vi "Beampointing_BELLA_HTT.vi"() -> ()   [LabVIEW 2020]
uses:
  Shared/GUI_Template/GUI_master/tcp_new_data_event.ctl
  Shared/GUI_Template/GUI_master/tcp new data cluster.ctl
  Ctrs/beam detection.ctl
  GUI_Beampointing_single_TRA/Ctrs/move.ctl
  General GUIs/Device GUIs/GUI_Cameras/Controls/Crosshair type def.ctl
  <vilib>/Utility/file.llb/Read From Spreadsheet File (string).vi
  <userlib>/_OpenG.lib/array/array.llb/Filter 1D Array with Scalar (String)__ogtk.vi
  <vilib>/Utility/file.llb/Write To Spreadsheet File (string).vi
  <vilib>/Analysis/NI_AALBase.lvlib
  <vilib>/vision/NI_Vision_Development_Module.lvlib
panel:
  out "error out 3":errorcluster
  out "error out":errorcluster
  in  "Position.Axis 1::100":dbl caption="Motor Axis 1" min=-3.0 max=13.0 format="%#_6f"
  in  "Position.Axis 2::100":dbl caption="Motor Axis 1" min=-3.0 max=17.0 format="%#_6f"
  in  "GUIdevice 100":string
  out "Array 3":sgl[](array[numeric])=[35.01637, 16.987305, 27.281555, 56.5656, 0.0, 12.310791, 0.0, 0.0, 0.0, 0.0, 0.0, 0.0]
  in  "save path":path=path "W:/BP_DATA"
  out "size(s) 6":i32=12
  out "config path":string
  out "motor refs 7":refnum<vi>[](array[refnum])
  out "Moving Y":string
  out "Moving X":string
  out "particles":T1(array[cluster])=[{"Area"=13625.0, "Number of Holes"=0.0, "Bounding Rect"={"Left"=100.0, "Top"=93.0, "Right"=241.0, "Bottom"=225.0}, "Center of Mass"={"X"=171.3850275229358, "Y"=158.37277064220183}, "Orientation"=31.450434142859965, "Dimensions"={"Width"=141.0, "Height"=132.0}}]
  out "motor refs 6":refnum<vi>[](array[refnum])
  out "millisecond timer value":u32=150056294
  out "motor refs 5":refnum<vi>[](array[refnum])
  out "appended path":path=path "C:/Users/loasis.BELLANET/Documents/000 Labview/Developers Version/Interface/GUI_Beampointing_multi/defaultDevices_PICObooster.txt"
  out "motor refs 4":refnum<vi>[](array[refnum])
  in  "active Axis ref 3":cluster{"Ref X":refnum<vi>, "Ref Y":refnum<vi>}
  out "motor refs 3":refnum<vi>[](array[refnum])
  in  "active man refs":cluster{"Ref X":refnum<vi>, "Ref Y":refnum<vi>}
  out "motor refs 2":refnum<vi>[](array[refnum])
  in  "Numeric":dbl=2.0
  out "Current State":string="Exit"
  in  "output cluster 2":T5 {"detection para"."smal para"."Measurement Parameter" items=["Center of Mass X", "Center of Mass Y", "First Pixel X", "First Pixel Y", "Bounding Rect Left", "Bounding Rect Top", "Bounding Rect Right", "Bounding Rect Bottom", "Max Feret Diameter Start X", "Max Feret Diameter Start Y", "Max Feret Diameter End X", "Max Feret Diameter End Y", "Max Horiz. Segment Length Left", "Max Horiz. Segment Length Right", "Max Horiz. Segment Length Row", "-", "Bounding Rect Width", "Bounding Rect Height", "Bounding Rect Diagonal", "Perimeter", "Convex Hull Perimeter", "Holes' Perimeter", "Max Feret Diameter", "Equivalent Ellipse Major Axis", "Equivalent Ellipse Minor Axis", "Equivalent Ellipse Minor Axis (Feret)", "Equivalent Rect Long Side", "Equivalent Rect Short Side", "Equivalent Rect Diagonal", "Equivalent Rect Short Side (Feret)", "Average Horiz. Segment Length", "Average Vert. Segment Length", "Hydraulic Radius", "Waddel Disk Diameter", "-", "Area", "Holes' Area", "Particle & Holes' Area", "Convex Hull Area", "Image Area", "-", "Number of Holes", "Number of Horiz. Segments", "Number of Vert. Segments", "-", "Orientation", "Max Feret Diameter Orientation", "-", "% Area/Image Area", "% Area/(Particle & Holes' Area)", "Ratio of Equivalent Ellipse Axes", "Ratio of Equivalent Rect Sides", "-", "Elongation Factor", "Compactness Factor", "Heywood Circularity Factor", "Type Factor", "-", "Sum X", "Sum Y", "Sum XX", "Sum XY", "Sum YY", "Sum XXX", "Sum XXY", "Sum XYY", "Sum YYY", "-", "Moment of Inertia XX", "Moment of Inertia XY", "Moment of Inertia YY", "Moment of Inertia XXX", "Moment of Inertia XXY", "Moment of Inertia XYY", "Moment of Inertia YYY", "Norm. Moment of Inertia XX", "Norm. Moment of Inertia XY", "Norm. Moment of Inertia YY", "Norm. Moment of Inertia XXX", "Norm. Moment of Inertia XXY", "Norm. Moment of Inertia XYY", "Norm. Moment of Inertia YYY", "Hu Moment 1", "Hu Moment 2", "Hu Moment 3", "Hu Moment 4", "Hu Moment 5", "Hu Moment 6", "Hu Moment 7"]; "detection para"."smal para"."Range Lower Value" format="%.2f"; "detection para"."smal para"."Range Upper Value" format="%.2f"; "detection para"."detection method" items=["clustering", "entropy", "metric", "moments", "inter-class variance"]; "detection para"."Filter" items=["No Filter", "Median Filter", "Low Pass Filter"]}
  out "CCDs":string[](array[string])=["RegenCam", "BoosterCam", "PreampCam", "Amp1Cam", "Amp2Cam", "Amp3Cam", "", "", "", "", "", ""]
  in  "GUIdevice 12":string
  in  "GUIdevice 11":string
  in  "GUIdevice 10":string
  in  "GUIdevice 9":string
  out "error out 2":errorcluster
  in  "active cams":string[](array[string])
  in  "Motor Y":dbl[][](array[numeric])
  in  "Motor X":dbl[][](array[numeric])
  out "Names":string[](array[string])=["device12", "device45", "", ""]
  in  "Offset X stats":dbl[][](array[numeric])
  in  "Offset Y stats":dbl[][](array[numeric])
  out "Box":T6(array[cluster])=[{"Left"=100.0, "Top"=93.0, "Right"=241.0, "Bottom"=225.0}, {"Left"=87.0, "Top"=22.0, "Right"=220.0, "Bottom"=185.0}, {"Left"=80.0, "Top"=37.0, "Right"=220.0, "Bottom"=176.0}, {"Left"=78.0, "Top"=52.0, "Right"=221.0, "Bottom"=209.0}, {"Left"=0.0, "Top"=0.0, "Right"=0.0, "Bottom"=0.0}]
  in  "Tab Control 2":enum32{"Config ", "Main", "History"}(tab)=enum."Main"
  in  "associated motors":T7={"Motor CCD 1"=0, "Motor CCD 2"=0, "Motor CCD 3"=1, "Motor CCD 4"=0, "Motor CCD 5"=0, "Motor CCD 6"=0, "Motor CCD 7"=0, "Motor CCD 8"=0, "Motor CCD 9"=0, "Motor CCD 10"=0, "Motor CCD 11"=0, "Motor CCD 12"=0} {"Motor CCD 12" items=["device12", "device34", "HeatESP", ""]; "Motor CCD 11" items=["device12", "device34", "HeatESP", ""]; "Motor CCD 10" items=["device12", "device34", "HeatESP", ""]; "Motor CCD 9" items=["device12", "device34", "HeatESP", ""]; "Motor CCD 8" items=["device12", "device34", "HeatESP", ""]; "Motor CCD 7" items=["device12", "device34", "HeatESP", ""]; "Motor CCD 6" items=["device12", "device34", "HeatESP", ""]; "Motor CCD 5" items=["device12", "device34", "HeatESP", ""]; "Motor CCD 4" items=["device12", "device34", "HeatESP", ""]; "Motor CCD 3" items=["device12", "device34", "HeatESP", ""]; "Motor CCD 2" items=["device12", "device34", "HeatESP", ""]; "Motor CCD 1" items=["device12", "device34", "HeatESP", ""]}
  out "Cameras":T8={"[0]"="RegenCam", "[1]"="BoosterCam", "[2]"="PreampCam", "[3]"="Amp1Cam", "[4]"="Amp2Cam", "[5]"="Amp3Cam", "[6]"="", "[7]"="", "[8]"="", "[8] 2"="", "[8] 3"="", "[8] 4"=""}
  out "Status":cluster{i32, i32, "Centroid X":dbl[][]}(graph)={0, 1, "Centroid X"=[[171.87383691112902, 0.0, 0.0], [153.80799798158193, 0.0, 0.0], [147.97157969527117, 0.0, 0.0], [147.97285865350722, 0.0, 0.0], [0.0, 0.0, 0.0], [0.0, 0.0, 0.0], [0.0, 0.0, 0.0], [0.0, 0.0, 0.0], [0.0, 0.0, 0.0], [0.0, 0.0, 0.0], [0.0, 0.0, 0.0], [0.0, 0.0, 0.0]]}
  in  "Exposure:12":dbl=0.095 min=0.0001 max=1.0 format="%#_6f"
  in  "Triggerdelay::12":dbl=0.003 min=0.0 max=0.09 format="%#_6f"
  in  "Exposure::11":dbl=0.095 min=0.0001 max=1.0 format="%#_6f"
  in  "Triggerdelay::11":dbl=0.003 min=0.0 max=0.09 format="%#_6f"
  in  "Exposure::10":dbl=0.095 min=0.0001 max=1.0 format="%#_6f"
  in  "Triggerdelay::10":dbl=0.003 min=0.0 max=0.09 format="%#_6f"
  in  "Exposure::9":dbl=0.095 min=0.0001 max=1.0 format="%#_6f"
  in  "Triggerdelay::9":dbl=0.003 min=0.0 max=0.09 format="%#_6f"
  in  "Trigger::9":bool
  in  "Trigger::10":bool caption="Trigger:10"
  in  "Trigger::11":bool
  in  "Trigger::12":bool
  in  "Target.Y::9":dbl=45.0 caption="T9y" min=0.0 max=2000.0 format="%#_6f"
  in  "Target.X::9":dbl=47.0 caption="Tx9" min=0.0 max=2000.0 format="%#_6f"
  in  "Target.Y::10":dbl=45.0 caption="T10y" min=0.0 max=2000.0 format="%#_6f"
  in  "Target.X::10":dbl=47.0 caption="T10x" min=0.0 max=2000.0 format="%#_6f"
  in  "Target.Y::11":dbl=45.0 caption="T11y" min=0.0 max=2000.0 format="%#_6f"
  in  "Target.X::11":dbl=47.0 caption="T11x" min=0.0 max=2000.0 format="%#_6f"
  in  "Target.Y::12":dbl=45.0 caption="T12y" min=0.0 max=2000.0 format="%#_6f"
  in  "Target.X::12":dbl=47.0 caption="T12x" min=0.0 max=2000.0 format="%#_6f"
  in  "Exposure::8":dbl=0.095 min=0.0001 max=1.0 format="%#_6f"
  in  "Triggerdelay::8":dbl=0.003 min=0.0 max=0.09 format="%#_6f"
  in  "Trigger::8":bool
  in  "Target.Y::8":dbl=45.0 caption="T8y" min=0.0 max=2000.0 format="%#_6f"
  in  "Target.X::8":dbl=47.0 caption="T8x" min=0.0 max=2000.0 format="%#_6f"
  in  "Target.Y::7":dbl=45.0 caption="T7x" min=0.0 max=2000.0 format="%#_6f"
  in  "Target.X::7":dbl=47.0 caption="T7y" min=0.0 max=2000.0 format="%#_6f"
  in  "Target.Y::6":dbl=142.0 caption="T6y" min=0.0 max=5000.0 format="%#_6f"
  in  "Target.X::6":dbl=123.0 caption="T6x" min=0.0 max=5000.0 format="%#_6f"
  in  "Target.Y::5":dbl=108.0 caption="T5y" min=0.0 max=2000.0 format="%#_6f"
  in  "Target.X::5":dbl=172.0 caption="T5x" min=0.0 max=2000.0 format="%#_6f"
  in  "Target.Y::4":dbl=130.0 caption="T4y" min=0.0 max=2000.0 format="%#_6f"
  in  "Target.X::4":dbl=148.0 caption="T4x" min=0.0 max=2000.0 format="%#_6f"
  in  "Target.Y::3":dbl=110.0 caption="T3y" min=0.0 max=2000.0 format="%#_6f"
  in  "Target.X::3":dbl=154.0 caption="T3x" min=0.0 max=2000.0 format="%#_6f"
  in  "Target.Y::2":dbl=106.0 caption="T2y" min=0.0 max=2000.0 format="%#_6f"
  in  "Target.X::2":dbl=163.0 caption="T2x" min=0.0 max=2000.0 format="%#_6f"
  in  "Target.Y::1":dbl=162.0 caption="T1y" min=0.0 max=2000.0 format="%#_6f"
  in  "Target.X::1":dbl=171.0 caption="T1x" min=0.0 max=2000.0 format="%#_6f"
  in  "Exposure::7":dbl=0.095 min=3.8e-05 max=1.0 format="%#_6f"
  in  "Triggerdelay::7":dbl=0.003 min=0.0 max=0.09 format="%#_6f"
  in  "Trigger::7":bool
  in  "Exposure::6":dbl=0.095 min=3.8e-05 max=1.0 format="%#_6f"
  in  "Triggerdelay::6":dbl=0.003 min=0.0 max=0.09 format="%#_6f"
  in  "Trigger::6":bool
  in  "Exposure::5":dbl=0.095 min=3.8e-05 max=1.0 format="%#_6f"
  in  "Triggerdelay::5":dbl=0.003 min=0.0 max=0.09 format="%#_6f"
  in  "Trigger::5":bool
  in  "Exposure::4":dbl=0.095 min=3.8e-05 max=1.0 format="%#_6f"
  in  "Triggerdelay::4":dbl=0.003 min=0.0 max=0.09 format="%#_6f"
  in  "Trigger::4":bool
  in  "Exposure::3":dbl=0.095 min=3.8e-05 max=1.0 format="%#_6f"
  in  "Triggerdelay::3":dbl=0.003 min=0.0 max=0.09 format="%#_6f"
  in  "Trigger::3":bool
  in  "Exposure::2":dbl=0.095 min=0.0 max=1.0 format="%#_6f"
  in  "Triggerdelay::2":dbl=0.003 min=0.0 max=1.0 format="%#_6f"
  in  "Trigger::2":bool
  out "image::1":T9(plugin-control) caption="BellaCam32_3"
  out "image::2":T9(plugin-control) caption="BellaCam46_2_Scatter_In_1"
  out "image::3":T9(plugin-control)
  out "image::4":T9(plugin-control)
  out "image::5":T9(plugin-control)
  out "image::6":T9(plugin-control)
  out "image::7":T9(plugin-control)
  out "image::8":T9(plugin-control)
  in  "Exposure::1":dbl=0.095 min=0.0001 max=1000001.0 format="%#_6f"
  in  "Triggerdelay::1":dbl=0.003 min=0.0 max=100000.0 format="%#_6f"
  in  "Trigger::1":bool
  in  "UDP error message":string
  out "required Y":bool[](array[boolean])=[FALSE, TRUE, FALSE, FALSE, FALSE]
  out "required X":bool[](array[boolean])=[FALSE, TRUE, FALSE, FALSE, FALSE]
  out "detected":bool[](array[boolean])=[TRUE, TRUE, TRUE, TRUE, FALSE]
  out "name array":string[](array[string])=["RegenCam", "BoosterCam", "PreampCam", "Amp1Cam", "Amp3Cam"]
  out "image::9":T9(plugin-control)
  out "image::10":T9(plugin-control)
  out "image::11":T9(plugin-control)
  out "image::12":T9(plugin-control)
  out "speedmode X":bool[](array[boolean])=[TRUE, TRUE, TRUE, TRUE, FALSE]
  out "speedmode Y":bool[](array[boolean])=[TRUE, FALSE, TRUE, TRUE, FALSE]
  out "CCD 9":cluster{timestamp[], dbl[]}[](graph)=[{[timestamp(3549547983.3591223 s since 1904-01-01)], [0.0]}, {[timestamp(3549547983.3591223 s since 1904-01-01)], [0.0]}, {[timestamp(3549547983.3591223 s since 1904-01-01)], [20.0]}, {[timestamp(3549547983.3591223 s since 1904-01-01)], [-20.0, -20.0, -20.0, -20.0]}]
  out "CCD 10":cluster{timestamp[], dbl[]}[](graph)=[{[timestamp(3549547983.360123 s since 1904-01-01)], [0.0]}, {[timestamp(3549547983.360123 s since 1904-01-01)], [0.0]}, {[timestamp(3549547983.360123 s since 1904-01-01)], [20.0]}, {[timestamp(3549547983.360123 s since 1904-01-01)], [-20.0, -20.0, -20.0, -20.0]}]
  out "CCD 11":cluster{timestamp[], dbl[]}[](graph)=[{[timestamp(3549547983.360123 s since 1904-01-01)], [0.0]}, {[timestamp(3549547983.360123 s since 1904-01-01)], [0.0]}, {[timestamp(3549547983.360123 s since 1904-01-01)], [20.0]}, {[timestamp(3549547983.360123 s since 1904-01-01)], [-20.0, -20.0, -20.0, -20.0]}]
  out "CCD 12":cluster{timestamp[], dbl[]}[](graph)=[{[timestamp(3549547983.360123 s since 1904-01-01)], [0.0]}, {[timestamp(3549547983.360123 s since 1904-01-01)], [0.0]}, {[timestamp(3549547983.360123 s since 1904-01-01)], [20.0]}, {[timestamp(3549547983.360123 s since 1904-01-01)], [-20.0, -20.0, -20.0, -20.0]}]
  out "CCD 5":cluster{timestamp[], dbl[]}[](graph)=[{[timestamp(3549547983.358122 s since 1904-01-01)], [0.0]}, {[timestamp(3549547983.358122 s since 1904-01-01)], [0.0]}, {[timestamp(3549547983.358122 s since 1904-01-01)], [20.0]}, {[timestamp(3549547983.358122 s since 1904-01-01)], [-20.0, -20.0, -20.0, -20.0]}]
  out "CCD 6":cluster{timestamp[], dbl[]}[](graph)=[{[timestamp(3549547983.3591223 s since 1904-01-01)], [0.0]}, {[timestamp(3549547983.3591223 s since 1904-01-01)], [0.0]}, {[timestamp(3549547983.3591223 s since 1904-01-01)], [20.0]}, {[timestamp(3549547983.3591223 s since 1904-01-01)], [-20.0, -20.0, -20.0, -20.0]}]
  out "CCD 7":cluster{timestamp[], dbl[]}[](graph)=[{[timestamp(3549547983.3591223 s since 1904-01-01)], [0.0]}, {[timestamp(3549547983.3591223 s since 1904-01-01)], [0.0]}, {[timestamp(3549547983.3591223 s since 1904-01-01)], [20.0]}, {[timestamp(3549547983.3591223 s since 1904-01-01)], [-20.0, -20.0, -20.0, -20.0]}]
  out "CCD 8":cluster{timestamp[], dbl[]}[](graph)=[{[timestamp(3549547983.3591223 s since 1904-01-01)], [0.0]}, {[timestamp(3549547983.3591223 s since 1904-01-01)], [0.0]}, {[timestamp(3549547983.3591223 s since 1904-01-01)], [20.0]}, {[timestamp(3549547983.3591223 s since 1904-01-01)], [-20.0, -20.0, -20.0, -20.0]}]
  out "CCD 2":cluster{timestamp[], dbl[]}[](graph)=[{[timestamp(3549547983.358122 s since 1904-01-01)], [3.0783937413765585]}, {[timestamp(3549547983.358122 s since 1904-01-01)], [8.883046862591215]}, {[timestamp(3549547983.358122 s since 1904-01-01)], [20.0]}, {[timestamp(3549547983.358122 s since 1904-01-01)], [-20.0, -20.0, -20.0, -20.0]}]
  out "CCD 1":cluster{timestamp[], dbl[]}[](graph)=[{[timestamp(3549547983.357121 s since 1904-01-01)], [3.1654865062995725]}, {[timestamp(3549547983.357121 s since 1904-01-01)], [-0.42630614615123363]}, {[timestamp(3549547983.357121 s since 1904-01-01)], [20.0]}, {[timestamp(3549547983.357121 s since 1904-01-01)], [-20.0, -20.0, -20.0, -20.0]}]
  out "CCD 3":cluster{timestamp[], dbl[]}[](graph)=[{[timestamp(3549547983.358122 s since 1904-01-01)], [5.607599326451648]}, {[timestamp(3549547983.358122 s since 1904-01-01)], [4.73033759911138]}, {[timestamp(3549547983.358122 s since 1904-01-01)], [0.0]}, {[timestamp(3549547983.358122 s since 1904-01-01)], [0.0, 0.0, 0.0, 0.0]}]
  out "CCD 4":cluster{timestamp[], dbl[]}[](graph)=[{[timestamp(3549547983.358122 s since 1904-01-01)], [1.2734976836249814]}, {[timestamp(3549547983.358122 s since 1904-01-01)], [-0.6350086940318818]}, {[timestamp(3549547983.358122 s since 1904-01-01)], [20.0]}, {[timestamp(3549547983.358122 s since 1904-01-01)], [-20.0, -20.0, -20.0, -20.0]}]
  in  "History Size":i32=2000
  out "History Index":i32=1
  in  "Feedback Global":bool
  in  "detection para":T3[](array[typedef])=[{"Filter"=1, "Filter Para"={"X Size"=5, "Y Size"=5, "% Tolerance"=1}, "detection method"=4, "smal para"=[{"Measurement Parameter"=35, "Range Lower Value"=0.0, "Range Upper Value"=0.0, "Range"=TRUE, "Measurement Type"=FALSE}], "Remove small Objects"=TRUE, "Restrict to round Objects"=FALSE}, {"Filter"=1, "Filter Para"={"X Size"=5, "Y Size"=5, "% Tolerance"=1}, "detection method"=4, "smal para"=[{"Measurement Parameter"=35, "Range Lower Value"=0.0, "Range Upper Value"=500.0, "Range"=FALSE, "Measurement Type"=FALSE}], "Remove small Objects"=TRUE, "Restrict to round Objects"=FALSE}, {"Filter"=1, "Filter Para"={"X Size"=5, "Y Size"=5, "% Tolerance"=1}, "detection method"=4, "smal para"=[{"Measurement Parameter"=35, "Range Lower Value"=0.0, "Range Upper Value"=500.0, "Range"=TRUE, "Measurement Type"=FALSE}], "Remove small Objects"=TRUE, "Restrict to round Objects"=FALSE}, {"Filter"=1, "Filter Para"={"X Size"=5, "Y Size"=5, "% Tolerance"=1}, "detection method"=4, "smal para"=[{"Measurement Parameter"=35, "Range Lower Value"=0.0, "Range Upper Value"=500.0, "Range"=TRUE, "Measurement Type"=FALSE}], "Remove small Objects"=TRUE, "Restrict to round Objects"=FALSE}, {"Filter"=1, "Filter Para"={"X Size"=5, "Y Size"=5, "% Tolerance"=1}, "detection method"=4, "smal para"=[{"Measurement Parameter"=35, "Range Lower Value"=0.0, "Range Upper Value"=500.0, "Range"=TRUE, "Measurement Type"=FALSE}], "Remove small Objects"=TRUE, "Restrict to round Objects"=FALSE}, {"Filter"=1, "Filter Para"={"X Size"=5, "Y Size"=5, "% Tolerance"=1}, "detection method"=4, "smal para"=[{"Measurement Parameter"=35, "Range Lower Value"=0.0, "Range Upper Value"=500.0, "Range"=TRUE, "Measurement Type"=FALSE}], "Remove small Objects"=TRUE, "Restrict to round Objects"=FALSE}, {"Filter"=1, "Filter Para"={"X Size"=5, "Y Size"=5, "% Tolerance"=1}, "detection method"=4, "smal para"=[{"Measurement Parameter"=35, "Range Lower Value"=0.0, "Range Upper Value"=500.0, "Range"=TRUE, "Measurement Type"=FALSE}], "Remove small Objects"=TRUE, "Restrict to round Objects"=FALSE}, {"Filter"=1, "Filter Para"={"X Size"=5, "Y Size"=5, "% Tolerance"=1}, "detection method"=3, "smal para"=[{"Measurement Parameter"=35, "Range Lower Value"=0.0, "Range Upper Value"=0.0, "Range"=FALSE, "Measurement Type"=FALSE}], "Remove small Objects"=TRUE, "Restrict to round Objects"=FALSE}, {"Filter"=1, "Filter Para"={"X Size"=5, "Y Size"=5, "% Tolerance"=1}, "detection method"=4, "smal para"=[{"Measurement Parameter"=35, "Range Lower Value"=0.0, "Range Upper Value"=0.0, "Range"=FALSE, "Measurement Type"=FALSE}], "Remove small Objects"=TRUE, "Restrict to round Objects"=FALSE}, {"Filter"=1, "Filter Para"={"X Size"=5, "Y Size"=5, "% Tolerance"=1}, "detection method"=4, "smal para"=[{"Measurement Parameter"=35, "Range Lower Value"=0.0, "Range Upper Value"=500.0, "Range"=TRUE, "Measurement Type"=FALSE}], "Remove small Objects"=TRUE, "Restrict to round Objects"=FALSE}, {"Filter"=1, "Filter Para"={"X Size"=5, "Y Size"=5, "% Tolerance"=1}, "detection method"=4, "smal para"=[{"Measurement Parameter"=35, "Range Lower Value"=0.0, "Range Upper Value"=500.0, "Range"=TRUE, "Measurement Type"=FALSE}], "Remove small Objects"=TRUE, "Restrict to round Objects"=FALSE}, {"Filter"=1, "Filter Para"={"X Size"=5, "Y Size"=5, "% Tolerance"=1}, "detection method"=4, "smal para"=[{"Measurement Parameter"=35, "Range Lower Value"=0.0, "Range Upper Value"=500.0, "Range"=TRUE, "Measurement Type"=FALSE}], "Remove small Objects"=TRUE, "Restrict to round Objects"=FALSE}] {"smal para"."Measurement Parameter" items=["Center of Mass X", "Center of Mass Y", "First Pixel X", "First Pixel Y", "Bounding Rect Left", "Bounding Rect Top", "Bounding Rect Right", "Bounding Rect Bottom", "Max Feret Diameter Start X", "Max Feret Diameter Start Y", "Max Feret Diameter End X", "Max Feret Diameter End Y", "Max Horiz. Segment Length Left", "Max Horiz. Segment Length Right", "Max Horiz. Segment Length Row", "-", "Bounding Rect Width", "Bounding Rect Height", "Bounding Rect Diagonal", "Perimeter", "Convex Hull Perimeter", "Holes' Perimeter", "Max Feret Diameter", "Equivalent Ellipse Major Axis", "Equivalent Ellipse Minor Axis", "Equivalent Ellipse Minor Axis (Feret)", "Equivalent Rect Long Side", "Equivalent Rect Short Side", "Equivalent Rect Diagonal", "Equivalent Rect Short Side (Feret)", "Average Horiz. Segment Length", "Average Vert. Segment Length", "Hydraulic Radius", "Waddel Disk Diameter", "-", "Area", "Holes' Area", "Particle & Holes' Area", "Convex Hull Area", "Image Area", "-", "Number of Holes", "Number of Horiz. Segments", "Number of Vert. Segments", "-", "Orientation", "Max Feret Diameter Orientation", "-", "% Area/Image Area", "% Area/(Particle & Holes' Area)", "Ratio of Equivalent Ellipse Axes", "Ratio of Equivalent Rect Sides", "-", "Elongation Factor", "Compactness Factor", "Heywood Circularity Factor", "Type Factor", "-", "Sum X", "Sum Y", "Sum XX", "Sum XY", "Sum YY", "Sum XXX", "Sum XXY", "Sum XYY", "Sum YYY", "-", "Moment of Inertia XX", "Moment of Inertia XY", "Moment of Inertia YY", "Moment of Inertia XXX", "Moment of Inertia XXY", "Moment of Inertia XYY", "Moment of Inertia YYY", "Norm. Moment of Inertia XX", "Norm. Moment of Inertia XY", "Norm. Moment of Inertia YY", "Norm. Moment of Inertia XXX", "Norm. Moment of Inertia XXY", "Norm. Moment of Inertia XYY", "Norm. Moment of Inertia YYY", "Hu Moment 1", "Hu Moment 2", "Hu Moment 3", "Hu Moment 4", "Hu Moment 5", "Hu Moment 6", "Hu Moment 7"]; "smal para"."Range Lower Value" format="%.2f"; "smal para"."Range Upper Value" format="%.2f"; "detection method" items=["clustering", "entropy", "metric", "moments", "inter-class variance"]; "Filter" items=["No Filter", "Median Filter", "Low Pass Filter"]}
  in  "GUIdevice 8":string
  in  "Tab Control":T10(tab)
  in  "new tdms":bool
  in  "Save Stats":bool
  in  "Save Config":bool
  in  "Load Config":bool
  in  "update speed [ms]":i32=1000
  in  "img to avg":i32=6 min=3 max=200
  in  "Reset History":bool
  in  "autodetect":bool
  in  "Detection Rate":dbl=0.8 min=0.001 max=1.0
  in  "Center":bool
  in  "Align":bool
  in  "Speedmode @":dbl=5.0 min=1.0 max=20.0
  in  "device ini":bool
  in  "beam detection para":T3={"Filter"=1, "Filter Para"={"X Size"=5, "Y Size"=5, "% Tolerance"=1}, "detection method"=4, "smal para"=[{"Measurement Parameter"=35, "Range Lower Value"=0.0, "Range Upper Value"=500.0, "Range"=FALSE, "Measurement Type"=FALSE}], "Remove small Objects"=TRUE, "Restrict to round Objects"=FALSE} {"smal para"."Measurement Parameter" items=["Center of Mass X", "Center of Mass Y", "First Pixel X", "First Pixel Y", "Bounding Rect Left", "Bounding Rect Top", "Bounding Rect Right", "Bounding Rect Bottom", "Max Feret Diameter Start X", "Max Feret Diameter Start Y", "Max Feret Diameter End X", "Max Feret Diameter End Y", "Max Horiz. Segment Length Left", "Max Horiz. Segment Length Right", "Max Horiz. Segment Length Row", "-", "Bounding Rect Width", "Bounding Rect Height", "Bounding Rect Diagonal", "Perimeter", "Convex Hull Perimeter", "Holes' Perimeter", "Max Feret Diameter", "Equivalent Ellipse Major Axis", "Equivalent Ellipse Minor Axis", "Equivalent Ellipse Minor Axis (Feret)", "Equivalent Rect Long Side", "Equivalent Rect Short Side", "Equivalent Rect Diagonal", "Equivalent Rect Short Side (Feret)", "Average Horiz. Segment Length", "Average Vert. Segment Length", "Hydraulic Radius", "Waddel Disk Diameter", "-", "Area", "Holes' Area", "Particle & Holes' Area", "Convex Hull Area", "Image Area", "-", "Number of Holes", "Number of Horiz. Segments", "Number of Vert. Segments", "-", "Orientation", "Max Feret Diameter Orientation", "-", "% Area/Image Area", "% Area/(Particle & Holes' Area)", "Ratio of Equivalent Ellipse Axes", "Ratio of Equivalent Rect Sides", "-", "Elongation Factor", "Compactness Factor", "Heywood Circularity Factor", "Type Factor", "-", "Sum X", "Sum Y", "Sum XX", "Sum XY", "Sum YY", "Sum XXX", "Sum XXY", "Sum XYY", "Sum YYY", "-", "Moment of Inertia XX", "Moment of Inertia XY", "Moment of Inertia YY", "Moment of Inertia XXX", "Moment of Inertia XXY", "Moment of Inertia XYY", "Moment of Inertia YYY", "Norm. Moment of Inertia XX", "Norm. Moment of Inertia XY", "Norm. Moment of Inertia YY", "Norm. Moment of Inertia XXX", "Norm. Moment of Inertia XXY", "Norm. Moment of Inertia XYY", "Norm. Moment of Inertia YYY", "Hu Moment 1", "Hu Moment 2", "Hu Moment 3", "Hu Moment 4", "Hu Moment 5", "Hu Moment 6", "Hu Moment 7"]; "smal para"."Range Lower Value" format="%.2f"; "smal para"."Range Upper Value" format="%.2f"; "detection method" items=["clustering", "entropy", "metric", "moments", "inter-class variance"]; "Filter" items=["No Filter", "Median Filter", "Low Pass Filter"]}
  in  "move config":T2={"Tolerance [%]"=0.1, "Stepsize"=0.0001, "Invert Axis"=TRUE, "Invert Direction X"=FALSE, "Invert Direction Y"=TRUE, "enable feedback"=FALSE, "Set Centriod Target"=FALSE}
  in  "Position 2":dbl=-20.0 caption="Stepsize" min=0.0 max=999999.0 format="%_6f"
  in  "Position 1":dbl=20.0 caption="Stepsize" min=0.0 max=999999.0 format="%_6f"
  in  "Right":bool caption="RelativeMove.Axis 1.CCW::1"
  in  "Left":bool caption="RelativeMove.Axis 1.CW::1"
  in  "Down":bool caption="RelativeMove.Axis. 2.CCW::1"
  in  "Up":bool caption="RelativeMove.Axis 2.CW::1"
  in  "StepSize":dbl=5.0 caption="Stepsize" min=0.0 max=500.0 format="%#.4f"
  in  "active axis refs 2":T11(array[cluster])
  in  "active Axis ref":cluster{"Ref X":refnum<vi>, "Ref Y":refnum<vi>}
  in  "CCDs":u16(ring) items=["BellaCam32_3", "BellaCam46_2_Scatter_In_1", "", "", "", "", "", "", "", "", "", ""]
  out "motor refs":refnum<vi>[](array[refnum])
  in  "Position.Axis 3::99":dbl caption="Motor Axis 1" min=-5000.0 max=5000.0
  in  "Position.Axis 4::99":dbl caption="Motor Axis 1" min=-5000.0 max=5000.0
  in  "Position.Axis 2::99":dbl=-20.0 caption="Motor Axis 1" min=-5000.0 max=5000.0
  in  "Position.Axis 1::99":dbl=20.0 caption="Motor Axis 1" min=-5000.0 max=5000.0
  in  "GUIdevice 99":string="PicoPad_LCave"
  in  "move properties":T2[](array[typedef])=[{"Tolerance [%]"=0.1, "Stepsize"=0.0001, "Invert Axis"=TRUE, "Invert Direction X"=FALSE, "Invert Direction Y"=TRUE, "enable feedback"=FALSE, "Set Centriod Target"=FALSE}, {"Tolerance [%]"=0.1, "Stepsize"=0.0001, "Invert Axis"=TRUE, "Invert Direction X"=FALSE, "Invert Direction Y"=TRUE, "enable feedback"=FALSE, "Set Centriod Target"=FALSE}, {"Tolerance [%]"=0.1, "Stepsize"=0.0001, "Invert Axis"=TRUE, "Invert Direction X"=FALSE, "Invert Direction Y"=TRUE, "enable feedback"=FALSE, "Set Centriod Target"=FALSE}, {"Tolerance [%]"=0.1, "Stepsize"=0.0001, "Invert Axis"=TRUE, "Invert Direction X"=FALSE, "Invert Direction Y"=TRUE, "enable feedback"=FALSE, "Set Centriod Target"=FALSE}, {"Tolerance [%]"=0.1, "Stepsize"=0.0001, "Invert Axis"=TRUE, "Invert Direction X"=FALSE, "Invert Direction Y"=TRUE, "enable feedback"=FALSE, "Set Centriod Target"=FALSE}, {"Tolerance [%]"=0.1, "Stepsize"=0.0001, "Invert Axis"=TRUE, "Invert Direction X"=FALSE, "Invert Direction Y"=TRUE, "enable feedback"=FALSE, "Set Centriod Target"=FALSE}, {"Tolerance [%]"=0.1, "Stepsize"=0.0001, "Invert Axis"=TRUE, "Invert Direction X"=FALSE, "Invert Direction Y"=TRUE, "enable feedback"=FALSE, "Set Centriod Target"=FALSE}, {"Tolerance [%]"=0.1, "Stepsize"=0.0001, "Invert Axis"=TRUE, "Invert Direction X"=FALSE, "Invert Direction Y"=TRUE, "enable feedback"=FALSE, "Set Centriod Target"=FALSE}, {"Tolerance [%]"=0.1, "Stepsize"=0.0001, "Invert Axis"=TRUE, "Invert Direction X"=FALSE, "Invert Direction Y"=TRUE, "enable feedback"=FALSE, "Set Centriod Target"=FALSE}, {"Tolerance [%]"=0.1, "Stepsize"=0.0001, "Invert Axis"=TRUE, "Invert Direction X"=FALSE, "Invert Direction Y"=TRUE, "enable feedback"=FALSE, "Set Centriod Target"=FALSE}, {"Tolerance [%]"=0.1, "Stepsize"=0.0001, "Invert Axis"=TRUE, "Invert Direction X"=FALSE, "Invert Direction Y"=TRUE, "enable feedback"=FALSE, "Set Centriod Target"=FALSE}, {"Tolerance [%]"=0.1, "Stepsize"=0.0001, "Invert Axis"=TRUE, "Invert Direction X"=FALSE, "Invert Direction Y"=TRUE, "enable feedback"=FALSE, "Set Centriod Target"=FALSE}, {"Tolerance [%]"=0.1, "Stepsize"=0.0001, "Invert Axis"=TRUE, "Invert Direction X"=FALSE, "Invert Direction Y"=TRUE, "enable feedback"=FALSE, "Set Centriod Target"=FALSE}]
  in  "Time":timestamp[][](array[timestamp])
  in  "Mean Size":dbl[][](array[numeric])
  in  "Size":dbl[][](array[numeric])
  in  "active CCDs":i32(listbox)=-1
  in  "Offset Y":dbl[][](array[numeric])
  in  "Offset X":dbl[][](array[numeric])
  in  "Mean Centroid X":dbl[][](array[numeric])
  in  "Mean Centroid Y":dbl[][](array[numeric])
  in  "Centroid Y":dbl[][](array[numeric])
  in  "Centroid X":dbl[][](array[numeric])
  in  "GUIdevice 7":string
  in  "GUIdevice 6":string="Amp3Cam"
  in  "GUIdevice 5":string="Amp2Cam"
  in  "GUIdevice 4":string="Amp1Cam"
  in  "GUIdevice 3":string="PreampCam"
  in  "GUIdevice 2":string="BoosterCam"
  in  "insert tag":bool=TRUE
  in  "stop":bool
  in  "GUIdevice 1":string="RegenCam"
  out "tcp data event":T12
  out "error IO 2":errorcluster
  # "x [Tolerance]"
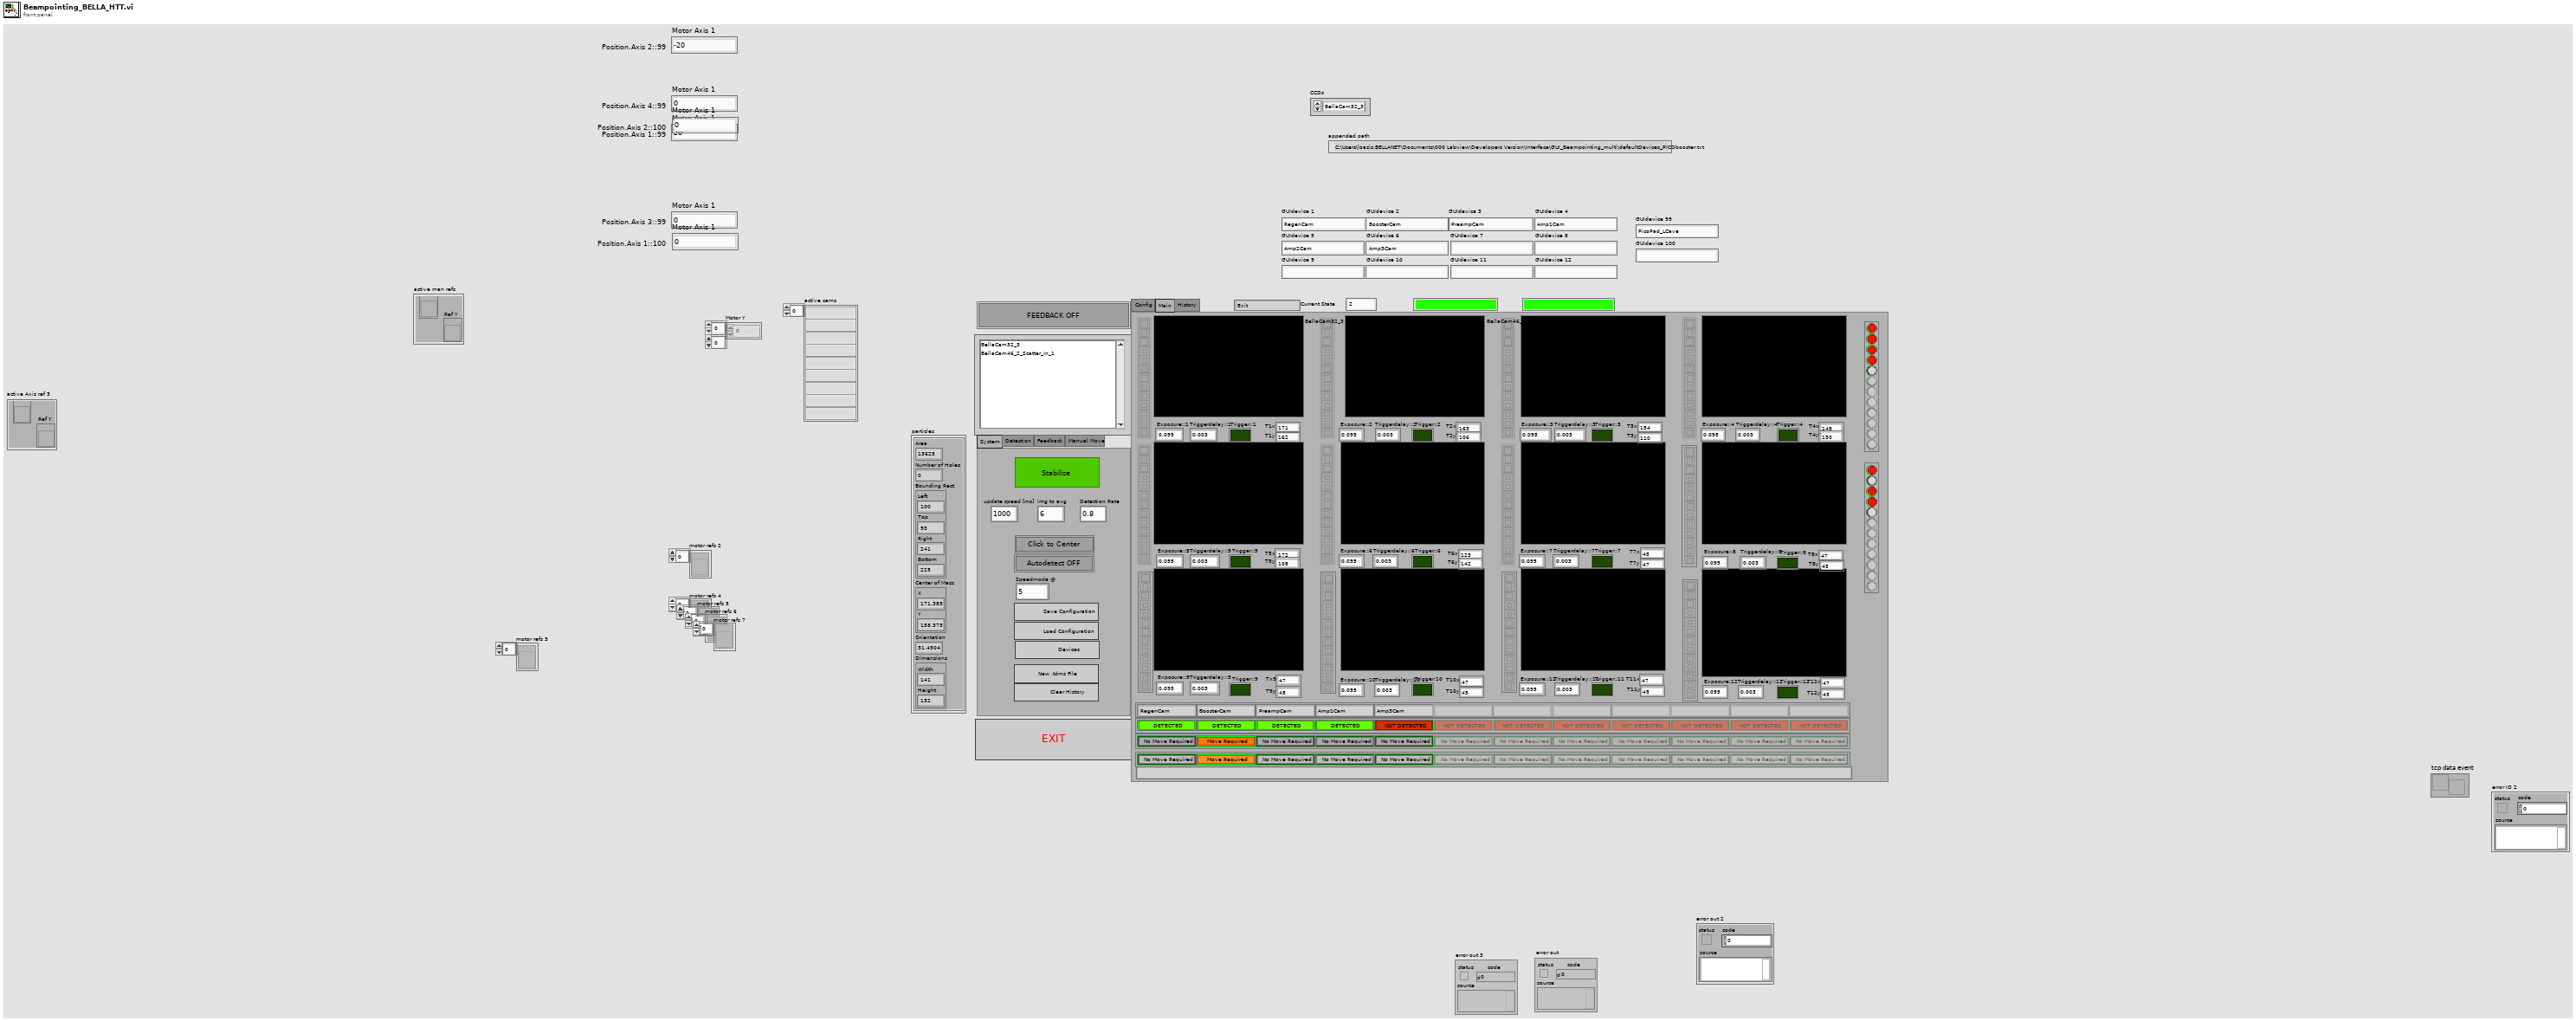
[diagram p1: front panel]
types:
  T1 = cluster{"Area":dbl, "Number of Holes":dbl, "Bounding Rect":cluster{"Left":dbl, "Top":dbl, "Right":dbl, "Bottom":dbl}, "Center of Mass":cluster{"X":dbl, "Y":dbl}, "Orientation":dbl, "Dimensions":cluster{"Width":dbl, "Height":dbl}}[]
  T2 = typedef "move.ctl" = cluster{"Tolerance [%]":dbl, "Stepsize":dbl, "Invert Axis":bool, "Invert Direction X":bool, "Invert Direction Y":bool, "enable feedback":bool, "Set Centriod Target":bool}
  T3 = typedef "beam detection.ctl" = cluster{"Filter":u16, "Filter Para":cluster{"X Size":i32, "Y Size":i32, "% Tolerance":i32}, "detection method":i32, "smal para":cluster{"Measurement Parameter":T4, "Range Lower Value":dbl, "Range Upper Value":dbl, "Range":bool, "Measurement Type":bool}[], "Remove small Objects":bool, "Restrict to round Objects":bool}
  T4 = typedef "Particle Parameters" = i32
  T5 = cluster{"CCDs":string[], "move properties":T2[], "detection para":T3[], "thresholds":cluster{"Lower value":sgl, "Upper value":sgl}[], "Value":cluster{"Motor CCD 1":u16, "Motor CCD 2":u16, "Motor CCD 3":u16, "Motor CCD 4":u16, "Motor CCD 5":u16, "Motor CCD 6":u16, "Motor CCD 7":u16, "Motor CCD 8":u16, "Motor CCD 9":u16, "Motor CCD 10":u16, "Motor CCD 11":u16, "Motor CCD 12":u16}}
  T6 = cluster{"Left":dbl, "Top":dbl, "Right":dbl, "Bottom":dbl}[]
  T7 = cluster{"Motor CCD 1":u16, "Motor CCD 2":u16, "Motor CCD 3":u16, "Motor CCD 4":u16, "Motor CCD 5":u16, "Motor CCD 6":u16, "Motor CCD 7":u16, "Motor CCD 8":u16, "Motor CCD 9":u16, "Motor CCD 10":u16, "Motor CCD 11":u16, "Motor CCD 12":u16}
  T8 = cluster{"[0]":string, "[1]":string, "[2]":string, "[3]":string, "[4]":string, "[5]":string, "[6]":string, "[7]":string, "[8]":string, "[8] 2":string, "[8] 3":string, "[8] 4":string}
  T9 = typedef "IMAQ Image.ctl" = refnum<image>
  T10 = enum32{"System", "Detection", "Feedback", "Manual Move"}
  T11 = cluster{"Ref X":refnum<vi>, "Ref Y":refnum<vi>}[]
  T12 = typedef "tcp_new_data_event.ctl" = refnum<user-event>
  T13 = typedef "tcp new data cluster.ctl" = cluster{"EventEnum":enum16{"new data", "connection status update"}, "Device name":string}
  T14 = typedef "Crosshair type def.ctl" = cluster{"Draw":bool, "Target":cluster{"x":dbl, "y":dbl}, "Size":cluster{"x":dbl, "y":dbl}, "Angle":dbl, "Color":u32, "Thickness":u8, "CrosshairLabel":string}
  T15 = cluster{"Left":i32, "Top":i32, "Right":i32, "Bottom":i32}
  T16 = enum32{"invalid app kind", "Development System", "Run Time System", "Student Edition", "Embedded LabVIEW", "Evaluation", "Custom"}
  T17 = enum16{"open", "open or create", "create or replace", "create", "open (read-only)"}
  T18 = enum32{"Invalid", "Standard", "Closed", "Hidden", "Minimized", "Maximized"}
  T19 = enum16{"open", "replace", "create", "open or create", "replace or create", "replace or create with confirmation"}
  T20 = enum8{"Enabled", "Disabled", "Disabled and Grayed Out"}
  T21 = typedef "Image Type" = u32
  T22 = cluster{"[0]":string, "[1]":string, "[2]":string, "[3]":string, "[4]":string, "[5]":string, "[6]":string, "[7]":string, "[8]":string, "[9]":string, "[10]":string, "[11]":string}
  T23 = cluster{"Target.X::1":refnum<vi>, "Target.Y::1":refnum<vi>}
  T24 = cluster{"Target.X::2":refnum<vi>, "Target.Y::2":refnum<vi>}
  T25 = cluster{"Target.X::3":refnum<vi>, "Target.Y::3":refnum<vi>}
  T26 = cluster{"Target.X::4":refnum<vi>, "Target.Y::4":refnum<vi>}
  T27 = cluster{"Target.X::5":refnum<vi>, "Target.Y::5":refnum<vi>}
  T28 = cluster{"Target.X::6":refnum<vi>, "Target.Y::6":refnum<vi>}
  T29 = cluster{"Target.X::7":refnum<vi>, "Target.Y::7":refnum<vi>}
  T30 = cluster{"Target.X::8":refnum<vi>, "Target.Y::8":refnum<vi>}
  T31 = cluster{"Target.X::12":refnum<vi>, "Target.Y::12":refnum<vi>}
  T32 = cluster{"Target.X::9":refnum<vi>, "Target.Y::9":refnum<vi>}
  T33 = cluster{"Target.X::10":refnum<vi>, "Target.Y::10":refnum<vi>}
  T34 = cluster{"Target.X::11":refnum<vi>, "Target.Y::11":refnum<vi>}
  T35 = cluster{"Target.X::12":refnum<vi>, "Target.Y::12":refnum<vi>}[]
  T36 = cluster{"Left":dbl, "Top":dbl, "Right":dbl, "Bottom":dbl}
  T37 = cluster{"Core":cluster{"Current VI Reference":refnum<vi>, "Close Panel on Exit?":bool}, "detection para":T3[], "thresholds":cluster{"Lower value":sgl, "Upper value":sgl}[], "Centroid X":dbl[][], "Centroid Y":dbl[][], "img to avg":i32, "Mean Centroid X":dbl[][], "Mean Centroid Y":dbl[][], "Offset X":dbl[][], "Offset Y":dbl[][], "Offset X stats ":dbl[][], "Offset Y stats ":dbl[][], "Size":dbl[][], "Mean Size":dbl[][], "Time":timestamp[][], "move properties":T2[], "active axis refs 2":cluster{"Ref X":refnum<vi>, "Ref Y":refnum<vi>}[], "active ccd":i32, "Feedback global":bool, "Motor X":dbl[][], "Motor Y":dbl[][], "active cams":string[], "Data Value Reference out":refnum<k34>, "active man refs":cluster{"Ref X":refnum<vi>, "Ref Y":refnum<vi>}, "detected":bool[], "speedmode X":bool[], "speedmode Y":bool[], "steps speed X":dbl[], "steps speed Y":dbl[]}
  T38 = cluster{"Current VI Reference":refnum<vi>, "Close Panel on Exit?":bool}
  T39 = cluster{"appended array":timestamp[], "appended array":dbl[]}
  T40 = cluster{"appended array":timestamp[], "appended array":dbl[]}[]
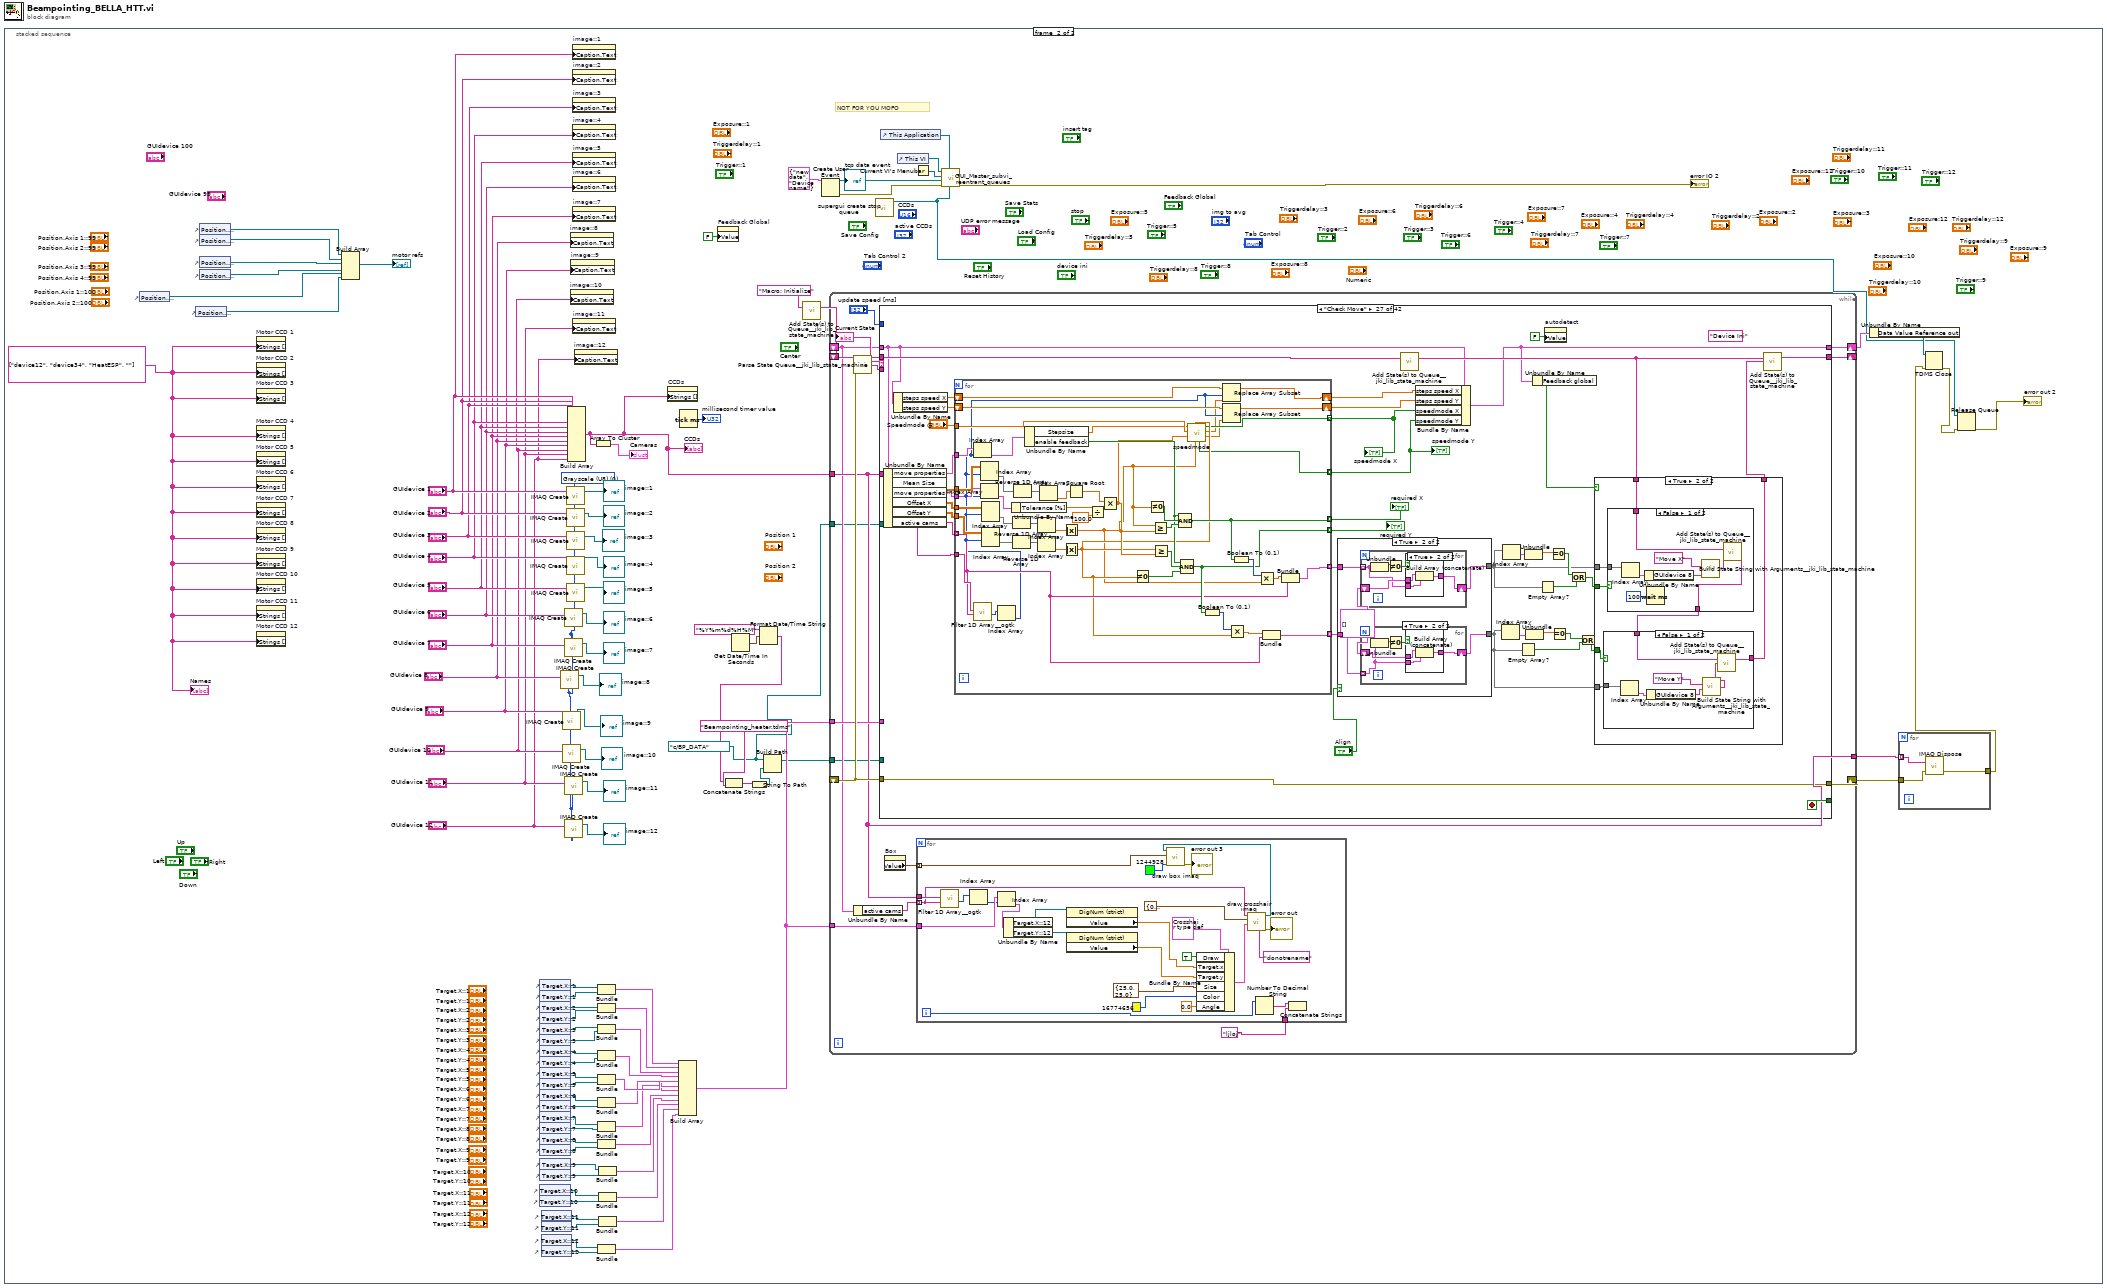
[diagram p0: block diagram]
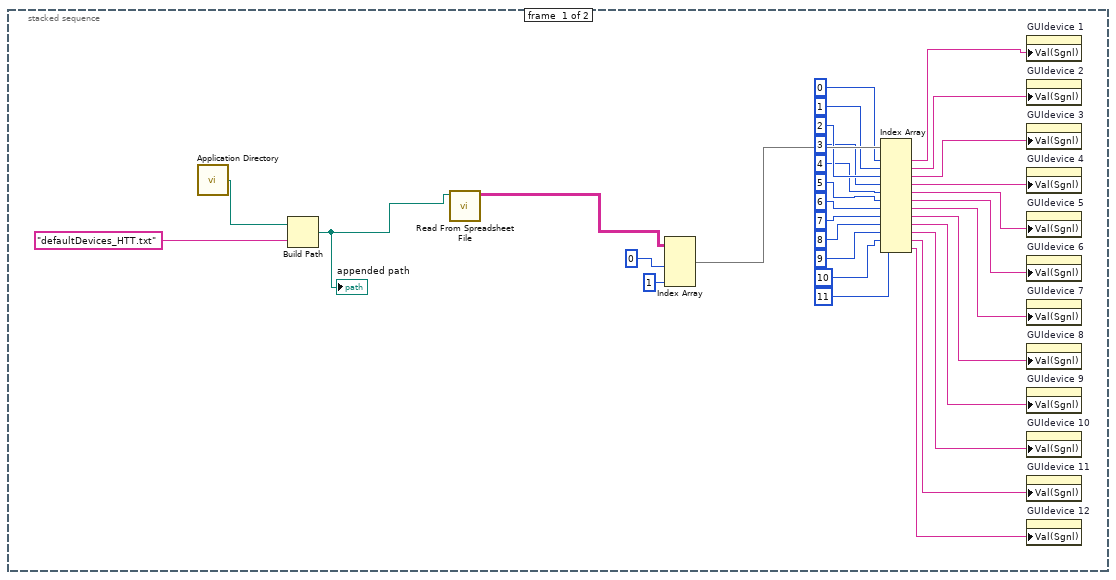
[diagram p2: hidden frame]
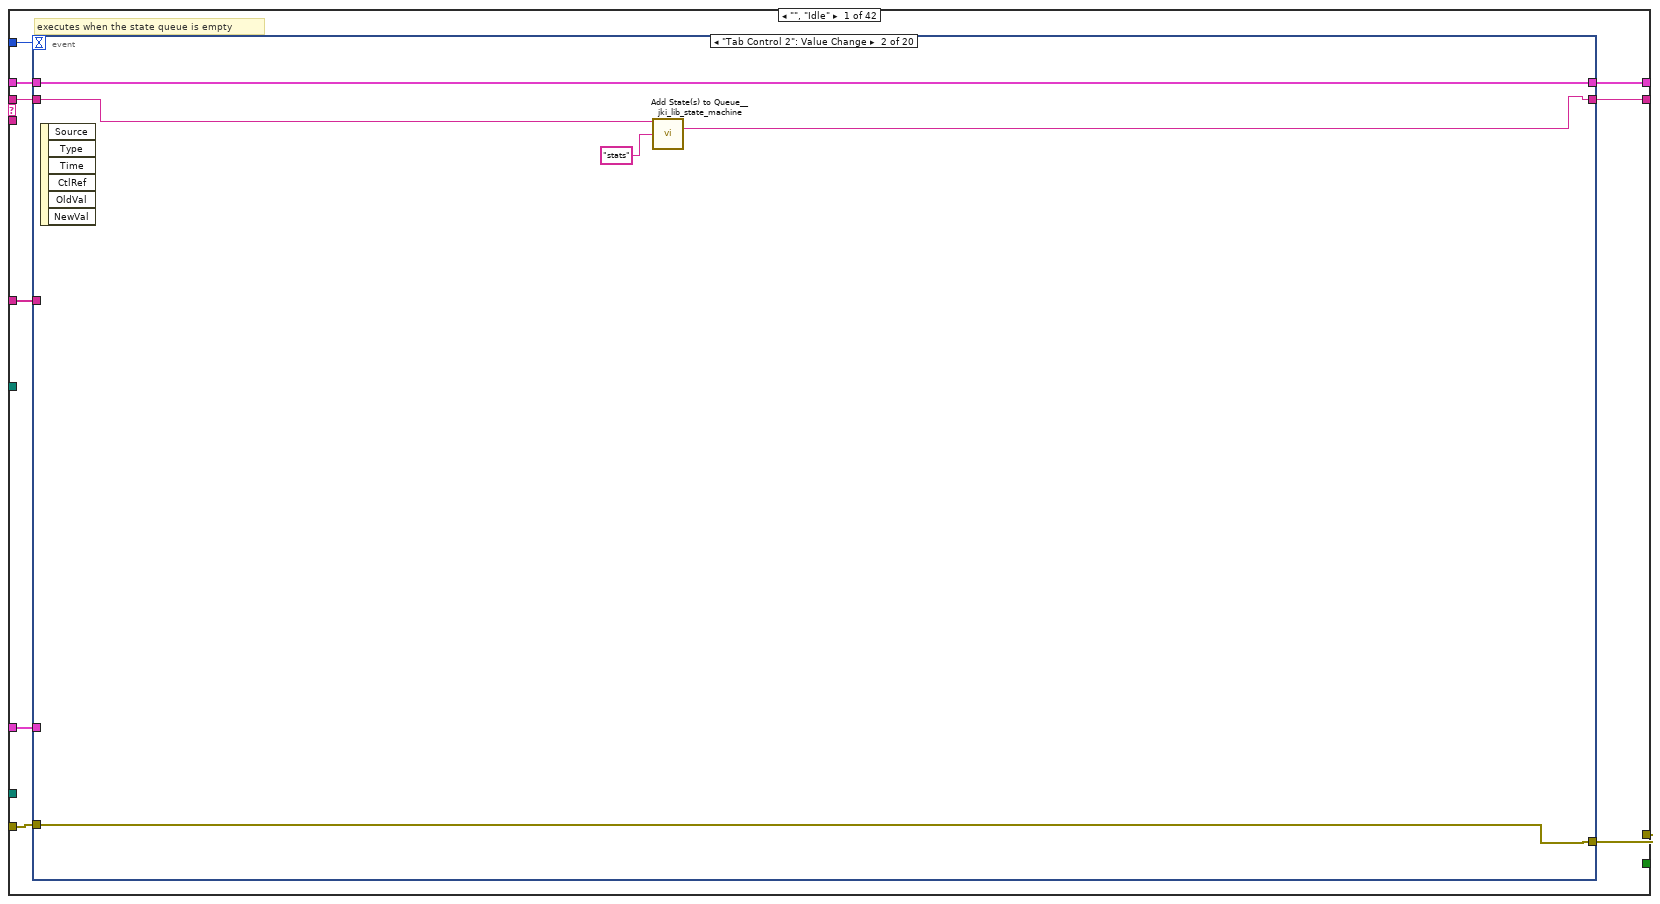
[diagram p3: hidden frame]
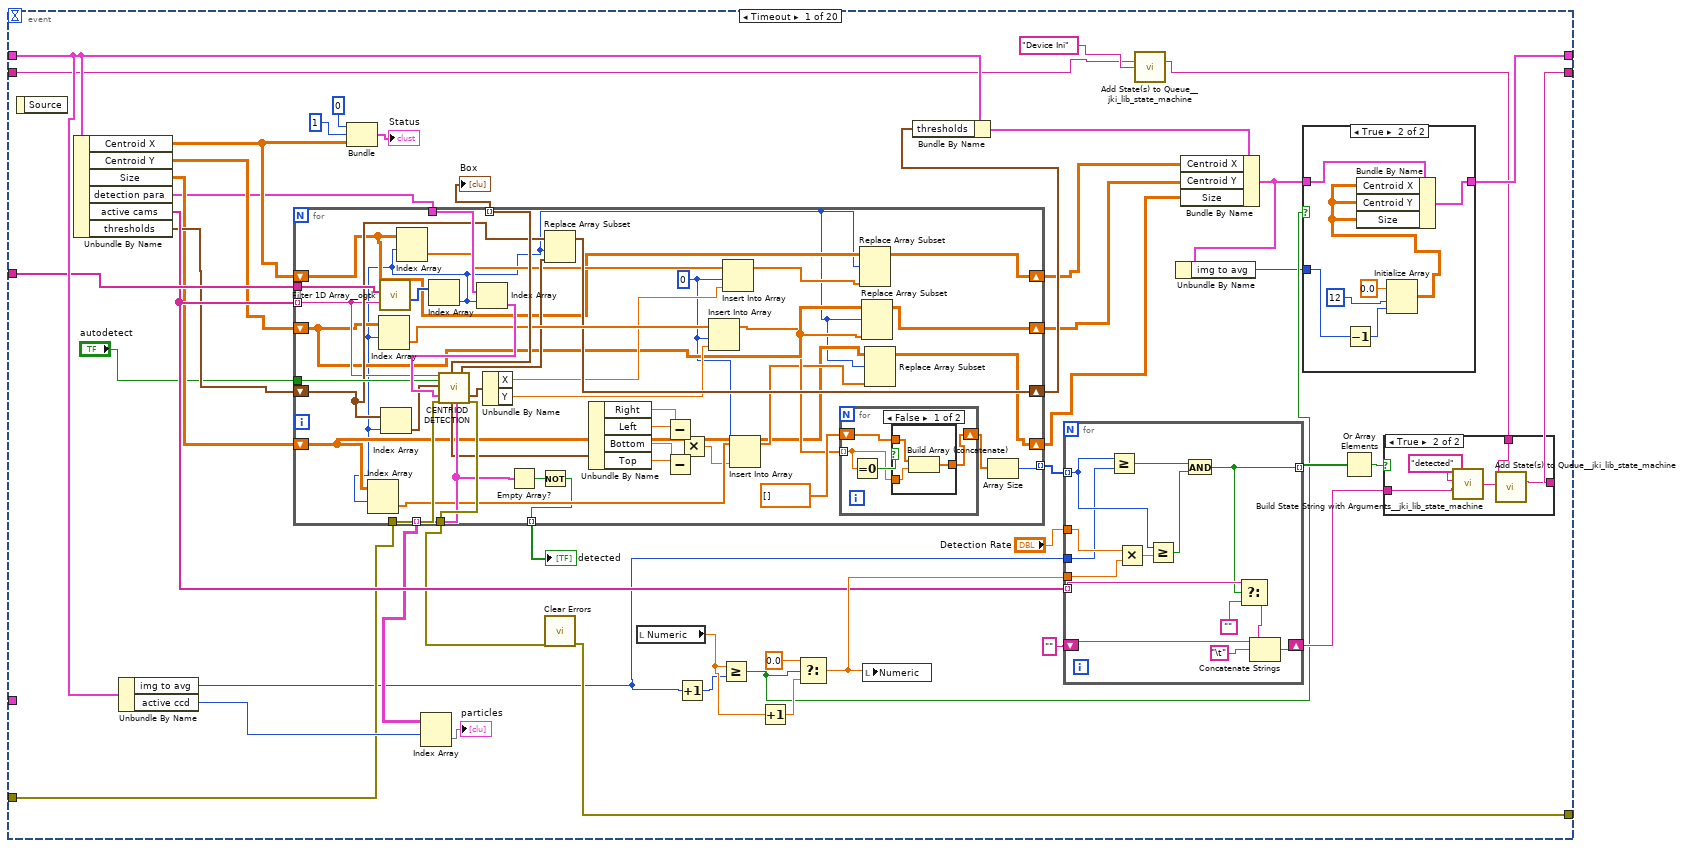
[diagram p4: hidden frame]
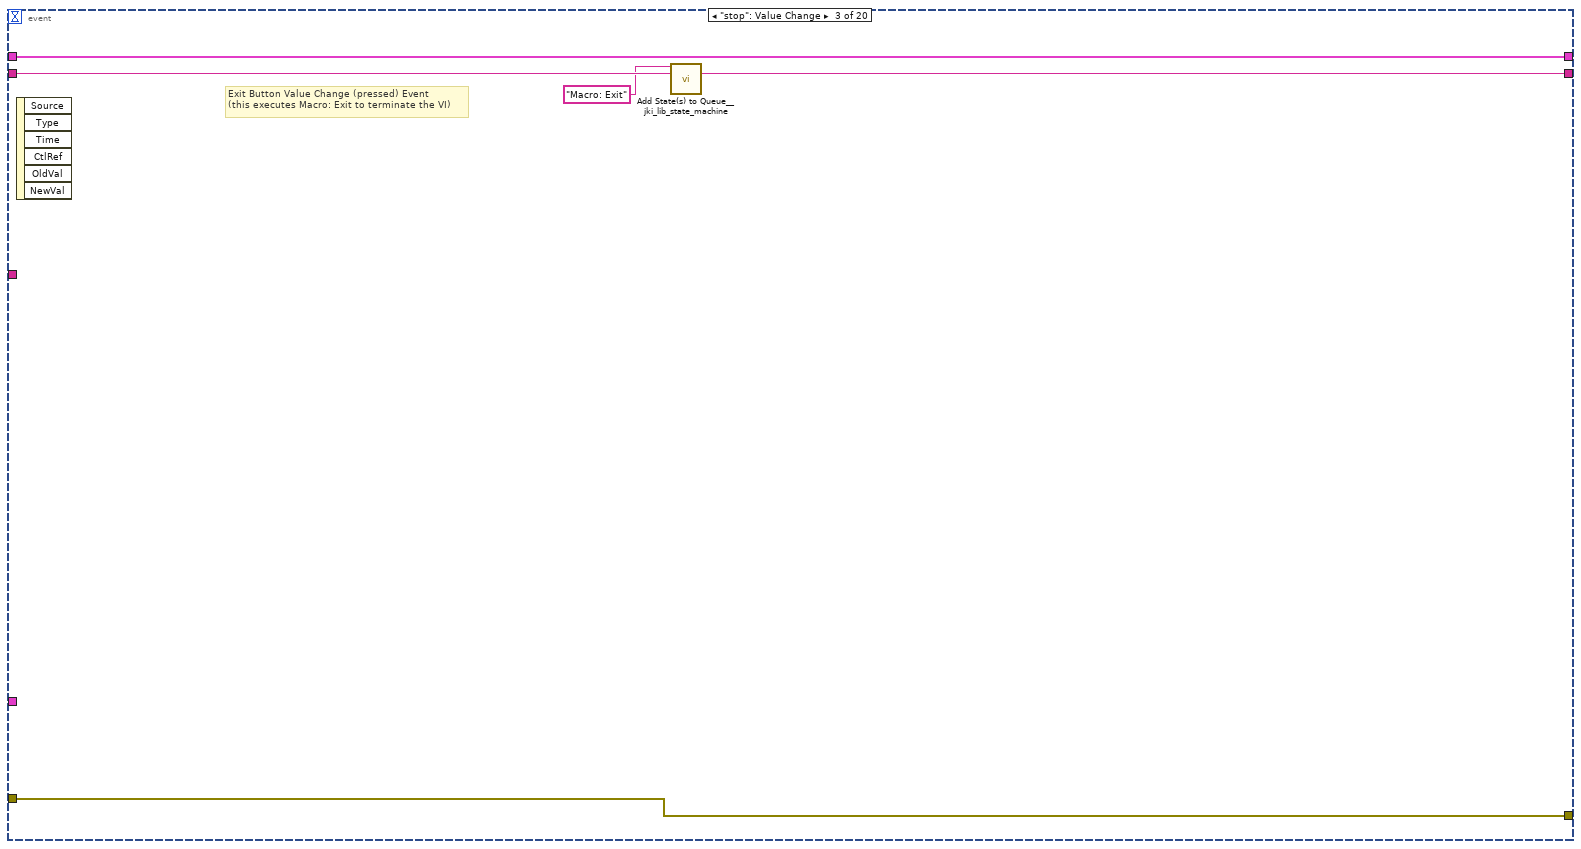
[diagram p8: hidden frame]
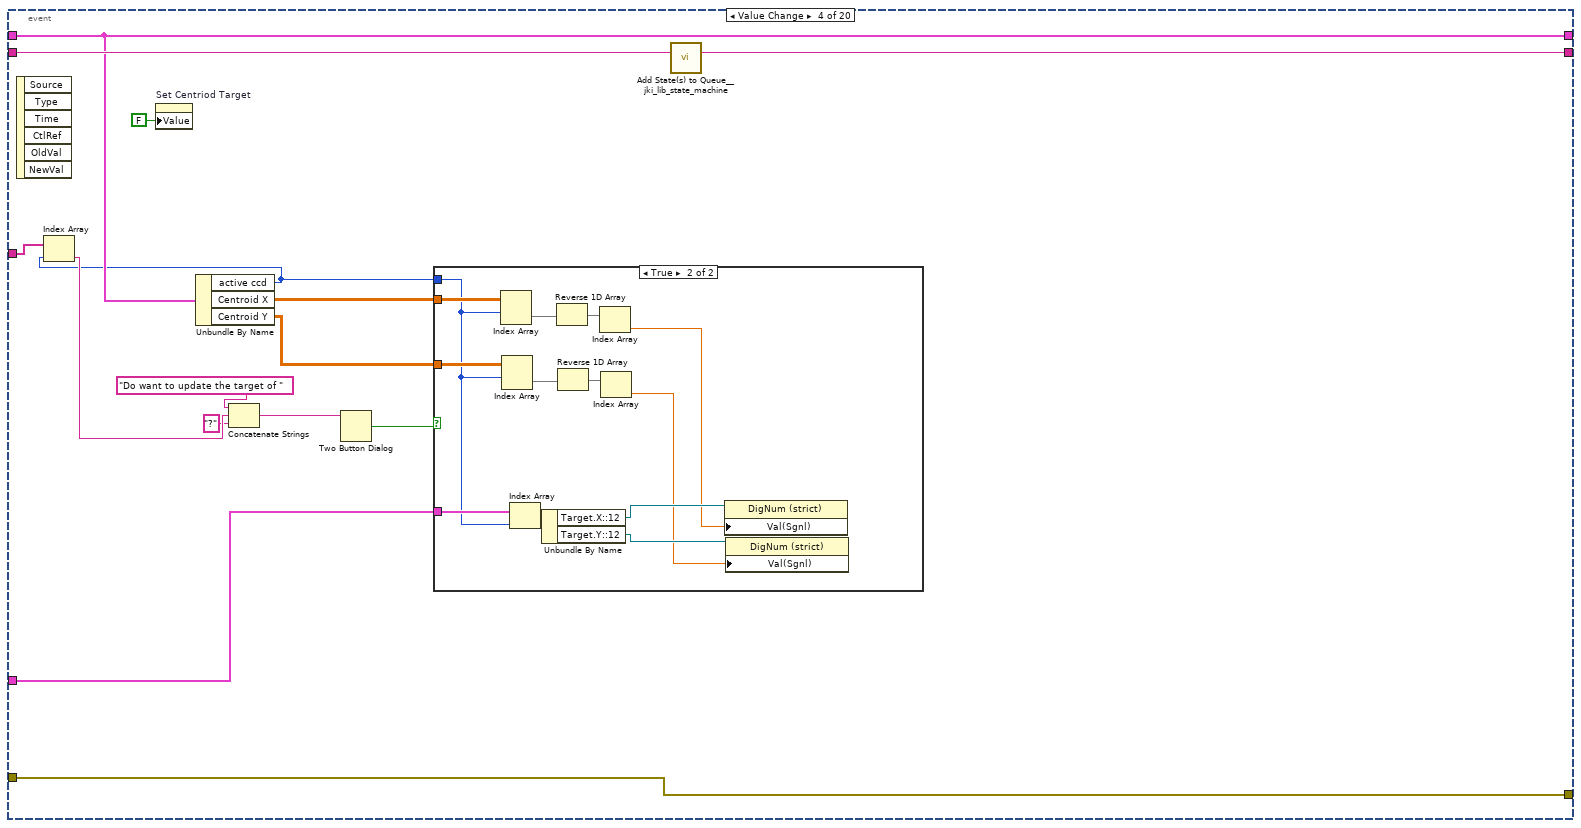
[diagram p9: hidden frame]
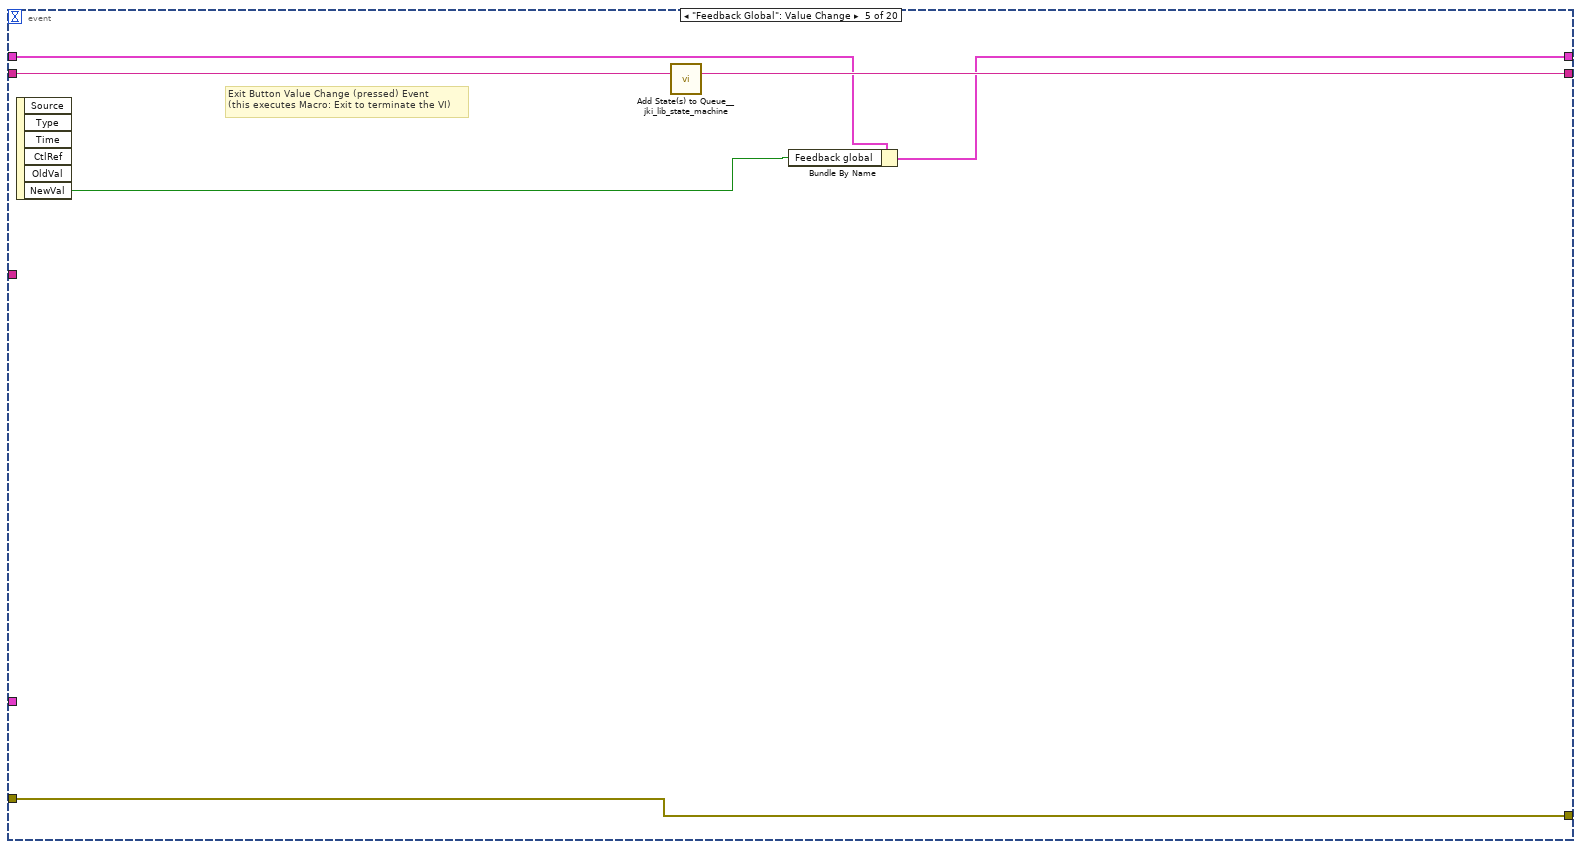
[diagram p11: hidden frame]
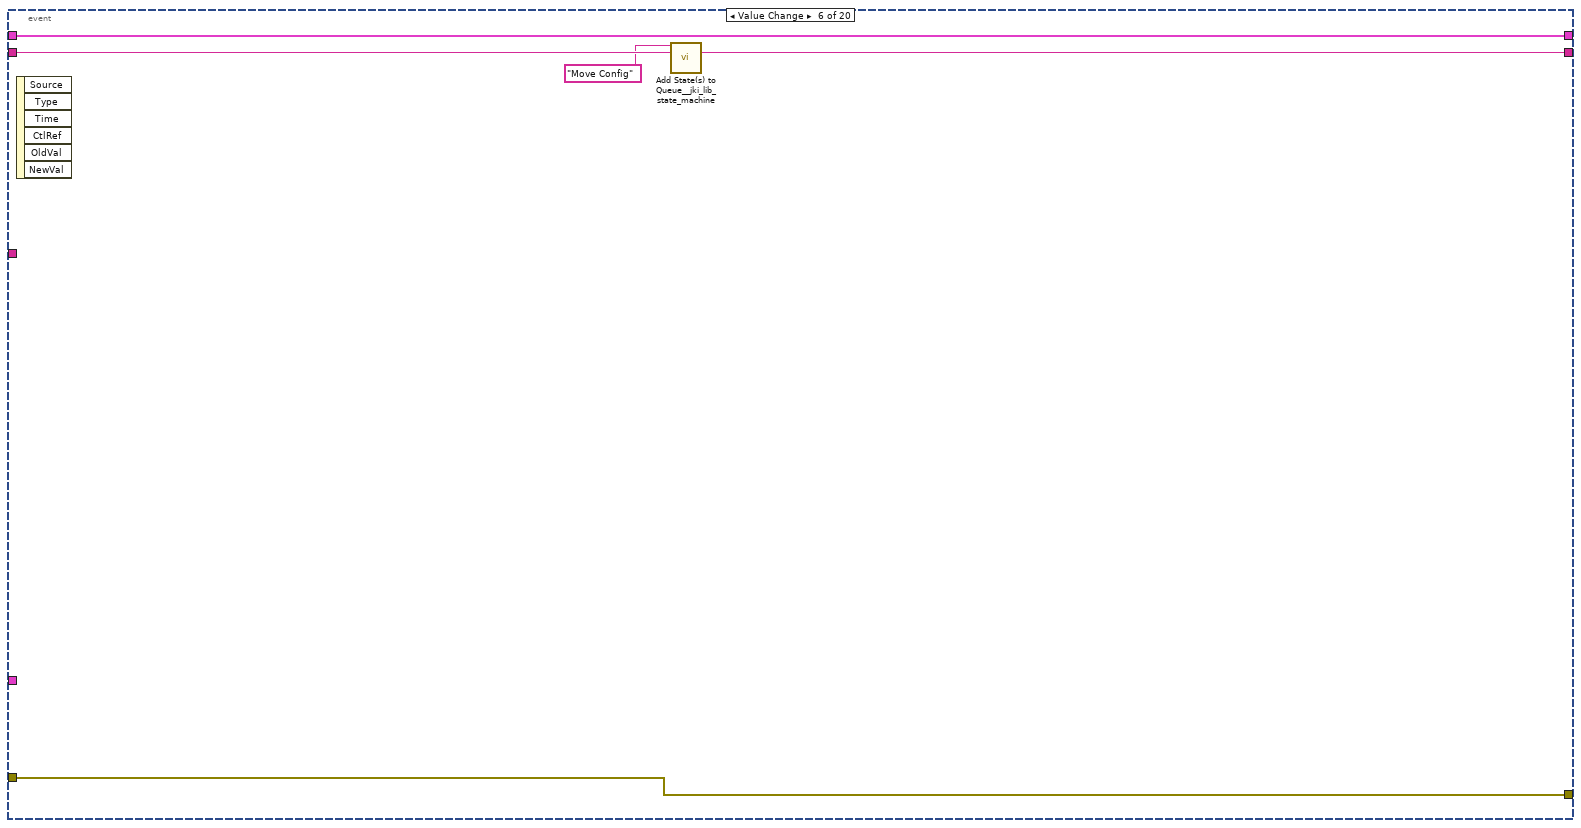
[diagram p12: hidden frame]
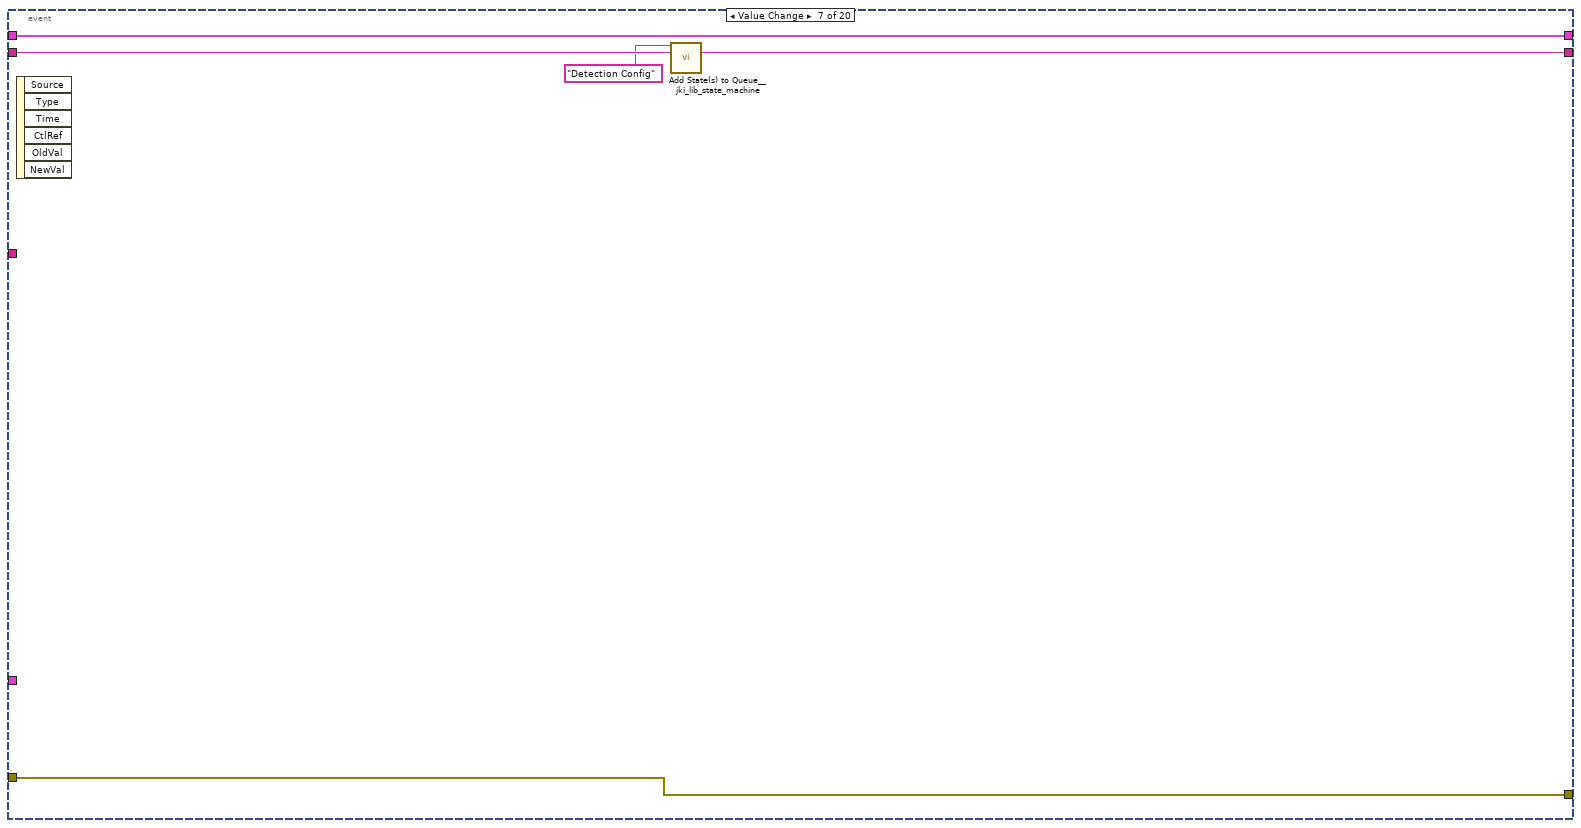
[diagram p13: hidden frame]
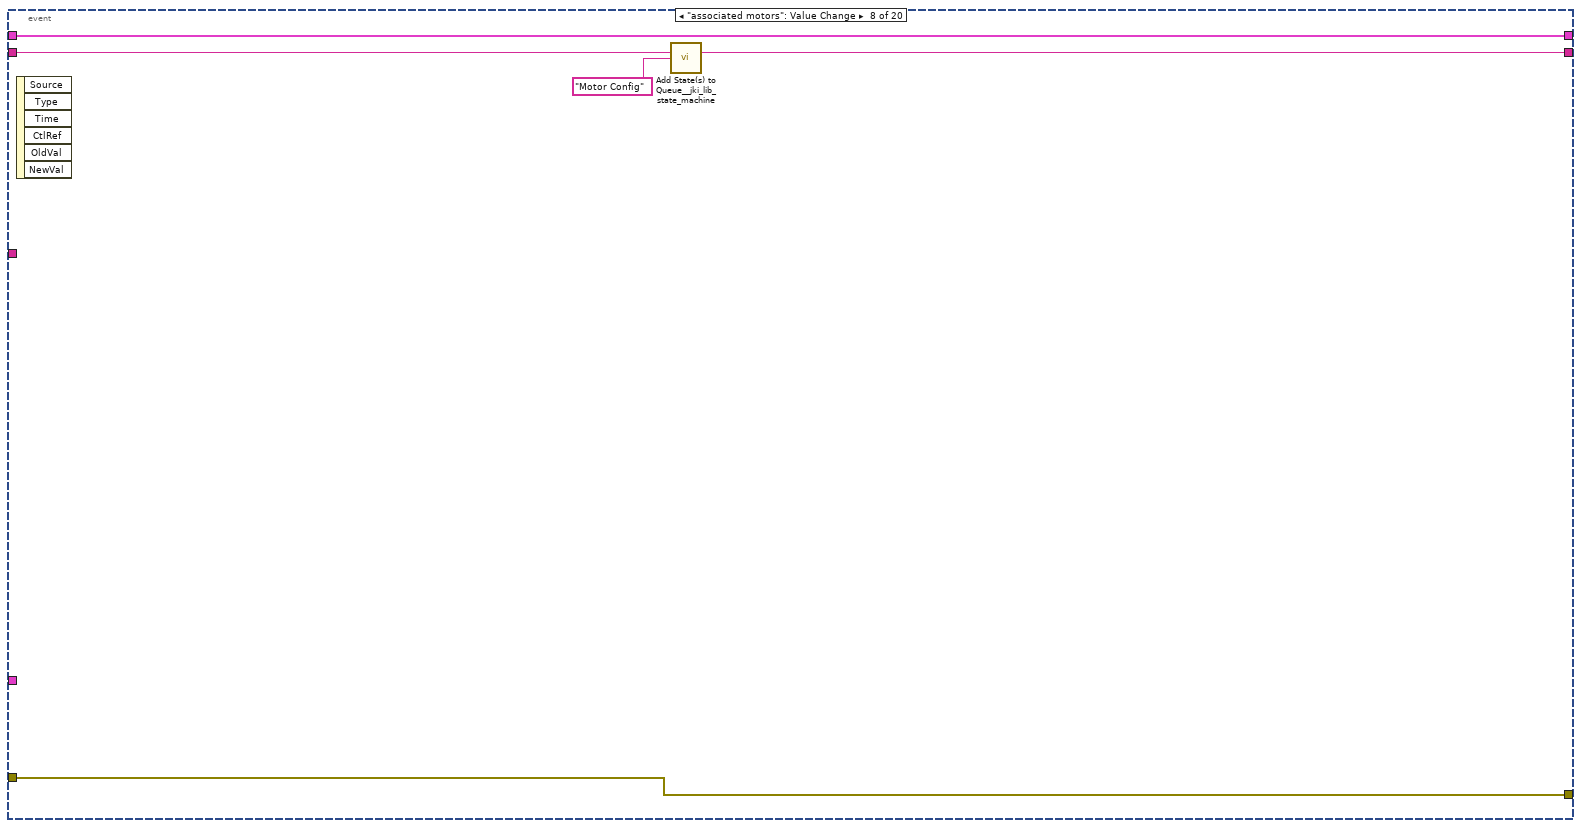
[diagram p14: hidden frame]
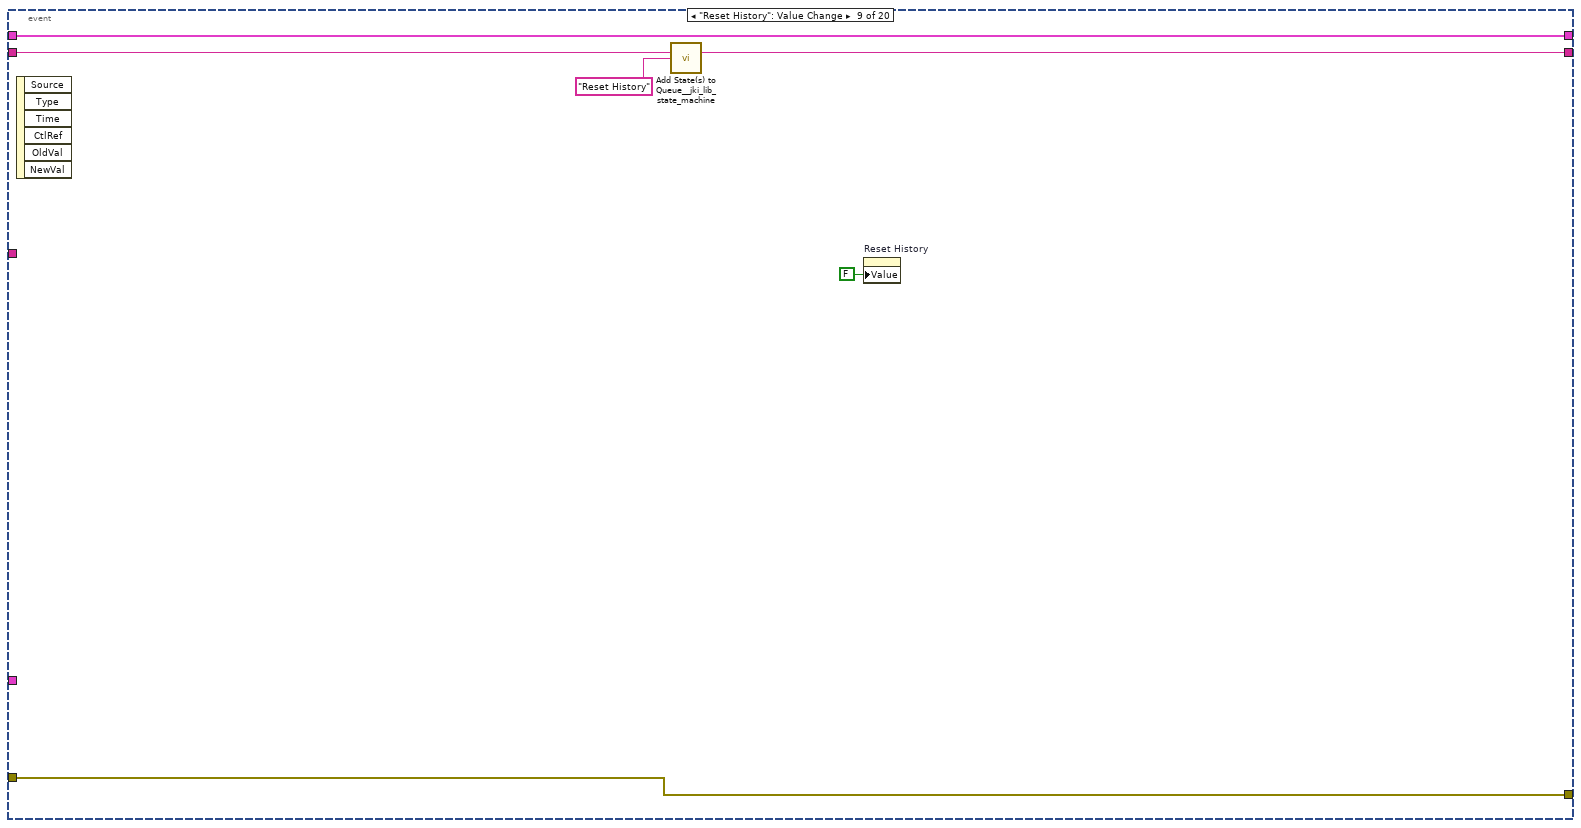
[diagram p15: hidden frame]
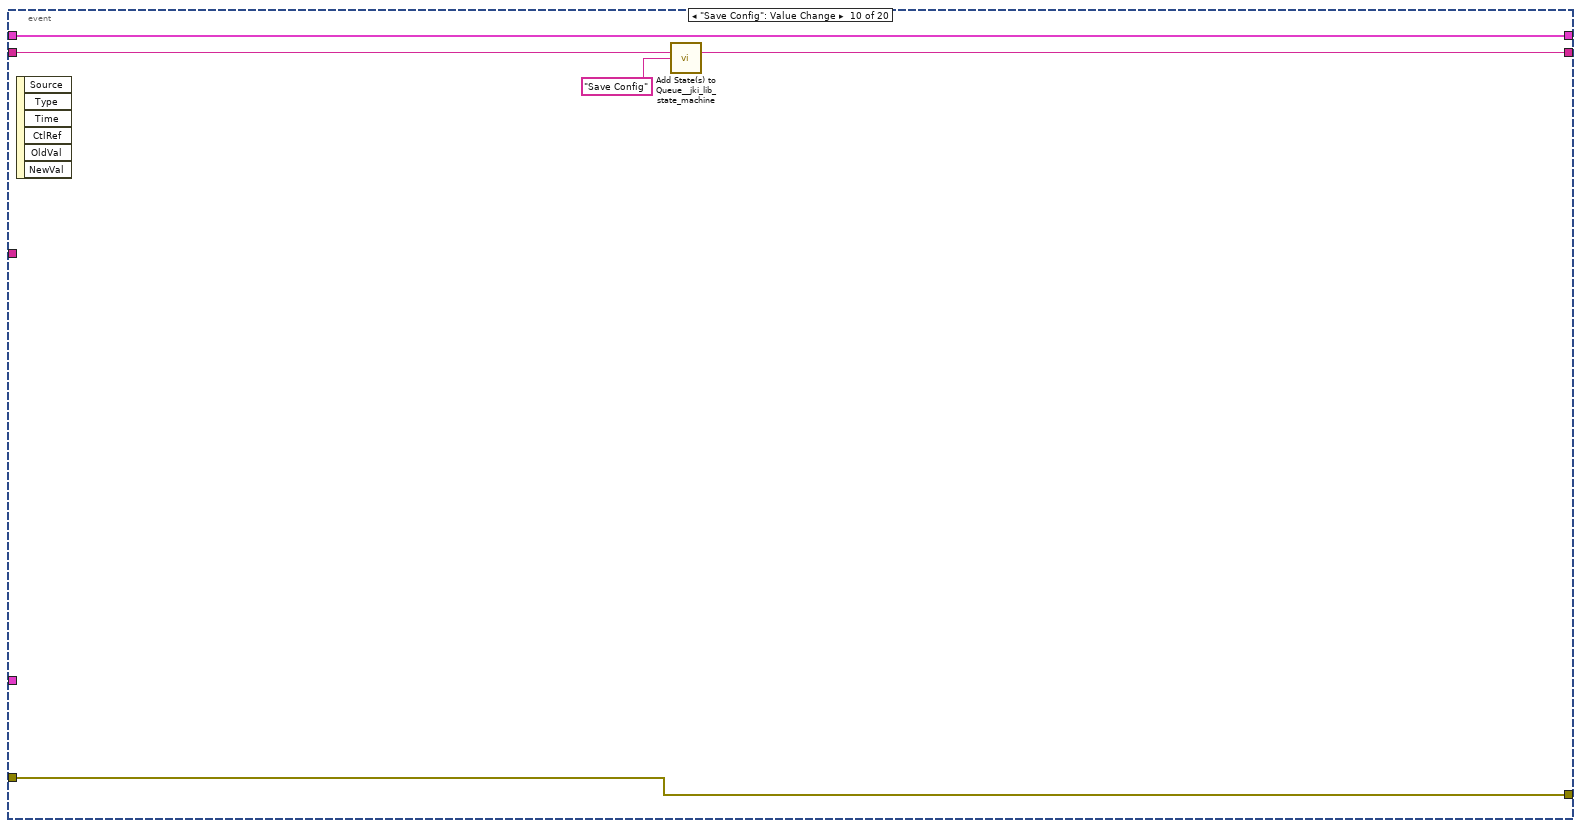
[diagram p16: hidden frame]
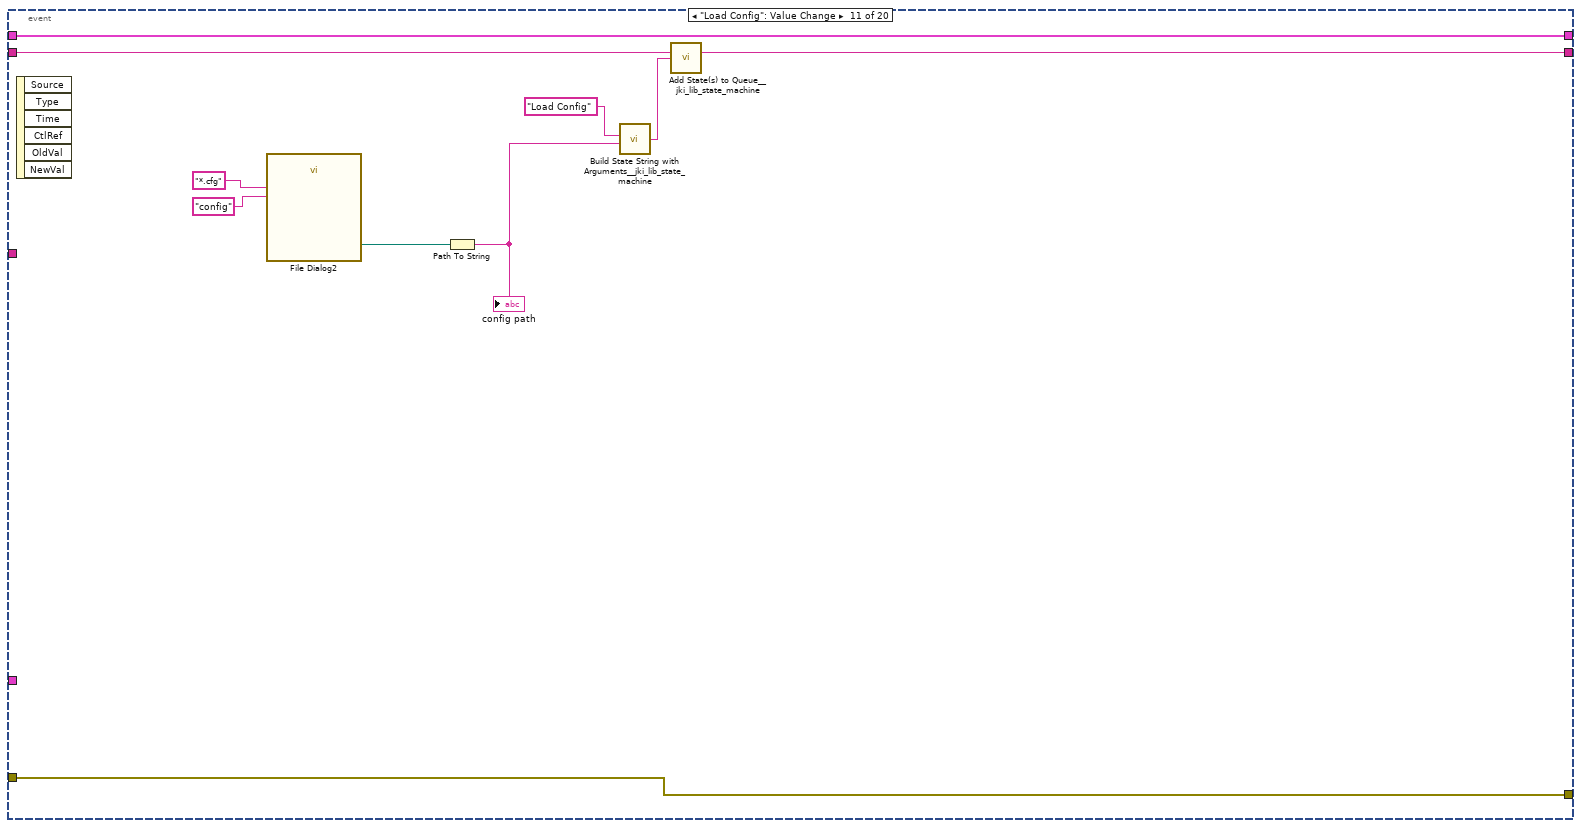
[diagram p17: hidden frame]
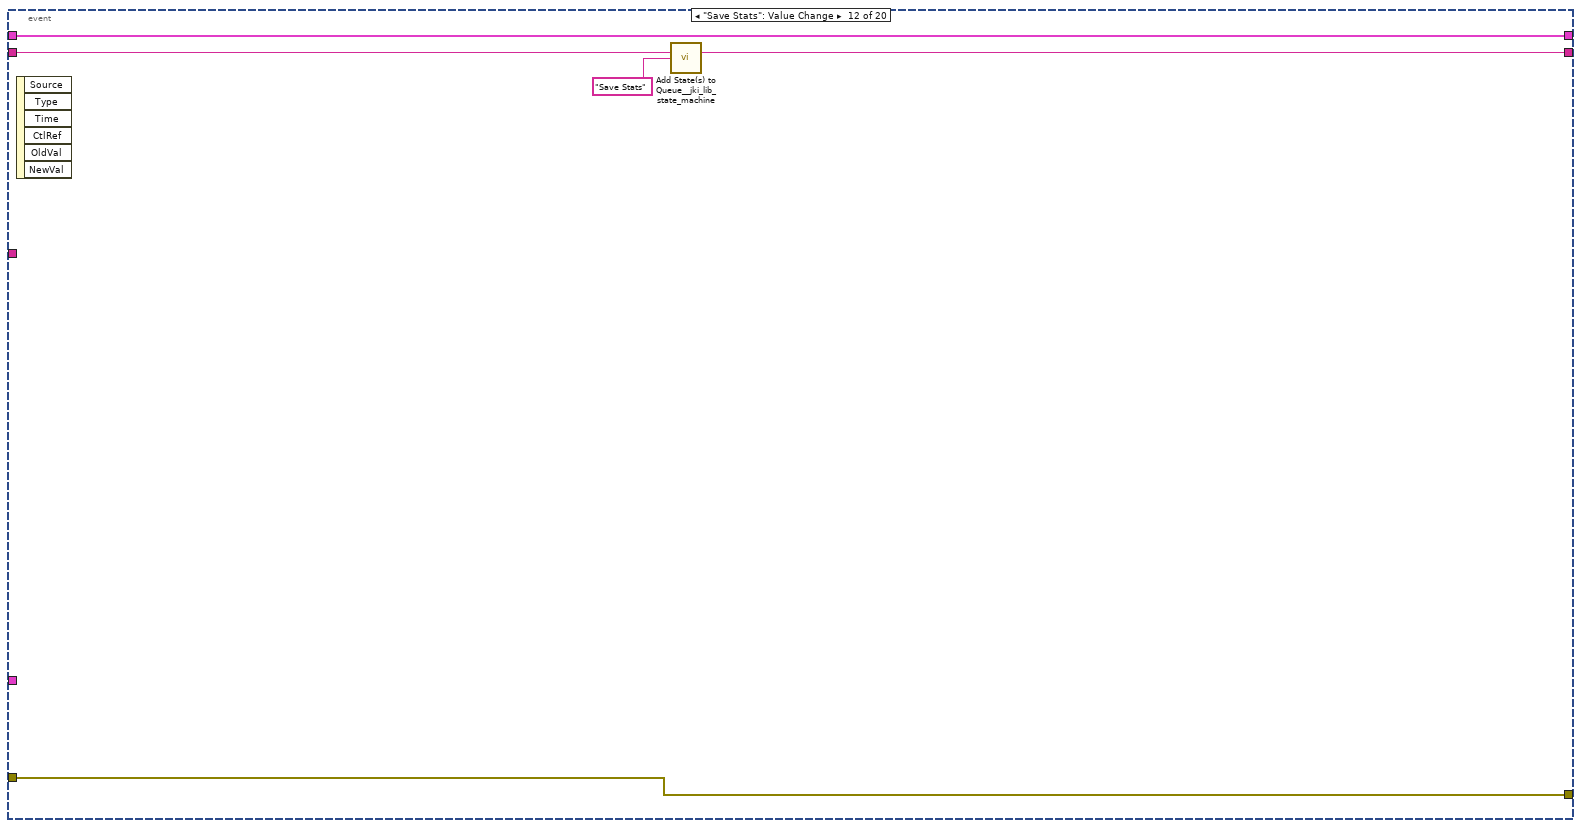
[diagram p18: hidden frame]
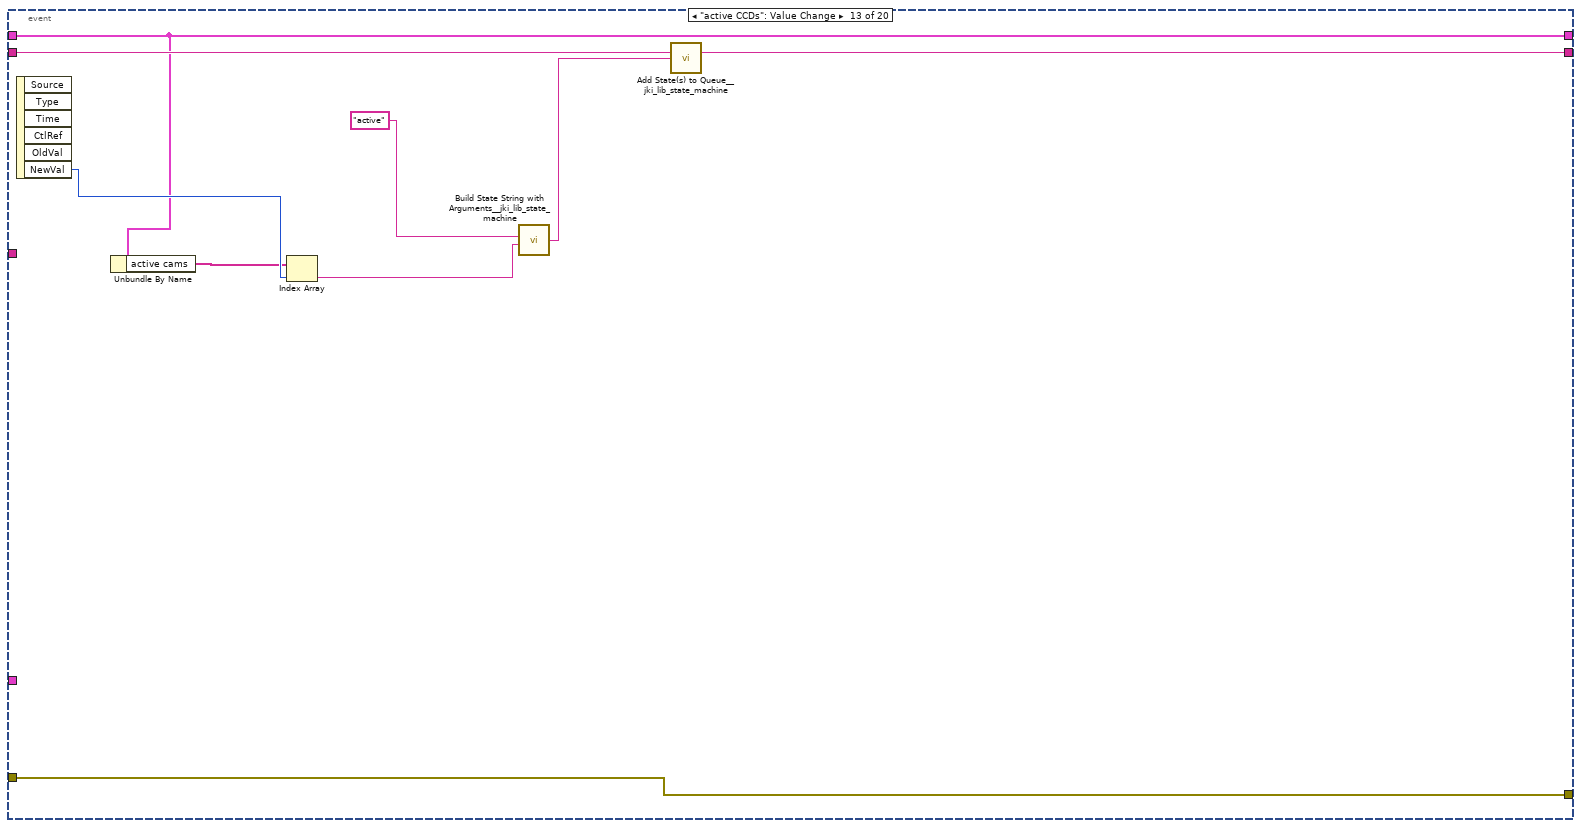
[diagram p19: hidden frame]
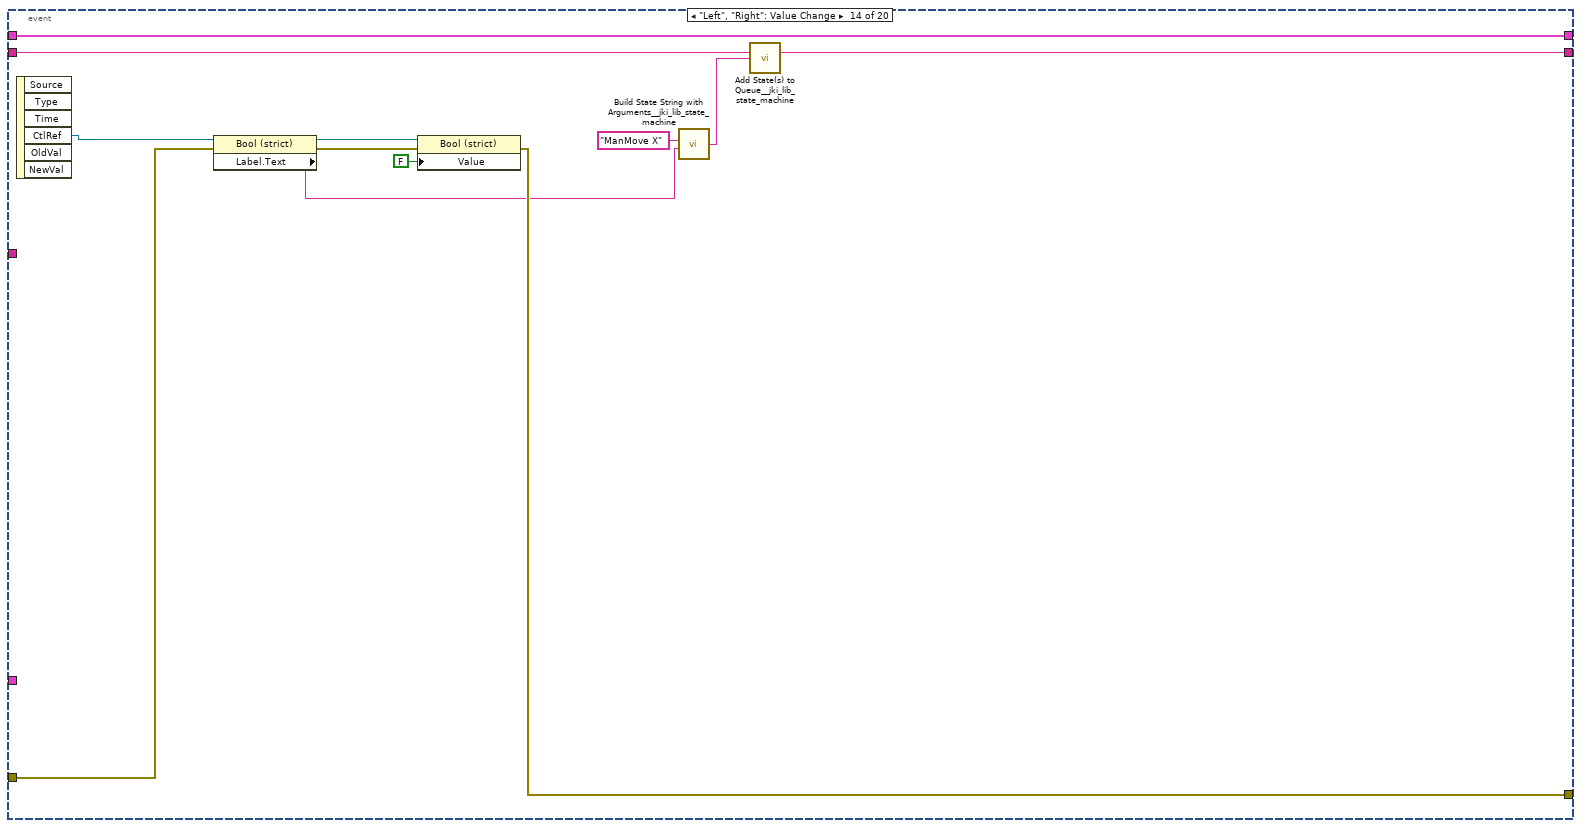
[diagram p20: hidden frame]
diagram:
  n1 = stacked-sequence {
    frame #0 {
      n2 = call <vilib>:"Application Directory.vi"() -> ("Application Directory"=w31:path)
      n3 = Build Path(base path=w31, name or relative path="defaultDevices_HTT.txt") -> (appended path=w29:path)
      "appended path" <- w29
      n4 = call-poly <vilib>:"Read From Spreadsheet File.vi"("file path (dialog if empty)"=w29) -> ("all rows"=w28:string[][])  [unwired: 6 in, 4 out]
      n5 = Index Array(array=w28, index (col) #1=0 ("disabled index (col)"), index (col) #2=1 ("index (col)")) -> (element #1=w25:string[])  [unwired: 2 in, 1 out]
      n6 = Index Array(array=w25, index #1=0 ("index"), index #2=1 ("index"), index #3=2 ("index"), index #4=3 ("index"), index #5=4 ("index"), index #6=5 ("index"), index #7=6 ("index"), index #8=7 ("index"), index #9=8 ("index"), index #10=9 ("index"), index #11=10 ("index"), index #12=11 ("index")) -> (element #1=w12:string, element #2=w11:string, element #3=w10:string, element #4=w9:string, element #5=w8:string, element #6=w7:string, element #7=w6:string, element #8=w5:string, element #9=w4:string, element #10=w3:string, element #11=w2:string, element #12=w1:string)
      n7 = property on="GUIdevice 1" class="Str"("Val(Sgnl)"=w12) -> ()  [unwired: 2 in, 2 out]
      n8 = property on="GUIdevice 2" class="Str"("Val(Sgnl)"=w11) -> ()  [unwired: 2 in, 2 out]
      n9 = property on="GUIdevice 3" class="Str"("Val(Sgnl)"=w10) -> ()  [unwired: 2 in, 2 out]
      n10 = property on="GUIdevice 4" class="Str"("Val(Sgnl)"=w9) -> ()  [unwired: 2 in, 2 out]
      n11 = property on="GUIdevice 5" class="Str"("Val(Sgnl)"=w8) -> ()  [unwired: 2 in, 2 out]
      n12 = property on="GUIdevice 6" class="Str"("Val(Sgnl)"=w7) -> ()  [unwired: 2 in, 2 out]
      n13 = property on="GUIdevice 7" class="Str"("Val(Sgnl)"=w6) -> ()  [unwired: 2 in, 2 out]
      n14 = property on="GUIdevice 8" class="Str"("Val(Sgnl)"=w5) -> ()  [unwired: 2 in, 2 out]
      n15 = property on="GUIdevice 9" class="Str"("Val(Sgnl)"=w4) -> ()  [unwired: 2 in, 2 out]
      n16 = property on="GUIdevice 10" class="Str"("Val(Sgnl)"=w3) -> ()  [unwired: 2 in, 2 out]
      n17 = property on="GUIdevice 11" class="Str"("Val(Sgnl)"=w2) -> ()  [unwired: 2 in, 2 out]
      n18 = property on="GUIdevice 12" class="Str"("Val(Sgnl)"=w1) -> ()  [unwired: 2 in, 2 out]
    }
    frame #1 {
      w37 = path "c:/BP_DATA" ("base path")
      w39 = string[] ["device12", "device34", "HeatESP", ""] ("elements")
      w43 = T21 0 items=["Grayscale (U8)", "Grayscale (I16)", "Grayscale (SGL)", "Complex (CSG)", "RGB (U32)", "HSL (U32)", "RGB (U64)", "Grayscale (U16)"] ("Image Type")
      # "NOT FOR YOU MOFO"
      n19 = control-ref of="Position.Axis 1::100"() -> (w36:refnum<vi>)
      n20 = control-ref of="Position.Axis 2::100"() -> (w35:refnum<vi>)
      n21 = control-ref of="Position.Axis 1::99"() -> (w114:refnum<vi>)
      n22 = control-ref of="Position.Axis 2::99"() -> (w113:refnum<vi>)
      n23 = control-ref of="Position.Axis 3::99"() -> (w112:refnum<vi>)
      n24 = control-ref of="Position.Axis 4::99"() -> (w111:refnum<vi>)
      n25 = property on="Motor CCD 1" class="Ring (strict)"("Strings []"=w39) -> ()  [unwired: 2 in, 2 out]
      n26 = property on="Motor CCD 2" class="Ring (strict)"("Strings []"=w39) -> ()  [unwired: 2 in, 2 out]
      n27 = property on="Motor CCD 3" class="Ring (strict)"("Strings []"=w39) -> ()  [unwired: 2 in, 2 out]
      n28 = property on="Motor CCD 4" class="Ring (strict)"("Strings []"=w39) -> ()  [unwired: 2 in, 2 out]
      n29 = property on="Motor CCD 5" class="Ring (strict)"("Strings []"=w39) -> ()  [unwired: 2 in, 2 out]
      n30 = property on="Motor CCD 6" class="Ring (strict)"("Strings []"=w39) -> ()  [unwired: 2 in, 2 out]
      n31 = property on="Motor CCD 7" class="Ring (strict)"("Strings []"=w39) -> ()  [unwired: 2 in, 2 out]
      n32 = property on="Motor CCD 8" class="Ring (strict)"("Strings []"=w39) -> ()  [unwired: 2 in, 2 out]
      n33 = property on="Motor CCD 9" class="Ring (strict)"("Strings []"=w39) -> ()  [unwired: 2 in, 2 out]
      n34 = property on="Motor CCD 10" class="Ring (strict)"("Strings []"=w39) -> ()  [unwired: 2 in, 2 out]
      n35 = property on="Motor CCD 11" class="Ring (strict)"("Strings []"=w39) -> ()  [unwired: 2 in, 2 out]
      n36 = property on="Motor CCD 12" class="Ring (strict)"("Strings []"=w39) -> ()  [unwired: 2 in, 2 out]
      n37 = Build Array(w114, w113, w112, w111, w36, w35) -> (→"motor refs":refnum<vi>[])
      n38 = control-ref of="Target.X::1"() -> (w97:refnum<vi>)
      n39 = control-ref of="Target.Y::1"() -> (w96:refnum<vi>)
      n40 = control-ref of="Target.X::2"() -> (w95:refnum<vi>)
      n41 = control-ref of="Target.Y::2"() -> (w94:refnum<vi>)
      n42 = control-ref of="Target.X::3"() -> (w93:refnum<vi>)
      n43 = control-ref of="Target.Y::3"() -> (w92:refnum<vi>)
      n44 = control-ref of="Target.X::4"() -> (w91:refnum<vi>)
      n45 = control-ref of="Target.Y::4"() -> (w90:refnum<vi>)
      n46 = control-ref of="Target.X::5"() -> (w89:refnum<vi>)
      n47 = control-ref of="Target.Y::5"() -> (w88:refnum<vi>)
      n48 = control-ref of="Target.X::6"() -> (w87:refnum<vi>)
      n49 = control-ref of="Target.Y::6"() -> (w86:refnum<vi>)
      n50 = control-ref of="Target.X::7"() -> (w85:refnum<vi>)
      n51 = control-ref of="Target.Y::7"() -> (w84:refnum<vi>)
      n52 = control-ref of="Target.X::8"() -> (w83:refnum<vi>)
      n53 = control-ref of="Target.Y::8"() -> (w82:refnum<vi>)
      n54 = control-ref of="Target.X::9"() -> (w60:refnum<vi>)
      n55 = control-ref of="Target.Y::9"() -> (w59:refnum<vi>)
      n56 = control-ref of="Target.X::10"() -> (w58:refnum<vi>)
      n57 = control-ref of="Target.Y::10"() -> (w57:refnum<vi>)
      n58 = control-ref of="Target.X::11"() -> (w56:refnum<vi>)
      n59 = control-ref of="Target.Y::11"() -> (w55:refnum<vi>)
      n60 = control-ref of="Target.X::12"() -> (w54:refnum<vi>)
      n61 = control-ref of="Target.Y::12"() -> (w53:refnum<vi>)
      n62 = call "IMAQ Create"("Image Name"="GUIdevice 8", "Image Type"=w43) -> ("New Image"=→"image::8":T9)  [unwired: 3 in, 1 out]
      n63 = call "IMAQ Create"("Image Name"="GUIdevice 9", "Image Type"=w43) -> ("New Image"=→"image::9":T9)  [unwired: 3 in, 1 out]
      n64 = call "IMAQ Create"("Image Name"="GUIdevice 10", "Image Type"=w43) -> ("New Image"=→"image::10":T9)  [unwired: 3 in, 1 out]
      n65 = call "IMAQ Create"("Image Name"="GUIdevice 6", "Image Type"=w43) -> ("New Image"=→"image::6":T9)  [unwired: 3 in, 1 out]
      n66 = call "IMAQ Create"("Image Name"="GUIdevice 7", "Image Type"=w43) -> ("New Image"=→"image::7":T9)  [unwired: 3 in, 1 out]
      n67 = call "IMAQ Create"("Image Name"="GUIdevice 11", "Image Type"=w43) -> ("New Image"=→"image::11":T9)  [unwired: 3 in, 1 out]
      n68 = call "IMAQ Create"("Image Name"="GUIdevice 12", "Image Type"=w43) -> ("New Image"=→"image::12":T9)  [unwired: 3 in, 1 out]
      n69 = call "IMAQ Create"("Image Name"="GUIdevice 2") -> ("New Image"=→"image::2":T9)  [unwired: 4 in, 1 out]
      n70 = call "IMAQ Create"("Image Name"="GUIdevice 4", "Image Type"=w43) -> ("New Image"=→"image::4":T9)  [unwired: 3 in, 1 out]
      n71 = call "IMAQ Create"("Image Name"="GUIdevice 1", "Image Type"=w43) -> ("New Image"=→"image::1":T9)  [unwired: 3 in, 1 out]
      n72 = call "IMAQ Create"("Image Name"="GUIdevice 3", "Image Type"=w43) -> ("New Image"=→"image::3":T9)  [unwired: 3 in, 1 out]
      n73 = call "IMAQ Create"("Image Name"="GUIdevice 5", "Image Type"=w43) -> ("New Image"=→"image::5":T9)  [unwired: 3 in, 1 out]
      n74 = Build Array("GUIdevice 1", "GUIdevice 2", "GUIdevice 3", "GUIdevice 4", "GUIdevice 5", "GUIdevice 6", "GUIdevice 7", "GUIdevice 8", "GUIdevice 9", "GUIdevice 10", "GUIdevice 11", "GUIdevice 12") -> (w71:string[])
      "CCDs" <- w71
      n75 = property on="image::8" class="ImageControl"("Caption.Text"="GUIdevice 8") -> ()  [unwired: 2 in, 2 out]
      n76 = property on="image::10" class="ImageControl"("Caption.Text"="GUIdevice 10") -> ()  [unwired: 2 in, 2 out]
      n77 = property on="image::9" class="ImageControl"("Caption.Text"="GUIdevice 9") -> ()  [unwired: 2 in, 2 out]
      n78 = property on="image::1" class="ImageControl"("Caption.Text"="GUIdevice 1") -> ()  [unwired: 2 in, 2 out]
      n79 = property on="image::2" class="ImageControl"("Caption.Text"="GUIdevice 2") -> ()  [unwired: 2 in, 2 out]
      n80 = property on="image::3" class="ImageControl"("Caption.Text"="GUIdevice 3") -> ()  [unwired: 2 in, 2 out]
      n81 = property on="image::4" class="ImageControl"("Caption.Text"="GUIdevice 4") -> ()  [unwired: 2 in, 2 out]
      n82 = property on="image::5" class="ImageControl"("Caption.Text"="GUIdevice 5") -> ()  [unwired: 2 in, 2 out]
      n83 = property on="image::6" class="ImageControl"("Caption.Text"="GUIdevice 6") -> ()  [unwired: 2 in, 2 out]
      n84 = property on="image::7" class="ImageControl"("Caption.Text"="GUIdevice 7") -> ()  [unwired: 2 in, 2 out]
      n85 = property on="image::11" class="ImageControl"("Caption.Text"="GUIdevice 11") -> ()  [unwired: 2 in, 2 out]
      n86 = property on="image::12" class="ImageControl"("Caption.Text"="GUIdevice 12") -> ()  [unwired: 2 in, 2 out]
      n87 = Array To Cluster(array=w71) -> (cluster=→"Cameras":T22)
      n88 = Bundle("Target.X::1"=w97, "Target.Y::1"=w96) -> (w81:T23)  [unwired: 1 in]
      n89 = Bundle("Target.X::2"=w95, "Target.Y::2"=w94) -> (w80:T24)  [unwired: 1 in]
      n90 = Bundle("Target.X::3"=w93, "Target.Y::3"=w92) -> (w79:T25)  [unwired: 1 in]
      n91 = Bundle("Target.X::4"=w91, "Target.Y::4"=w90) -> (w72:T26)  [unwired: 1 in]
      n92 = Bundle("Target.X::5"=w89, "Target.Y::5"=w88) -> (w78:T27)  [unwired: 1 in]
      n93 = Bundle("Target.X::6"=w87, "Target.Y::6"=w86) -> (w77:T28)  [unwired: 1 in]
      n94 = Bundle("Target.X::7"=w85, "Target.Y::7"=w84) -> (w76:T29)  [unwired: 1 in]
      n95 = Bundle("Target.X::8"=w83, "Target.Y::8"=w82) -> (w75:T30)  [unwired: 1 in]
      n96 = Bundle("Target.X::12"=w54, "Target.Y::12"=w53) -> (w49:T31)  [unwired: 1 in]
      n97 = Bundle("Target.X::9"=w60, "Target.Y::9"=w59) -> (w52:T32)  [unwired: 1 in]
      n98 = Bundle("Target.X::10"=w58, "Target.Y::10"=w57) -> (w51:T33)  [unwired: 1 in]
      n99 = Bundle("Target.X::11"=w56, "Target.Y::11"=w55) -> (w50:T34)  [unwired: 1 in]
      n100 = property on="CCDs" class="Ring (strict)"("Strings []"=w71) -> ()  [unwired: 2 in, 2 out]
      n101 = Build Array(w81, w80, w79, w72, w78, w77, w76, w75, w52, w51, w50, w49) -> (w74:T35)
      n102 = Tick Count (ms)() -> (millisecond timer value=→"millisecond timer value":u32)
      n103 = property on="Feedback Global" class="Bool (strict)"("Value"=FALSE ("Feedback Global")) -> ()  [unwired: 2 in, 2 out]
      n104 = Get Date/Time In Seconds() -> (seconds since 1Jan1904=w62:timestamp)
      n105 = Format Date/Time String(time format string (%c)="%Y%m%d%H%M", seconds (now)=w62) -> (date/time string=w61:string)  [unwired: 1 in]
      n106 = Concatenate Strings(w61, "Beampointing_heater.tdms" ("string")) -> (w65:string)
      n107 = String To Path(string=w65) -> (path=w64:path)
      n108 = Build Path(base path=w37, name or relative path=w64) -> (appended path=w67:path)
      n109 = call <vilib>:"Add State(s) to Queue__jki_lib_state_machine.vi"("State(s) in (\"\")"="Macro: Initialize") -> ("States Out"=w116:string)  [unwired: 14 in]
      n110 = Create User Event(user event datatype=T13 {"EventEnum"=enum."new data", "Device name"="Device name"} ("New Event")) -> (user event=w124:refnum<user-event>, error out=w126:errorcluster)  [unwired: 1 in]
      "tcp data event" <- w124
      n111 = while "JKI - String-Based Queued State Machine (Basic) v1.0" {
        shift-right: [w145] -> w70
        shift-left: _ -> [w138]
        shift-right: [w148] -> w98
        shift-left: _ -> [w144]
        shift-right: [w147] -> _
        shift-left: w116 -> [w149]
        tunnel: w74 -> [w142]
        tunnel: w71 -> [w140]
        tunnel: [w140] -> w99
        tunnel: w74 -> [w141]
        tunnel: w67 -> [w136]
        tunnel: w37 -> [w135]
        stop <- w146 stop-if-true
        n112 = Unbundle By Name(w138) -> ("active cams"=w137:string[])
        n113 = call <vilib>:"Parse State Queue__jki_lib_state_machine.vi"("State Queue"=w149, "Error In (no error)"=w144) -> ("Remaining States"=w151:string, "Current State"=w152:string, "Arguments"=w150:string)  [unwired: 11 in]
        "Current State" <- w152
        n114 = case shown="\"Check Move\"" w152 {
          selector: w152 -> [_ _ w464 _ _ _ _ _ _ _ _ _ _ _ _ _ _ _ _ _ _ _ _ _ _ _ _ _ _ _ _ _ _ _ _ _ _ _ _ _ _ _]
          tunnel: w151 -> [w187 w463 w468 w486 w492 w497 w501 w542 w558 w562 w566 w572 w583 w607 w616 w626 w630 w658 w778 w830 w860 w869 w891 w912 w916 w932 w1081 w1230 w1310 w1374 w1449 w1525 w1549 w1564 w1638 w1690 w1700 w1741 w1837 w1863 w1877 w1900]
          tunnel: w150 -> [_ _ _ _ _ _ _ _ _ _ _ w567 w578 _ _ _ _ w636 w731 _ w845 _ _ _ _ w933 _ w1209 w1296 w1360 w1428 w1519 _ _ _ _ _ _ _ _ w1881 _]
          tunnel: w138 -> [w185 w460 w466 w476 w489 w495 w498 _ w553 w559 w564 w570 w577 w604 w613 w618 w627 w652 w768 w828 w841 w865 w883 w905 w913 w921 w1060 w1203 w1306 w1370 w1426 w1521 w1546 w1561 w1634 w1687 w1697 w1715 w1835 w1860 w1880 w1891]
          tunnel: [w184 w461 w470 w484 errorcluster {"status"=FALSE, "code"=0, "source"=""} ("error out") w494 w499 w509 w555 w560 w563 w568 w580 w605 w614 w624 w628 w654 w734 w819 w849 w867 w889 w910 w914 w966 w1094 w1228 w1308 w1372 w1447 w1514 w1547 w1562 w1635 w1688 w1698 w1702 w1799 w1861 w1875 w1898] -> w148
          tunnel: w144 -> [w183 w461 w469 w484 w488 w494 w499 w510 w556 w560 w563 w569 w581 w605 w614 w624 w628 w655 w732 w820 w848 w867 w889 w910 w914 w966 w1094 w1228 w1308 w1372 w1447 w1515 w1547 w1562 w1636 w1688 w1698 w1704 w1833 w1861 w1875 w1898]
          tunnel: [w186 w462 w467 w485 w491 w496 w500 w541 w557 w561 w565 w571 w582 w606 w615 w625 w629 w646 w777 w829 w859 w868 w890 w911 w915 w937 w1095 w1229 w1309 w1373 w1448 w1524 w1548 w1563 w1637 w1689 w1699 w1740 w1836 w1862 w1876 w1899] -> w147
          tunnel: [_ _ _ _ _ TRUE _ _ _ _ _ _ _ _ _ _ _ _ _ _ _ _ _ _ _ _ _ _ _ _ _ _ _ _ _ _ _ _ _ _ _ _] -> w146
          tunnel: [w180 w460 w466 w475 w489 w495 w498 w511 w553 w559 w564 w570 w577 w604 w613 w618 w627 w657 w767 w828 w854 w864 w882 w904 w913 w959 w1062 w1203 w1306 w1370 w1426 w1523 w1546 w1561 w1634 w1686 w1697 w1715 w1834 w1860 w1879 w1890] -> w145
          tunnel: "update speed [ms]" -> [w182 _ _ _ _ _ _ _ _ _ _ _ _ _ _ _ _ _ _ _ _ _ _ _ _ _ _ _ _ _ _ _ _ _ _ _ _ _ _ _ _ _]
          tunnel: w142 -> [w179 _ _ _ _ _ _ _ _ _ _ _ _ _ _ _ _ _ _ _ _ _ _ _ _ w957 _ _ _ _ _ _ _ _ _ _ _ _ _ w1845 _ _]
          tunnel: w140 -> [w181 _ _ _ _ _ _ w506 _ _ _ _ _ _ _ _ _ w639 w766 _ w855 _ _ _ _ w925 w1061 w1227 _ _ w1446 w1520 _ w1551 _ _ _ w1714 _ _ _ _]
          tunnel: w136 -> [_ _ _ _ _ _ _ w508 _ _ _ _ _ _ _ _ _ w656 _ _ _ _ _ _ _ _ _ _ _ _ _ _ _ _ _ _ _ _ _ _ _ _]
          tunnel: w135 -> [_ _ _ _ _ _ _ _ _ _ _ _ _ _ _ _ _ _ _ _ _ _ _ _ _ _ _ _ _ _ _ _ _ _ _ _ _ _ w1805 _ _ _]
          frame "", "Idle" {
            # "executes when the state queue is empty"
            n115 = event shown="[1] \"Tab Control 2\": Value Change" {
              selector: _ -> [_ _ _ _ _ _ _ _ _ _ _ _ _ _ _ _ _ _ _ _]
              dyn-events: _ -> [_ _ _ _ _ _ _ _ _ _ _ _ _ _ _ _ _ _ _ _]
              timeout: w182 -> [_ _ _ _ _ _ _ _ _ _ _ _ _ _ _ _ _ _ _ _]
              tunnel: w187 -> [w190 w314 w321 w336 w355 w360 w365 w370 w376 w381 w391 w396 w405 w417 w429 w434 w439 w445 w449 w459]
              tunnel: [w217 w313 w320 w335 w354 w359 w364 w369 w375 w380 w390 w395 w404 w416 w428 w433 w438 w444 w447 w458] -> w186
              tunnel: w185 -> [w213 w316 w318 w332 w351 w357 w362 w367 w373 w378 w388 w393 w398 w415 w427 w432 w437 w443 w450 w456]
              tunnel: [w228 w312 w319 w334 w353 w358 w363 w368 w374 w379 w389 w394 w403 w410 w422 w431 w436 w442 w446 w457] -> w184
              tunnel: w183 -> [w204 w312 w319 w334 w353 w358 w363 w368 w374 w379 w389 w394 w403 w411 w423 w431 w436 w442 w446 w457]
              tunnel: [w216 w316 w318 w332 w350 w357 w362 w367 w373 w378 w388 w393 w398 w415 w427 w432 w437 w443 w450 w456] -> w180
              tunnel: w181 -> [w209 _ _ w328 _ _ _ _ _ _ _ _ _ _ _ _ _ _ _ _]
              tunnel: w179 -> [_ _ _ w330 _ _ _ _ _ _ _ _ _ _ _ _ _ _ _ _]
              event Timeout {
                n116 = event-data() -> ()  [unwired: 1 in, 1 out]
                n117 = Unbundle By Name(w213) -> ("Centroid X"=w210:dbl[][], "Centroid Y"=w207:dbl[][], "Size"=w205:dbl[][], "detection para"=w200:T3[], "active cams"=w208:string[], "thresholds"=w206:cluster{"Lower value":sgl, "Upper value":sgl}[])
                n118 = Unbundle By Name(w213) -> ("img to avg"=w188:i32, "active ccd"=w212:i32)
                n119 = for {
                  tunnel: w208 -> [w249] mode=indexing
                  tunnel: [w250] -> w195 mode=indexing
                  tunnel: w209 -> [w272]
                  tunnel: w200 -> [w270]
                  tunnel: [w233] -> w194 mode=indexing
                  tunnel: [w268] -> w203 mode=indexing
                  tunnel: [w266] -> w211 mode=indexing
                  tunnel: "autodetect" -> [w260]
                  tunnel: w204 -> [w273]
                  tunnel: [w274] -> w202
                  shift-right: [w257] -> w199
                  shift-left: w206 -> [w259]
                  shift-right: [w244] -> w198
                  shift-left: w210 -> [w246]
                  shift-right: [w240] -> w197
                  shift-left: w207 -> [w242]
                  shift-right: [w234] -> w196
                  shift-left: w205 -> [w236]
                  w238 = 0 ("index")
                  n120 = call-poly <userlib>:"Filter 1D Array__ogtk.vi"("items to filter"=w249, "array"=w272) -> ("filtered item indices"=w271:i32[])  [unwired: 4 in, 1 out]
                  n121 = Index Array(array=w271) -> (element=w235:i32)  [unwired: 1 in]
                  n122 = Index Array(array=w236, index (row)=w235) -> (element=w264:dbl[])  [unwired: 1 in]
                  n123 = Index Array(array=w242, index (row)=w235) -> (element=w265:dbl[])  [unwired: 1 in]
                  n124 = Index Array(array=w259, index=w235) -> (element=w263:cluster{"Lower value":sgl, "Upper value":sgl})
                  n125 = Index Array(array=w246, index (row)=w235) -> (element=w248:dbl[])  [unwired: 1 in]
                  n126 = Index Array(array=w270, index=w235) -> (element=w267:T3)
                  n127 = call "CENTRIOD DETECTION.vi"("Refnum in"=w249, "auto threshold"=w260, "Threshold Range In"=w263, "beam detection para"=w267, "error in (no error)"=w273) -> ("Bounding Rect"=w266:T36, "Particle Reports (Pixels)"=w268:T1, "Threshold Range Out"=w258:cluster{"Lower value":sgl, "Upper value":sgl}, "Centriod"=w275:cluster{"X":dbl, "Y":dbl}, "error out"=w274:errorcluster)  [unwired: 7 in, 3 out]
                  n128 = Unbundle By Name(w275) -> ("X"=w247:dbl, "Y"=w243:dbl)
                  n129 = Empty Array?(array=w268) -> (empty?=w269:bool)
                  n130 = Not(x=w269) -> (.not. x?=w233:bool)
                  n131 = Replace Array Subset(array=w259, new element=w258, index=w235) -> (w257:cluster{"Lower value":sgl, "Upper value":sgl}[])
                  n132 = Unbundle By Name(w266) -> ("Right"=w256:dbl, "Left"=w255:dbl, "Bottom"=w254:dbl, "Top"=w253:dbl)
                  n133 = Subtract(x=w256, y=w255) -> (x-y=w251:dbl)
                  n134 = Subtract(x=w254, y=w253) -> (x-y=w252:dbl)
                  n135 = Multiply(x=w251, y=w252) -> (x*y=w239:dbl)
                  n136 = Insert Into Array(array=w265, index=w238, new element=w243) -> (w241:dbl[])
                  n137 = Insert Into Array(array=w248, index=w238, new element=w247) -> (w245:dbl[])
                  n138 = Insert Into Array(array=w264, index=w238, new element=w239) -> (w237:dbl[])
                  n139 = for {
                    shift-right: [w276] -> w261
                    shift-left: dbl[] [] ("Array 4") -> [w279]
                    tunnel: w241 -> [w277] mode=indexing
                    n140 = Equal To 0?(x=w277) -> (x = 0?=w278:bool)
                    n141 = case shown="False" w278 {
                      tunnel: w279 -> [w282 w283]
                      tunnel: w277 -> [w281 _]
                      tunnel: [w280 w283] -> w276
                      frame False {
                        n142 = Build Array (concatenate)(w282, w281) -> (w280:dbl[])
                      }
                      frame True {
                      }
                    }
                  }
                  n143 = Replace Array Subset(array=w246, new element=w245, index (row)=w235) -> (w244:dbl[][])  [unwired: 1 in]
                  n144 = Replace Array Subset(array=w242, new element=w241, index (row)=w235) -> (w240:dbl[][])  [unwired: 1 in]
                  n145 = Replace Array Subset(array=w236, new element=w237, index (row)=w235) -> (w234:dbl[][])  [unwired: 1 in]
                  n146 = Array Size(array=w261) -> (size(s)=w250:i32)
                }
                "detected" <- w194
                "Box" <- w211
                n147 = Bundle(0, 1, "Centroid X"=w210) -> (→"Status":cluster{i32, i32, "Centroid X":dbl[][]})  [unwired: 1 in]
                n148 = Index Array(array=w203, index (row)=w212) -> (element=→"particles":T1)  [unwired: 1 in]
                n149 = call <vilib>:"Clear Errors.vi"("error in (no error)"=w202) -> ("error out"=w228:errorcluster)  [unwired: 5 in, 1 out]
                n150 = local read "Numeric"() -> (w221:dbl)
                n151 = Increment(x=w188) -> (x+1=w218:i32)
                n152 = Greater Or Equal?(x=w221, y=w218) -> (x >= y?=w215:bool)
                n153 = Increment(x=w221) -> (x+1=w220:dbl)
                n154 = Select(t=0.0, s=w215, f=w220) -> (s? t:f=w219:dbl)
                n155 = local write "Numeric"(w219) -> ()
                n156 = Bundle By Name(cluster=w213, "thresholds"=w199) -> (w224:T37)
                n157 = for {
                  tunnel: w195 -> [w305] mode=indexing
                  tunnel: w208 -> [w311] mode=indexing
                  shift-right: [w306] -> w229
                  shift-left: "" ("GUIdevice 7") -> [w309]
                  tunnel: [w300] -> w231 mode=indexing
                  tunnel: "Detection Rate" -> [w304]
                  tunnel: w219 -> [w302]
                  tunnel: w188 -> [w298]
                  n158 = Greater Or Equal?(x=w305, y=w298) -> (x >= y?=w301:bool)
                  n159 = Multiply(x=w304, y=w302) -> (x*y=w303:dbl)
                  n160 = Greater Or Equal?(x=w305, y=w303) -> (x >= y?=w299:bool)
                  n161 = And(x=w301, y=w299) -> (x .and. y?=w300:bool)
                  n162 = Select(t=w311, s=w300, f="") -> (s? t:f=w307:string)
                  n163 = Concatenate Strings(w309, "\t", w307) -> (w306:string)
                }
                n164 = call <vilib>:"Add State(s) to Queue__jki_lib_state_machine.vi"("State(s) in (\"\")"=w190, "State(s) at Back (\"\")"="Device Ini" ("State(s) at Back (\"\")")) -> ("States Out"=w189:string)  [unwired: 13 in]
                n165 = Bundle By Name(cluster=w224, "Centroid X"=w198, "Centroid Y"=w197, "Size"=w196) -> (w193:T37)
                n166 = Unbundle By Name(w193) -> ("img to avg"=w192:i32)
                n167 = case shown="True" w215 {
                  tunnel: w193 -> [w284 w291]
                  tunnel: [w284 w290] -> w216
                  tunnel: w192 -> [_ w286]
                  frame False {
                  }
                  frame True {
                    n168 = Decrement(x=w286) -> (x-1=w289:i32)
                    n169 = Initialize Array(0.0 ("element"), 12 ("dimension size"), w289) -> (w285:dbl[][])
                    n170 = Bundle By Name(cluster=w291, "Centroid X"=w285, "Centroid Y"=w285, "Size"=w285) -> (w290:T37)
                  }
                }
                n171 = Or Array Elements(Boolean array=w231) -> (logical OR=w230:bool)
                n172 = case shown="True" w230 {
                  tunnel: w229 -> [_ w296]
                  tunnel: w189 -> [w292 w294]
                  tunnel: [w292 w293] -> w217
                  frame False {
                  }
                  frame True {
                    n173 = call <vilib>:"Build State String with Arguments__jki_lib_state_machine.vi"("Arguments (\"\")"=w296, "State"="detected") -> ("State with Arguments"=w295:string)  [unwired: 4 in]
                    n174 = call <vilib>:"Add State(s) to Queue__jki_lib_state_machine.vi"("State(s) in (\"\")"=w294, "State(s) at Back (\"\")"=w295) -> ("States Out"=w293:string)  [unwired: 13 in]
                  }
                }
              }
              event "Tab Control 2": Value Change {
                n175 = event-data() -> ()  [unwired: 1 in, 6 out]
                n176 = call <vilib>:"Add State(s) to Queue__jki_lib_state_machine.vi"("State(s) in Front (\"\")"=w314, "State(s) at Back (\"\")"="stats" ("State")) -> ("States Out"=w313:string)  [unwired: 13 in]
              }
              event "stop": Value Change {
                # "Exit Button Value Change (pressed) Event\n(this executes Macro: Exit to terminate the VI)"
                n177 = event-data() -> ()  [unwired: 1 in, 6 out]
                n178 = call <vilib>:"Add State(s) to Queue__jki_lib_state_machine.vi"("State(s) in Front (\"\")"="Macro: Exit", "State(s) in (\"\")"=w321) -> ("States Out"=w320:string)  [unwired: 13 in]
              }
              event Value Change {
                n179 = event-data() -> ()  [unwired: 1 in, 6 out]
                n180 = property on="Set Centriod Target" class="Bool (strict)"("Value"=FALSE) -> ()  [unwired: 2 in, 2 out]
                n181 = Unbundle By Name(w332) -> ("active ccd"=w324:i32, "Centroid X"=w323:dbl[][], "Centroid Y"=w322:dbl[][])
                n182 = Index Array(array=w328, index=w324) -> (element=w327:string)
                n183 = Concatenate Strings("Do want to update the target of " ("message"), w327, "?" ("string")) -> (w325:string)
                n184 = Two Button Dialog(message=w325) -> (T button?=w331:bool)  [unwired: 2 in]
                n185 = case shown="True" w331 {
                  tunnel: w330 -> [_ w343]
                  tunnel: w324 -> [_ w342]
                  tunnel: w323 -> [_ w349]
                  tunnel: w322 -> [_ w344]
                  frame False {
                  }
                  frame True {
                    n186 = Index Array(array=w349, index (row)=w342) -> (element=w348:dbl[])  [unwired: 1 in]
                    n187 = Index Array(array=w344, index (row)=w342) -> (element=w345:dbl[])  [unwired: 1 in]
                    n188 = Index Array(array=w343, index=w342) -> (element=w341:T31)
                    n189 = Unbundle By Name(w341) -> ("Target.X::12"=w340:refnum<vi>, "Target.Y::12"=w338:refnum<vi>)
                    n190 = Reverse 1D Array(array=w348) -> (reversed array=w347:dbl[])
                    n191 = Reverse 1D Array(array=w345) -> (reversed array=w346:dbl[])
                    n192 = Index Array(array=w347) -> (element=w339:dbl)  [unwired: 1 in]
                    n193 = Index Array(array=w346) -> (element=w337:dbl)  [unwired: 1 in]
                    n194 = property class="DigNum (strict)"(reference=w340, "Val(Sgnl)"=w339) -> ()  [unwired: 1 in, 2 out]
                    n195 = property class="DigNum (strict)"(reference=w338, "Val(Sgnl)"=w337) -> ()  [unwired: 1 in, 2 out]
                  }
                }
                n196 = call <vilib>:"Add State(s) to Queue__jki_lib_state_machine.vi"("State(s) in (\"\")"=w336) -> ("States Out"=w335:string)  [unwired: 14 in]
              }
              event "Feedback Global": Value Change {
                # "Exit Button Value Change (pressed) Event\n(this executes Macro: Exit to terminate the VI)"
                n197 = event-data() -> ("NewVal"=w352:bool)  [unwired: 1 in, 5 out]
                n198 = call <vilib>:"Add State(s) to Queue__jki_lib_state_machine.vi"("State(s) in (\"\")"=w355) -> ("States Out"=w354:string)  [unwired: 14 in]
                n199 = Bundle By Name(cluster=w351, "Feedback global"=w352) -> (w350:T37)
              }
              event Value Change {
                n200 = event-data() -> ()  [unwired: 1 in, 6 out]
                n201 = call <vilib>:"Add State(s) to Queue__jki_lib_state_machine.vi"("State(s) in Front (\"\")"="Move Config", "State(s) in (\"\")"=w360) -> ("States Out"=w359:string)  [unwired: 13 in]
              }
              event Value Change {
                n202 = event-data() -> ()  [unwired: 1 in, 6 out]
                n203 = call <vilib>:"Add State(s) to Queue__jki_lib_state_machine.vi"("State(s) in Front (\"\")"="Detection Config", "State(s) in (\"\")"=w365) -> ("States Out"=w364:string)  [unwired: 13 in]
              }
              event "associated motors": Value Change {
                n204 = event-data() -> ()  [unwired: 1 in, 6 out]
                n205 = call <vilib>:"Add State(s) to Queue__jki_lib_state_machine.vi"("State(s) in (\"\")"=w370, "State(s) at Back (\"\")"="Motor Config" ("State(s) at Back (\"\")")) -> ("States Out"=w369:string)  [unwired: 13 in]
              }
              event "Reset History": Value Change {
                n206 = event-data() -> ()  [unwired: 1 in, 6 out]
                n207 = call <vilib>:"Add State(s) to Queue__jki_lib_state_machine.vi"("State(s) in (\"\")"=w376, "State(s) at Back (\"\")"="Reset History" ("State(s) at Back (\"\")")) -> ("States Out"=w375:string)  [unwired: 13 in]
                n208 = property on="Reset History" class="Bool (strict)"("Value"=FALSE ("Reset History")) -> ()  [unwired: 2 in, 2 out]
              }
              event "Save Config": Value Change {
                n209 = event-data() -> ()  [unwired: 1 in, 6 out]
                n210 = call <vilib>:"Add State(s) to Queue__jki_lib_state_machine.vi"("State(s) in (\"\")"=w381, "State(s) at Back (\"\")"="Save Config" ("State(s) at Back (\"\")")) -> ("States Out"=w380:string)  [unwired: 13 in]
              }
              event "Load Config": Value Change {
                n211 = event-data() -> ()  [unwired: 1 in, 6 out]
                n212 = call "File Dialog2"("pattern (all files)"="*.cfg", "pattern label"="config") -> ("selected path"=w385:path)  [unwired: 10 in, 3 out]
                n213 = Path To String(path=w385) -> (string=w383:string)
                "config path" <- w383
                n214 = call <vilib>:"Build State String with Arguments__jki_lib_state_machine.vi"("Arguments (\"\")"=w383, "State"="Load Config" ("State(s) at Back (\"\")")) -> ("State with Arguments"=w382:string)  [unwired: 4 in]
                n215 = call <vilib>:"Add State(s) to Queue__jki_lib_state_machine.vi"("State(s) in (\"\")"=w391, "State(s) at Back (\"\")"=w382) -> ("States Out"=w390:string)  [unwired: 13 in]
              }
              event "Save Stats": Value Change {
                n216 = event-data() -> ()  [unwired: 1 in, 6 out]
                n217 = call <vilib>:"Add State(s) to Queue__jki_lib_state_machine.vi"("State(s) in (\"\")"=w396, "State(s) at Back (\"\")"="Save Stats" ("State(s) at Back (\"\")")) -> ("States Out"=w395:string)  [unwired: 13 in]
              }
              event "active CCDs": Value Change {
                n218 = event-data() -> ("NewVal"=w402:i32)  [unwired: 1 in, 5 out]
                n219 = Unbundle By Name(w398) -> ("active cams"=w397:string[])
                n220 = Index Array(array=w397, index=w402) -> (element=w400:string)
                n221 = call <vilib>:"Build State String with Arguments__jki_lib_state_machine.vi"("Arguments (\"\")"=w400, "State"="active" ("State(s) at Back (\"\")")) -> ("State with Arguments"=w399:string)  [unwired: 4 in]
                n222 = call <vilib>:"Add State(s) to Queue__jki_lib_state_machine.vi"("State(s) in (\"\")"=w405, "State(s) at Back (\"\")"=w399) -> ("States Out"=w404:string)  [unwired: 13 in]
              }
              event "Left", "Right": Value Change {
                n223 = event-data() -> ("CtlRef"=w414:refnum<vi>)  [unwired: 1 in, 5 out]
                n224 = property class="Bool (strict)"(reference=w414, error in=w411) -> (reference out=w413:refnum<vi>, error out=w412:errorcluster, "Label.Text"=w408:string)
                n225 = property class="Bool (strict)"(reference=w413, error in=w412, "Value"=FALSE) -> (error out=w410:errorcluster)  [unwired: 1 out]
                n226 = call <vilib>:"Build State String with Arguments__jki_lib_state_machine.vi"("Arguments (\"\")"=w408, "State"="ManMove X") -> ("State with Arguments"=w407:string)  [unwired: 4 in]
                n227 = call <vilib>:"Add State(s) to Queue__jki_lib_state_machine.vi"("State(s) in (\"\")"=w417, "State(s) at Back (\"\")"=w407) -> ("States Out"=w416:string)  [unwired: 13 in]
              }
              event "Up", "Down": Value Change {
                n228 = event-data() -> ("CtlRef"=w426:refnum<vi>)  [unwired: 1 in, 5 out]
                n229 = property class="Bool (strict)"(reference=w426, error in=w423) -> (reference out=w425:refnum<vi>, error out=w424:errorcluster, "Label.Text"=w420:string)
                n230 = property class="Bool (strict)"(reference=w425, error in=w424, "Value"=FALSE) -> (error out=w422:errorcluster)  [unwired: 1 out]
                n231 = call <vilib>:"Build State String with Arguments__jki_lib_state_machine.vi"("Arguments (\"\")"=w420, "State"="ManMove Y") -> ("State with Arguments"=w419:string)  [unwired: 4 in]
                n232 = call <vilib>:"Add State(s) to Queue__jki_lib_state_machine.vi"("State(s) in (\"\")"=w429, "State(s) at Back (\"\")"=w419) -> ("States Out"=w428:string)  [unwired: 13 in]
              }
              event "Center": Value Change {
                n233 = event-data() -> ()  [unwired: 1 in, 6 out]
                n234 = call <vilib>:"Add State(s) to Queue__jki_lib_state_machine.vi"("State(s) in (\"\")"=w434, "State(s) at Back (\"\")"="Center" ("State(s) at Back (\"\")")) -> ("States Out"=w433:string)  [unwired: 13 in]
              }
              event "new tdms": Value Change {
                n235 = event-data() -> ()  [unwired: 1 in, 6 out]
                n236 = call <vilib>:"Add State(s) to Queue__jki_lib_state_machine.vi"("State(s) in (\"\")"=w439, "State(s) at Back (\"\")"="newtdms" ("State(s) at Back (\"\")")) -> ("States Out"=w438:string)  [unwired: 13 in]
              }
              event "device ini": Value Change {
                n237 = event-data() -> ()  [unwired: 1 in, 6 out]
                n238 = property on="device ini" class="Bool (strict)"("Value"=FALSE ("test")) -> ()  [unwired: 2 in, 2 out]
                n239 = call <vilib>:"Add State(s) to Queue__jki_lib_state_machine.vi"("State(s) in (\"\")"=w445, "State(s) at Back (\"\")"="Device Ini" ("State(s) at Back (\"\")")) -> ("States Out"=w444:string)  [unwired: 13 in]
              }
              event "img to avg": Value Change {
                n240 = event-data() -> ("NewVal"=w451:i32)  [unwired: 1 in, 5 out]
                n241 = Number To Decimal String(number=w451) -> (decimal integer string=w453:string)  [unwired: 1 in]
                n242 = call <vilib>:"Build State String with Arguments__jki_lib_state_machine.vi"("Arguments (\"\")"=w453, "State"="ImgToAvg" ("State(s) at Back (\"\")")) -> ("State with Arguments"=w448:string)  [unwired: 4 in]
                n243 = call <vilib>:"Add State(s) to Queue__jki_lib_state_machine.vi"("State(s) in (\"\")"=w449, "State(s) at Back (\"\")"=w448) -> ("States Out"=w447:string)  [unwired: 13 in]
              }
              event Panel Close? {
                # "Discard the event because we'll close the front panel ourselves in Macro: Exit"
                # "Close Panel button (pressed) Event\n(this executes Macro: Exit to terminate the VI)"
                n244 = event-data() -> ()  [unwired: 1 in, 1 out]
                n245 = call <vilib>:"Add State(s) to Queue__jki_lib_state_machine.vi"("State(s) in Front (\"\")"="Macro: Exit", "State(s) in (\"\")"=w459) -> ("States Out"=w458:string)  [unwired: 13 in]
                n246 = event-data("Discard?"=TRUE) -> ()  [unwired: 1 in, 1 out]
              }
            }
          }
          frame "---------- Core ----------" {
            # "Do not put any code in this frame.\n(it is a separator no-op)"
            n247 = call <vilib>:"Add State(s) to Queue__jki_lib_state_machine.vi"("State(s) in (\"\")"=w463) -> ("States Out"=w462:string)  [unwired: 14 in]
          }
          frame Default {
            w473 = 42 items=["No error", "Argument error", "Memory is full", "Out of zone", "End of file", "File already open", "Generic file I/O error", "File not found", "File permission error", "Disk is full", "Duplicate path", "Too many files open", "System feature not enabled", "Resource file not found", "Cannot add resource", "Resource not found", "Image not found", "Image memory error", "Pen does not exist", "Config type invalid", "Config token not found", "Config parse error", "Config memory error", "Bad external code format", "Bad external code offset", "External code not present", "Null window", "Destroy window error", "Null menu", "Print aborted", "Bad print record", "Print driver error", "Windows error during printing", "Memory error during printing", "Print dialog error", "Generic print error", "Invalid device refnum", "Device not found", "Device parameter error", "Device unit error", "Cannot open device", "Device call aborted", "Generic error", "Cancelled by user", "Object ID too low", "Object ID too high", "Object not in heap", "Unknown heap", "Unknown object (invalid DefProc)", "Unknown object (DefProc not in table)", "Message out of range", "Invalid (null) method", "Unknown message", "Manager call not supported", "Bad address", "Network operation in progress", "Network operation timed out", "Connection is busy", "Network attribute not supported", "Network error", "Address in use", "System out of memory", "Connection aborted", "Connection refused", "Not connected", "Already connected", "Connection closed", "Initialization error (interapplication manager)", "Bad occurrence", "Wait on unbound occurrence handler", "Occurrence queue overflow", "Datalog type conflict", "Unused", "Unrecognized type (interapplication manager)", "Memory corrupt", "Failed to make temporary DLL", "Old CIN version", "Drag socket not found", "Failed to load drop-object", "Failed to register OLE object", "Failed to release OLE object", "Format specifier type mismatch", "Unknown format specifier", "Too few format specifiers", "Too many format specifiers", "Scan failed", "Newer CIN version", "Error converting to variant", "Runtime menu error", "Password tampered", "Variant attribute not found", "Incompatible variant data type", "Event data is not available", "Event Store is not present", "Occurrence is not found", "Event Queue is not created", "Event info is not available", "Refnum passed is NULL", "Error retrieving Class GUID", "Error retrieving CoClass GUID", "Error retrieving TypeLib GUID.", "Bad built application magic bytes.", "Specific driver is different from the specific driver associated with the Logical Name.", "There is no session opened to the class driver.", "Max Error", "MAX - Error with config objects", "MAX - Error loading configuration", "MAX - Group not supported"]
            # "Current State"
            # "Do not delete, rename, or modify this frame.\n(this is used to capture unhandled states and typos)"
            # "Handle mistyped state name (developer tool)"
            n248 = Format Into String(format string="Software Exception: Unhandled State \"%s\"." ("message"), error in=w469, w464) -> (resulting string=w472:string, error out=w471:errorcluster)  [unwired: 1 in]
            n249 = call <vilib>:"Error Cluster From Error Code.vi"("show call chain? (False)"=TRUE, "error in (no error)"=w471, "error message (\"\")"=w472, "error code (0)"=w473) -> ("error out"=w470:errorcluster)  [unwired: 5 in]
            n250 = call <vilib>:"Add State(s) to Queue__jki_lib_state_machine.vi"("State(s) in (\"\")"=w468) -> ("States Out"=w467:string)  [unwired: 14 in]
          }
          frame "Initialize Core Data" {
            # "Do not delete, rename, or modify this frame.\n(this is used to determine panel behavior on exit)"
            # "originally closed?"
            # "exe?"
            # "If panel starts closed or is an EXE, then close it when we exit"
            n251 = property class="VI"() -> ("Front Panel.Open"=w483:bool)  [unwired: 2 in, 2 out]
            n252 = property class="App"() -> ("App.Kind"=w482:T16)  [unwired: 2 in, 2 out]
            n253 = control-ref of="Current VI Reference"() -> (w477:refnum<vi>)
            n254 = Not(x=w483) -> (.not. x?=w480:bool)
            n255 = Equal?(x=w482, y=T16."Run Time System" ("Application:Kind")) -> (x = y?=w479:bool)
            n256 = Or(x=w480, y=w479) -> (x .or. y?=w478:bool)
            n257 = Bundle By Name(cluster=w476, "Core.Current VI Reference"=w477, "Core.Close Panel on Exit?"=w478) -> (w475:T37)
            n258 = call <vilib>:"Add State(s) to Queue__jki_lib_state_machine.vi"("State(s) in (\"\")"=w486) -> ("States Out"=w485:string)  [unwired: 14 in]
          }
          frame "Error Handler" {
            # "Unhandled Error -- Display it"
            # "Handle any errors here.\nYou can also output any states to clean-up after errors occur"
            # "Clear error"
            n259 = call <vilib>:"General Error Handler.vi"("error in (no error)"=w488) -> ()  [unwired: 10 in, 5 out]
            n260 = call <vilib>:"Add State(s) to Queue__jki_lib_state_machine.vi"("State(s) in Front (\"\")"="/* Post Error States", "State(s) in (\"\")"=w492) -> ("States Out"=w491:string)  [unwired: 13 in]
          }
          frame "Exit" {
            # "Do not put any code in this frame.\n(No errors that occur here will be handled.)"
            n261 = call <vilib>:"Add State(s) to Queue__jki_lib_state_machine.vi"("State(s) in (\"\")"=w497) -> ("States Out"=w496:string)  [unwired: 14 in]
          }
          frame "---------- Data ----------" {
            # "Do not put any code in this frame.\n(It is a separator no-op. You can make a copy of this frame to create a new Data frame)"
            n262 = call <vilib>:"Add State(s) to Queue__jki_lib_state_machine.vi"("State(s) in (\"\")"=w501) -> ("States Out"=w500:string)  [unwired: 14 in]
          }
          frame "Data: Initialize" {
            w502 = dbl[] [0.0, 0.0, 0.0, 0.0, 0.0, 0.0, 0.0, 0.0, 0.0, 0.0, 0.0, 0.0]  # steps speed Y
            w503 = dbl[] [0.0, 0.0, 0.0, 0.0, 0.0, 0.0, 0.0, 0.0, 0.0, 0.0, 0.0, 0.0]  # steps speed X
            w507 = bool[] [FALSE, FALSE, FALSE, FALSE, TRUE, TRUE, TRUE, FALSE, FALSE, FALSE, FALSE, FALSE]  # detected
            w517 = bool[] [FALSE, FALSE, FALSE, FALSE, FALSE, FALSE, FALSE, FALSE, FALSE, FALSE, FALSE, TRUE]  # speedmode Y
            w518 = bool[] [FALSE, FALSE, FALSE, FALSE, FALSE, FALSE, FALSE, FALSE, FALSE, FALSE, FALSE, TRUE]  # speedmode X
            w520 = cluster{"Lower value":sgl, "Upper value":sgl}[] [{"Lower value"=93.0, "Upper value"=255.0}, {"Lower value"=105.0, "Upper value"=255.0}, {"Lower value"=0.0, "Upper value"=255.0}, {"Lower value"=127.0, "Upper value"=255.0}, {"Lower value"=0.0, "Upper value"=255.0}, {"Lower value"=0.0, "Upper value"=255.0}, {"Lower value"=0.0, "Upper value"=255.0}, {"Lower value"=0.0, "Upper value"=255.0}, {"Lower value"=0.0, "Upper value"=255.0}, {"Lower value"=0.0, "Upper value"=255.0}, {"Lower value"=0.0, "Upper value"=255.0}, {"Lower value"=0.0, "Upper value"=255.0}]  # thresholds
            w527 = FALSE  # Feedback global
            w529 = 0  # active ccd
            w513 = 6  # img to avg
            w540 = T38 {"Current VI Reference"=refnum, "Close Panel on Exit?"=FALSE}  # Core
            # "Initialize the shift-register data, here.\n(data names are defined by what you wire into the bundle function)"
            n263 = disable-structure shown="Disabled" {
              disable-tunnel: w510 -> [w552 _]
              disable-tunnel: [w551 _] -> w509
              disable-tunnel: w508 -> [w550 _]
              disable-tunnel: [w549 _] -> _
              disable-tunnel: w506 -> [w543 _]
              frame Disabled {
                n264 = TDMS Open(6:FALSE ("disable buffering (T)"), 7:enum16{"1.0", "2.0"}."2.0" ("file format version (2.0)"), 8:w552, 10:T17."create or replace" ("operation"), 11:w550) -> (0:w547:errorcluster, 3:w548:refnum<k34>)  [unwired: 2 in]
                n265 = call "TDMSbuffersize.vi"("error in (no error)"=w547, "group names"=w543, "Data Value Reference in"=w548) -> ("error out"=w551:errorcluster, "Data Value Reference out"=w549:refnum<k34>)  [unwired: 7 in]
              }
              frame Enabled {
              }
            }
            n266 = call <vilib>:"Add State(s) to Queue__jki_lib_state_machine.vi"("State(s) in Front (\"\")"="newtdms" ("State(s) in Front (\"\")"), "State(s) in (\"\")"=w542) -> ("States Out"=w541:string)  [unwired: 13 in]
            n267 = Bundle("Core"=w540, "detection para"="detection para", "thresholds"=w520, "Centroid X"="Centroid X", "Centroid Y"="Centroid Y", "img to avg"=w513, "Mean Centroid X"="Mean Centroid X", "Mean Centroid Y"="Mean Centroid Y", "Offset X"="Offset X", "Offset Y"="Offset Y", "Offset X stats"="Offset X stats", "Offset Y stats"="Offset Y stats", "Size"="Size", "Mean Size"="Mean Size", "Time"="Time", "move properties"="move properties", "active axis refs 2"="active axis refs 2", "active ccd"=w529, "Feedback global"=w527, "Motor X"="Motor X", "Motor Y"="Motor Y", "active cams"="active cams", "Data Value Reference out"=refnum<k34> refnum, "active man refs"="active man refs", "detected"=w507, "speedmode X"=w518, "speedmode Y"=w517, "steps speed X"=w503, "steps speed Y"=w502) -> (w512:T37)  [unwired: 1 in]
            n268 = Initialize Array(0.0 ("element"), 12 ("dimension size"), w513) -> (w516:dbl[][])
            n269 = Bundle By Name(cluster=w512, "Centroid X"=w516, "Centroid Y"=w516, "Size"=w516) -> (w511:T37)
          }
          frame "Data: Cleanup" {
            # "Cleanup any data and references, here.\n(this is called automatically, by the Macro: Exit)"
            n270 = Unbundle By Name(w553) -> ("Core.Current VI Reference"=w554:refnum<vi>)
            n271 = Close Reference(reference=w554, error in (no error)=w556) -> (error out=w555:errorcluster)
            n272 = call <vilib>:"Add State(s) to Queue__jki_lib_state_machine.vi"("State(s) in (\"\")"=w558) -> ("States Out"=w557:string)  [unwired: 14 in]
          }
          frame "---------- UI ----------" {
            # "Do not put any code in this frame.\n(It is a separator no-op. You can make a copy of this frame to create a new UI frame)"
            n273 = call <vilib>:"Add State(s) to Queue__jki_lib_state_machine.vi"("State(s) in (\"\")"=w562) -> ("States Out"=w561:string)  [unwired: 14 in]
          }
          frame "UI: Initialize" {
            # "Initialize the User Interface, here.\n(this is called automatically, by the Macro: Init)"
            n274 = call <vilib>:"Add State(s) to Queue__jki_lib_state_machine.vi"("State(s) in (\"\")"=w566) -> ("States Out"=w565:string)  [unwired: 14 in]
          }
          frame "UI: Cursor Set" {
            # "Argument"
            # "Set and Unset Cursor Busy.\n(Usage: \"UI: Cursor Set >> Busy|Idle\")"
            n275 = case shown="\"Idle\", Default" w567 {
              tunnel: w569 -> [w574 w576]
              tunnel: [w573 w575] -> w568
              frame "Idle", Default {
                n276 = call <vilib>:"Unset Busy.vi"("error in (no error)"=w574) -> ("error out"=w573:errorcluster)  [unwired: 10 in]
              }
              frame "Busy" {
                n277 = call <vilib>:"Set Busy.vi"("error in (no error)"=w576) -> ("error out"=w575:errorcluster)  [unwired: 9 in, 1 out]
              }
            }
            n278 = call <vilib>:"Add State(s) to Queue__jki_lib_state_machine.vi"("State(s) in (\"\")"=w572) -> ("States Out"=w571:string)  [unwired: 14 in]
          }
          frame "UI: Front Panel State" {
            # "Argument"
            # "Set Front Panel Open or Closed\n(Usage: \"UI: Front Panel State >> Open|Close\")"
            n279 = Unbundle By Name(w577) -> ("Core.Current VI Reference"=w579:refnum<vi>)
            n280 = case shown="\"Open\", Default" w578 {
              tunnel: w581 -> [w587 w598]
              tunnel: [w588 w599] -> w580
              tunnel: w579 -> [_ _]
              frame "Open", Default {
                n281 = property class="VI"(error in=w587) -> (reference out=w585:refnum<vi>, error out=w586:errorcluster, "Front Panel.Open"=w584:bool)  [unwired: 1 in]
                n282 = case shown="False" w584 {
                  tunnel: [w591 w594] -> w588
                  tunnel: w586 -> [w590 w594]
                  tunnel: w585 -> [w589 _]
                  frame False {
                    n283 = invoke class="VI" method="FP.Open"(reference=w589, error in=w590, "Activate"=TRUE, "State"=T18."Standard") -> (error out=w591:errorcluster)  [unwired: 1 in, 4 out]
                  }
                  frame True {
                  }
                }
              }
              frame "Close" {
                n284 = property class="VI"(error in=w598) -> (reference out=w596:refnum<vi>, error out=w597:errorcluster, "Front Panel.Open"=w595:bool)  [unwired: 1 in]
                n285 = case shown="True" w595 {
                  tunnel: [w600 w603] -> w599
                  tunnel: w597 -> [w600 w602]
                  tunnel: w596 -> [_ w601]
                  frame False {
                  }
                  frame True {
                    n286 = invoke class="VI" method="FP.Close"(reference=w601, error in=w602) -> (error out=w603:errorcluster)  [unwired: 1 in, 2 out]
                  }
                }
              }
            }
            n287 = call <vilib>:"Add State(s) to Queue__jki_lib_state_machine.vi"("State(s) in (\"\")"=w583) -> ("States Out"=w582:string)  [unwired: 14 in]
          }
          frame "---------- Macro ----------" {
            # "Do not put any code in this frame.\n(It is a separator no-op. You can make a copy of this frame to create a new Macro frame)"
            n288 = call <vilib>:"Add State(s) to Queue__jki_lib_state_machine.vi"("State(s) in (\"\")"=w607) -> ("States Out"=w606:string)  [unwired: 14 in]
          }
          frame "Macro: Initialize" {
            # "Initialization Macro\n(This is called once, when the VI starts)"
            n289 = property on="img to avg" class="DigNum (strict)"() -> ("Value"=w609:i32)  [unwired: 2 in, 2 out]
            n290 = Number To Decimal String(number=w609) -> (decimal integer string=w611:string)  [unwired: 1 in]
            n291 = call <vilib>:"Build State String with Arguments__jki_lib_state_machine.vi"("Arguments (\"\")"=w611, "State"="ImgToAvg") -> ("State with Arguments"=w608:string)  [unwired: 4 in]
            n292 = call <vilib>:"Add State(s) to Queue__jki_lib_state_machine.vi"("State(s) in Front (\"\")"="Data: Initialize\nInitialize Core Data\nUI: Initialize\nUI: Front Panel State >> Open\nDevice Ini >> 3000", "State(s) in (\"\")"=w616, "State(s) at Back (\"\")"=w608) -> ("States Out"=w615:string)  [unwired: 12 in]
          }
          frame "Macro: Exit" {
            # "Exit Macro\n(This is called once, when the VI exits)"
            n293 = Unbundle By Name(w618) -> ("Core.Close Panel on Exit?"=w617:bool)
            n294 = Select(t="UI: Front Panel State >> Close", s=w617, f="") -> (s? t:f=w621:string)
            n295 = call <vilib>:"Add State(s) to Queue__jki_lib_state_machine.vi"("State(s) in (\"\")"=w621, "State(s) at Back (\"\")"="Data: Cleanup\nExit") -> ("States Out"=w619:string)  [unwired: 13 in]
            n296 = call <vilib>:"Add State(s) to Queue__jki_lib_state_machine.vi"("State(s) in Front (\"\")"=w619, "State(s) in (\"\")"=w626) -> ("States Out"=w625:string)  [unwired: 13 in]
          }
          frame "---------- Ini and Configure ----------" {
            # "Template Separator\n(You can make a copy of, or modify, this frame)"
            n297 = call <vilib>:"Add State(s) to Queue__jki_lib_state_machine.vi"("State(s) in (\"\")"=w630) -> ("States Out"=w629:string)  [unwired: 14 in]
          }
          frame "Device Ini" {
            # "Your code here.\n(You can make a copy of, or modify, this frame)"
            n298 = Empty String/Path?(string/path=w636) -> (empty?=w653:bool)
            n299 = flat-sequence {
              tunnel: w639 -> [w660]
              tunnel: [w660] -> w640
              tunnel: w638 -> [w659]
              tunnel: w640 -> [w665]
              tunnel: [w663] -> w637
              frame #0 {
                n300 = Wait (ms)(milliseconds to wait=w659) -> ()  [unwired: 1 out]
              }
              frame #1 {
                n301 = local read "Array 3"() -> (w661:sgl[])
                n302 = disable-structure shown="Disabled" {
                  disable-tunnel: w665 -> [w668 _]
                  disable-tunnel: [w666 _] -> _
                  frame Disabled {
                    n303 = for {
                      tunnel: w668 -> [w669] mode=indexing
                      shift-right: [w671] -> w666
                      shift-left: string[] [] -> [w672]
                      n304 = call "send command.vi"("Device Name"=w669) -> ("status"=w673:bool)  [unwired: 4 in]
                      n305 = Wait (ms)(milliseconds to wait=u32 1) -> ()  [unwired: 1 out]
                      n306 = case shown="True" w673 {
                        tunnel: w672 -> [w674 w677]
                        tunnel: [w674 w676] -> w671
                        tunnel: w669 -> [_ w675]
                        frame False {
                        }
                        frame True {
                          n307 = Build Array (concatenate)(w677, w675) -> (w676:string[])
                        }
                      }
                    }
                  }
                  frame Enabled {
                  }
                }
                n308 = for {
                  tunnel: w665 -> [w680] mode=indexing
                  shift-right: [w685] -> w663
                  shift-left: string[] [] -> [w686]
                  tunnel: [w679] -> w662 mode=indexing
                  shift-right: [w683] -> _
                  shift-left: w661 -> [w683]
                  i -> [w684]
                  n309 = call "IMAQ Histograph"("Image"=w680) -> ("error out"=w678:errorcluster, "Mean Value"=w679:sgl)  [unwired: 7 in, 2 out]
                  n310 = Index Array(array=w683, index=w684) -> (element=w682:sgl)
                  n311 = call <vilib>:"Clear Errors.vi"("error in (no error)"=w678) -> ()  [unwired: 5 in, 2 out]
                  n312 = Equal?(x=w679, y=w682) -> (x = y?=w681:bool)
                  n313 = case shown="False" w681 {
                    tunnel: w686 -> [w689 w690]
                    tunnel: [w688 w690] -> w685
                    tunnel: w680 -> [w687 _]
                    frame False {
                      n314 = Build Array (concatenate)(w689, w687) -> (w688:string[])
                    }
                    frame True {
                    }
                  }
                }
                "Array 3" <- w662
              }
            }
            n315 = case shown="False" w653 {
              tunnel: w636 -> [w725 _]
              tunnel: [w724 0] -> w638
              frame False {
                n316 = Decimal String To Number(string=w725) -> (number=w724:i32)  [unwired: 2 in, 1 out]
              }
              frame True {
              }
            }
            n317 = Equal?(x=w636, y="T") -> (x = y?=w633:bool)
            n318 = Unbundle By Name(w652) -> ("active cams"=w645:string[])
            n319 = call <vilib>:"Add State(s) to Queue__jki_lib_state_machine.vi"("State(s) in (\"\")"=w658) -> ("States Out"=w647:string)  [unwired: 14 in]
            n320 = Equal?(x=w645, y=w637) -> (x = y?=w651:bool[])
            n321 = Empty Array?(array=w645) -> (empty?=w650:bool)
            n322 = Not(x=w650) -> (.not. x?=w649:bool)
            n323 = Build Array (concatenate)(w651, w649) -> (w648:bool[])
            n324 = Array Size(array=w637) -> (size(s)=w644:i32)
            n325 = Array Size(array=w645) -> (size(s)=w643:i32)
            n326 = And Array Elements(Boolean array=w648) -> (logical AND=w641:bool)
            n327 = Equal?(x=w644, y=w643) -> (x = y?=w642:bool)
            n328 = And(x=w642, y=w641) -> (x .and. y?=w634:bool)
            n329 = Not(x=w634) -> (.not. x?=w632:bool)
            n330 = Or(x=w633, y=w632) -> (x .or. y?=w631:bool)
            n331 = case shown="True" w631 {
              tunnel: [w693 w709] -> w657
              tunnel: w656 -> [_ _]
              tunnel: w655 -> [w692 w707]
              tunnel: [w692 w707] -> w654
              tunnel: w652 -> [w693 w703]
              tunnel: w637 -> [_ w704]
              tunnel: w647 -> [w691 _]
              tunnel: [w691 w697] -> w646
              frame False {
              }
              frame True {
                n332 = property on="active CCDs" class="LstBox (strict)"("Item Names"=w704) -> ()  [unwired: 2 in, 2 out]
                n333 = Array Size(array=w704) -> (size(s)=w716:i32)
                n334 = Initialize Array(0.0 ("element"), w716, 0 ("dimension size")) -> (w711:dbl[][])
                n335 = Unbundle By Name(w703) -> ("img to avg"=w702:i32)
                n336 = Bundle By Name(cluster=w703, "active cams"=w704) -> (w710:T37)
                n337 = Initialize Array(0.0 ("element"), 12 ("dimension size"), w702) -> (w701:dbl[][])
                n338 = local write "Numeric"(0.0 ("Numeric")) -> ()
                n339 = Bundle By Name(cluster=w710, "Offset X stats"=w711, "Offset Y stats"=w711, "Centroid X"=w701, "Centroid Y"=w701, "Mean Centroid X"=w711, "Mean Centroid Y"=w711, "Offset X"=w711, "Offset Y"=w711, "Size"=w701, "Mean Size"=w711, "Motor X"=w711, "Motor Y"=w711) -> (w709:T37)
                n340 = for {
                  N: 1 -> [_]
                  shift-right: [w718] -> w714
                  shift-left: timestamp[][] [] ("Time") -> [w720]
                  n341 = for {
                    N: 12 -> [_]
                    tunnel: w720 -> [w723] mode=indexing
                    tunnel: [w721] -> w718 mode=indexing
                    n342 = Get Date/Time In Seconds() -> (seconds since 1Jan1904=w722:timestamp)
                    n343 = Build Array (concatenate)(w723, w722) -> (w721:timestamp[])
                  }
                }
                n344 = property on="config path" class="Str"() -> ("Value"=w699:string)  [unwired: 2 in, 2 out]
                n345 = call <vilib>:"Add State(s) to Queue__jki_lib_state_machine.vi"("State(s) in Front (\"\")"="Move Config\nMotor Config\nDetection Config\nactive\nCenter" ("State(s) in Front (\"\")"), "State(s) in (\"\")"="" ("State(s) in (\"\")")) -> ("States Out"=w698:string)  [unwired: 13 in]
                n346 = call <vilib>:"Build State String with Arguments__jki_lib_state_machine.vi"("Arguments (\"\")"=w699, "State"="Load Config" ("State(s) in Front (\"\")")) -> ("State with Arguments"=w696:string)  [unwired: 4 in]
                n347 = call <vilib>:"Add State(s) to Queue__jki_lib_state_machine.vi"("State(s) in (\"\")"=w698, "State(s) at Back (\"\")"=w696) -> ("States Out"=w697:string)  [unwired: 13 in]
                n348 = property on="Time" class="Arr (strict)"("Value"=w714) -> ()  [unwired: 2 in, 2 out]
                "name array" <- w704
              }
            }
          }
          frame "Load Config" {
            # "Your code here.\n(You can make a copy of, or modify, this frame)"
            n349 = Unbundle By Name(w768) -> ("detection para"=w774:T3[], "move properties"=w771:T2[], "thresholds"=w764:cluster{"Lower value":sgl, "Upper value":sgl}[])
            n350 = Empty String/Path?(string/path=w731) -> (empty?=w730:bool)
            n351 = case shown="False" w730 {
              tunnel: [w784 T5 {"CCDs"=[], "move properties"=[], "detection para"=[], "thresholds"=[], "Value"={"Motor CCD 1"=0, "Motor CCD 2"=0, "Motor CCD 3"=0, "Motor CCD 4"=0, "Motor CCD 5"=0, "Motor CCD 6"=0, "Motor CCD 7"=0, "Motor CCD 8"=0, "Motor CCD 9"=0, "Motor CCD 10"=0, "Motor CCD 11"=0, "Motor CCD 12"=0}} ("output cluster 2")] -> w776
              tunnel: [w782 w791] -> w735
              tunnel: w732 -> [w781 w791]
              tunnel: w731 -> [w780 _]
              frame False {
                n352 = String To Path(string=w780) -> (path=w779:path)
                n353 = Open/Create/Replace File(file path (use dialog)=w779, error in=w781, operation (0:open)=T19."open or create") -> (refnum out=w786:refnum<file>, error out=w787:errorcluster)  [unwired: 3 in, 1 out]
                n354 = Read from Binary File(5:"output cluster 2", 8:w787, 11:w786) -> (0:w788:errorcluster, 2:w784:T5, 3:w789:refnum<file>)  [unwired: 3 in, 1 out]
                n355 = Close File(refnum=w789, error in=w788) -> (error out=w782:errorcluster)  [unwired: 1 out]
              }
              frame True {
              }
            }
            n356 = property on="Load Config" class="Bool (strict)"("Value"=FALSE ("Load Config")) -> ()  [unwired: 2 in, 2 out]
            n357 = Unbundle By Name(w776) -> ("Value"=w762:T7, "CCDs"=w775:string[], "detection para"=w773:T3[], "move properties"=w772:T2[], "thresholds"=w765:cluster{"Lower value":sgl, "Upper value":sgl}[])
            n358 = Cluster To Array(cluster=w762) -> (array=w763:u16[])
            n359 = call <vilib>:"Add State(s) to Queue__jki_lib_state_machine.vi"("State(s) in (\"\")"=w778, "State(s) at Back (\"\")"="Motor Config" ("State(s) at Back (\"\")")) -> ("States Out"=w777:string)  [unwired: 13 in]
            n360 = for {
              tunnel: w775 -> [w807]
              tunnel: w773 -> [w809]
              tunnel: w772 -> [w808]
              shift-right: [w801] -> w770
              shift-left: w774 -> [w806]
              shift-right: [w799] -> w769
              shift-left: w771 -> [w805]
              tunnel: w766 -> [w804] mode=indexing
              tunnel: w765 -> [w800]
              shift-right: [w796] -> w728
              shift-left: w764 -> [w798]
              tunnel: w763 -> [w795]
              tunnel: [w792] -> w761 mode=indexing
              i -> [w793]
              n361 = call-poly <userlib>:"Filter 1D Array__ogtk.vi"("items to filter"=w804, "array"=w807) -> ("filtered item indices"=w810:i32[])  [unwired: 4 in, 1 out]
              n362 = Index Array(array=w810) -> (element=w794:i32)  [unwired: 1 in]
              n363 = Index Array(array=w795, index=w794) -> (element=w792:u16)
              n364 = Index Array(array=w809, index=w794) -> (element=w803:T3)
              n365 = Index Array(array=w808, index=w794) -> (element=w802:T2)
              n366 = Index Array(array=w800, index=w794) -> (element=w797:cluster{"Lower value":sgl, "Upper value":sgl})
              n367 = Replace Array Subset(array=w806, new element=w803, index=w793) -> (w801:T3[])
              n368 = Replace Array Subset(array=w805, new element=w802, index=w793) -> (w799:T2[])
              n369 = Replace Array Subset(array=w798, new element=w797, index=w793) -> (w796:cluster{"Lower value":sgl, "Upper value":sgl}[])
            }
            n370 = Array Size(array=w728) -> (size(s)=→"size(s) 6":i32)
            n371 = Index Array(array=w761, index #1=0 ("index (row)"), index #2=1 ("index (row)"), index #3=2 ("index (row)"), index #4=3 ("index (row)"), index #5=4 ("index (row)"), index #6=5 ("index (row)"), index #7=6 ("index (row)"), index #8=7 ("index (row)"), index #9=8 ("index (row)"), index #10=9 ("index (row)"), index #11=10 ("index (row)"), index #12=11 ("index (row)")) -> (element #1=w748:u16, element #2=w747:u16, element #3=w746:u16, element #4=w745:u16, element #5=w744:u16, element #6=w743:u16, element #7=w742:u16, element #8=w741:u16, element #9=w740:u16, element #10=w739:u16, element #11=w738:u16, element #12=w737:u16)
            n372 = Bundle By Name(cluster=w762, "Motor CCD 1"=w748, "Motor CCD 2"=w747, "Motor CCD 3"=w746, "Motor CCD 4"=w745, "Motor CCD 5"=w744, "Motor CCD 6"=w743, "Motor CCD 7"=w742, "Motor CCD 8"=w741, "Motor CCD 9"=w740, "Motor CCD 10"=w739, "Motor CCD 11"=w738, "Motor CCD 12"=w737) -> (w736:T7)
            n373 = Bundle By Name(cluster=w768, "detection para"=w770, "move properties"=w769, "thresholds"=w728) -> (w767:T37)
            n374 = property on="associated motors" class="Clust (strict)"(error in=w735, "Val(Sgnl)"=w736) -> (error out=w734:errorcluster)  [unwired: 1 in, 1 out]
          }
          frame "Save Config" {
            # "Your code here.\n(You can make a copy of, or modify, this frame)"
            n375 = Unbundle By Name(w828) -> ("move properties"=w814:T2[], "detection para"=w823:T3[], "thresholds"=w811:cluster{"Lower value":sgl, "Upper value":sgl}[])
            n376 = property on="associated motors" class="Clust (strict)"() -> ("Value"=w822:T7)  [unwired: 2 in, 2 out]
            n377 = property on="Save Config" class="Bool (strict)"("Value"=FALSE ("Save Config")) -> ()  [unwired: 2 in, 2 out]
            n378 = local read "CCDs"() -> (w812:string[])
            n379 = call "File Dialog"("pattern (all files)"="*.cfg", "pattern label"="config") -> ("selected path"=w816:path)  [unwired: 10 in, 3 out]
            n380 = Bundle("CCDs"=w812, "move properties"=w814, "detection para"=w823, "thresholds"=w811, "Value"=w822) -> (w815:T5)  [unwired: 1 in]
            n381 = Open/Create/Replace File(file path (use dialog)=w816, error in=w820, operation (0:open)=T19."replace or create with confirmation") -> (refnum out=w824:refnum<file>, error out=w825:errorcluster)  [unwired: 3 in, 1 out]
            n382 = Write to Binary File(file (use dialog)=w824, data=w815, error in=w825) -> (refnum out=w827:refnum<file>, error out=w826:errorcluster)  [unwired: 3 in, 1 out]
            n383 = Close File(refnum=w827, error in=w826) -> (error out=w819:errorcluster)  [unwired: 1 out]
            n384 = call <vilib>:"Add State(s) to Queue__jki_lib_state_machine.vi"("State(s) in (\"\")"=w830) -> ("States Out"=w829:string)  [unwired: 14 in]
          }
          frame "active" {
            # "Your code here.\n(You can make a copy of, or modify, this frame)"
            n385 = Empty String/Path?(string/path=w845) -> (empty?=w844:bool)
            n386 = Unbundle By Name(w841) -> ("move properties"=w857:T2[], "detection para"=w853:T3[])  [unwired: 1 out]
            n387 = Unbundle By Name(w841) -> ("active axis refs 2"=w840:T11)
            n388 = call-poly <userlib>:"Filter 1D Array__ogtk.vi"("items to filter"=w845, "array"=w855) -> ("filtered item indices"=w858:i32[])  [unwired: 4 in, 1 out]
            n389 = Index Array(array=w858) -> (element=w842:i32)  [unwired: 1 in]
            n390 = Select(t=0, s=w844, f=w842) -> (s? t:f=w838:i32)
            n391 = Index Array(array=w840, index=w838) -> (element=w839:cluster{"Ref X":refnum<vi>, "Ref Y":refnum<vi>})
            n392 = Unbundle By Name(w839) -> ("Ref X"=w837:refnum<vi>, "Ref Y"=w836:refnum<vi>)
            n393 = Index Array(array=w857, index=w838) -> (element=w856:T2)
            n394 = Index Array(array=w853, index=w838) -> (element=w852:T3)
            n395 = property on="move config" class="Clust (strict)"(error in=w848, "Value"=w856) -> (error out=w846:errorcluster)  [unwired: 1 in, 1 out]
            n396 = property on="beam detection para" class="Clust (strict)"(error in=w846, "Value"=w852) -> (error out=w847:errorcluster)  [unwired: 1 in, 1 out]
            n397 = call <vilib>:"Add State(s) to Queue__jki_lib_state_machine.vi"("State(s) in (\"\")"=w860) -> ("States Out"=w859:string)  [unwired: 14 in]
            n398 = property class="DigNum (strict)"(reference=w837, error in=w847) -> (error out=w833:errorcluster, "Value"=w835:dbl)  [unwired: 1 out]
            n399 = Bundle By Name(cluster="active Axis ref 3", "Ref X"=w837, "Ref Y"=w836) -> (w850:cluster{"Ref X":refnum<vi>, "Ref Y":refnum<vi>})
            n400 = Bundle By Name(cluster=w841, "active ccd"=w838, "active man refs"=w850) -> (w854:T37)
            n401 = property on="Position 1" class="DigNum (strict)"(error in=w833, "Value"=w835) -> (error out=w832:errorcluster)  [unwired: 1 in, 1 out]
            n402 = property class="DigNum (strict)"(reference=w836, error in=w832) -> (error out=w831:errorcluster, "Value"=w834:dbl)  [unwired: 1 out]
            n403 = property on="Position 2" class="DigNum (strict)"(error in=w831, "Value"=w834) -> (error out=w849:errorcluster)  [unwired: 1 in, 1 out]
          }
          frame "Detection Config" {
            # "Your code here.\n(You can make a copy of, or modify, this frame)"
            n404 = Unbundle By Name(w865) -> ("detection para"=w861:T3[], "active ccd"=w866:i32)
            n405 = Replace Array Subset(array=w861, new element="beam detection para", index=w866) -> (w862:T3[])
            n406 = Bundle By Name(cluster=w865, "detection para"=w862) -> (w864:T37)
            n407 = call <vilib>:"Add State(s) to Queue__jki_lib_state_machine.vi"("State(s) in (\"\")"=w869) -> ("States Out"=w868:string)  [unwired: 14 in]
          }
          frame "Motor Config" {
            # "Your code here.\n(You can make a copy of, or modify, this frame)"
            n408 = Unbundle By Name("associated motors") -> ("Motor CCD 1"=w886:u16, "Motor CCD 2"=w887:u16, "Motor CCD 3"=w888:u16, "Motor CCD 4"=w881:u16, "Motor CCD 5"=w880:u16, "Motor CCD 6"=w879:u16, "Motor CCD 7"=w878:u16, "Motor CCD 8"=w877:u16, "Motor CCD 9"=w876:u16, "Motor CCD 10"=w875:u16, "Motor CCD 11"=w874:u16, "Motor CCD 12"=w873:u16)
            n409 = Build Array(w886, w887, w888, w881, w880, w879, w878, w877, w876, w875, w874, w873) -> (w872:u16[])
            n410 = local read "motor refs"() -> (w884:refnum<vi>[])
            n411 = Increment(x=w872) -> (x+1=w871:u16[])
            n412 = for {
              tunnel: w871 -> [w903] mode=indexing
              tunnel: w884 -> [w898]
              tunnel: [w892] -> w870 mode=indexing
              n413 = Multiply(x=w903, y=u16 2) -> (x*y=w899:u16)
              n414 = Subtract(x=w899, y=u16 2) -> (x-y=w897:u16)
              n415 = Subtract(x=w899, y=u16 1) -> (x-y=w896:u16)
              n416 = Index Array(array=w898, index=w897) -> (element=w895:refnum<vi>)
              n417 = Index Array(array=w898, index=w896) -> (element=w894:refnum<vi>)
              n418 = Bundle By Name(cluster="active Axis ref", "Ref X"=w895, "Ref Y"=w894) -> (w892:cluster{"Ref X":refnum<vi>, "Ref Y":refnum<vi>})
            }
            n419 = call <vilib>:"Add State(s) to Queue__jki_lib_state_machine.vi"("State(s) in (\"\")"=w891) -> ("States Out"=w890:string)  [unwired: 14 in]
            n420 = Bundle By Name(cluster=w883, "active axis refs 2"=w870) -> (w882:T37)
          }
          frame "Move Config" {
            # "Your code here.\n(You can make a copy of, or modify, this frame)"
            n421 = Unbundle By Name(w905) -> ("move properties"=w909:T2[], "active ccd"=w908:i32)
            n422 = Replace Array Subset(array=w909, new element="move config", index=w908) -> (w906:T2[])
            n423 = Bundle By Name(cluster=w905, "move properties"=w906) -> (w904:T37)
            n424 = call <vilib>:"Add State(s) to Queue__jki_lib_state_machine.vi"("State(s) in (\"\")"=w912) -> ("States Out"=w911:string)  [unwired: 14 in]
          }
          frame "----------Centroid & Move----------" {
            # "Template Separator\n(You can make a copy of, or modify, this frame)"
            n425 = call <vilib>:"Add State(s) to Queue__jki_lib_state_machine.vi"("State(s) in (\"\")"=w916) -> ("States Out"=w915:string)  [unwired: 14 in]
          }
          frame "detected" {
            n426 = Unbundle By Name(w921) -> ("Offset X"=w956:dbl[][], "Offset Y"=w955:dbl[][], "Size"=w954:dbl[][], "Mean Size"=w953:dbl[][], "Time"=w950:timestamp[][], "Motor X"=w930:dbl[][], "active axis refs 2"=w929:T11, "Motor Y"=w928:dbl[][])
            n427 = Spreadsheet String To Array(format string="%s", spreadsheet string=w933, array type (2D Dbl)=string[] []) -> (array=w924:string[])  [unwired: 1 in]
            n428 = for {
              tunnel: w925 -> [w970] mode=indexing
              tunnel: w924 -> [w969]
              tunnel: [w968] -> w923 mode=indexing
              n429 = for {
                tunnel: w970 -> [w973]
                tunnel: [w972] -> w967 mode=indexing
                tunnel: w969 -> [w971] mode=indexing
                n430 = Equal?(x=w973, y=w971) -> (x = y?=w972:bool)
              }
              n431 = Or Array Elements(Boolean array=w967) -> (logical OR=w968:bool)
            }
            n432 = Unbundle By Name(w921) -> ("Mean Centroid X"=w961:dbl[][], "Mean Centroid Y"=w960:dbl[][], "Centroid X"=w963:dbl[][], "Centroid Y"=w962:dbl[][])
            n433 = call <vilib>:"Build State String with Arguments__jki_lib_state_machine.vi"("Arguments (\"\")"=w933, "State"="stats") -> ("State with Arguments"=w934:string)  [unwired: 4 in]
            n434 = call <vilib>:"Add State(s) to Queue__jki_lib_state_machine.vi"("State(s) in Front (\"\")"=w934, "State(s) in (\"\")"=w932) -> ("States Out"=w931:string)  [unwired: 13 in]
            n435 = for {
              tunnel: w963 -> [w1023]
              tunnel: w962 -> [w1022]
              tunnel: w961 -> [w1021]
              tunnel: w960 -> [w1020]
              tunnel: [w1019] -> w947 mode=indexing
              tunnel: [w1018] -> w958 mode=indexing
              tunnel: w957 -> [w1017] mode=indexing
              tunnel: w956 -> [w1016]
              tunnel: w955 -> [w1015]
              tunnel: [w1014] -> w922 mode=indexing
              tunnel: [w1013] -> w948 mode=indexing
              tunnel: w954 -> [w1012]
              tunnel: w953 -> [w1011]
              tunnel: [w1010] -> w952 mode=indexing
              tunnel: w950 -> [w1009]
              tunnel: [w1008] -> w949 mode=indexing
              tunnel: w930 -> [w1000]
              tunnel: w929 -> [w999]
              tunnel: w928 -> [w998]
              tunnel: [w978] -> w927 mode=indexing
              tunnel: [w977] -> w926 mode=indexing
              tunnel: w923 -> [w976]
              i -> [w975]
              n436 = Unbundle By Name(w1017) -> ("Target.X::12"=w982:refnum<vi>, "Target.Y::12"=w981:refnum<vi>)
              n437 = Index Array(array=w1000, index (row)=w975) -> (element=w1003:dbl[])  [unwired: 1 in]
              n438 = Index Array(array=w999, index=w975) -> (element=w1002:cluster{"Ref X":refnum<vi>, "Ref Y":refnum<vi>})
              n439 = Index Array(array=w998, index (row)=w975) -> (element=w1007:dbl[])  [unwired: 1 in]
              n440 = Index Array(array=w976, index=w975) -> (element=w974:bool)
              n441 = Index Array(array=w1021, index (row)=w975) -> (element=w994:dbl[])  [unwired: 1 in]
              n442 = Index Array(array=w1020, index (row)=w975) -> (element=w995:dbl[])  [unwired: 1 in]
              n443 = Index Array(array=w1023, index (row)=w975) -> (element=w997:dbl[])  [unwired: 1 in]
              n444 = Index Array(array=w1022, index (row)=w975) -> (element=w996:dbl[])  [unwired: 1 in]
              n445 = Index Array(array=w1016, index (row)=w975) -> (element=w990:dbl[])  [unwired: 1 in]
              n446 = Index Array(array=w1015, index (row)=w975) -> (element=w989:dbl[])  [unwired: 1 in]
              n447 = Index Array(array=w1012, index (row)=w975) -> (element=w987:dbl[])  [unwired: 1 in]
              n448 = Index Array(array=w1011, index (row)=w975) -> (element=w986:dbl[])  [unwired: 1 in]
              n449 = Index Array(array=w1009, index (row)=w975) -> (element=w983:timestamp[])  [unwired: 1 in]
              n450 = Unbundle By Name(w1002) -> ("Ref X"=w1001:refnum<vi>, "Ref Y"=w1005:refnum<vi>)
              n451 = property class="DigNum (strict)"(reference=w982) -> ("Value"=w980:dbl)  [unwired: 1 in, 2 out]
              n452 = property class="DigNum (strict)"(reference=w981) -> ("Value"=w979:dbl)  [unwired: 1 in, 2 out]
              n453 = call <vilib>:"Std Deviation and Variance.vi"("X"=w997) -> ("mean"=w993:dbl)  [unwired: 1 in, 2 out]
              n454 = call <vilib>:"Std Deviation and Variance.vi"("X"=w996) -> ("mean"=w992:dbl)  [unwired: 1 in, 2 out]
              n455 = call <vilib>:"Std Deviation and Variance.vi"("X"=w987) -> ("mean"=w985:dbl)  [unwired: 1 in, 2 out]
              n456 = Get Date/Time In Seconds() -> (seconds since 1Jan1904=w984:timestamp)
              n457 = property class="DigNum (strict)"(reference=w1001) -> ("Value"=w1004:dbl)  [unwired: 1 in, 2 out]
              n458 = property class="DigNum (strict)"(reference=w1005) -> ("Value"=w1006:dbl)  [unwired: 1 in, 2 out]
              n459 = Subtract(x=w980, y=w993) -> (x-y=w991:dbl)
              n460 = Subtract(x=w979, y=w992) -> (x-y=w988:dbl)
              n461 = case shown="True" w974 {
                tunnel: [w1036 w1055] -> w1019
                tunnel: [w1024 w1054] -> w1018
                tunnel: [w1025 w1053] -> w1014
                tunnel: [w1026 w1052] -> w1013
                tunnel: [w1027 w1051] -> w1010
                tunnel: [w1028 w1050] -> w1008
                tunnel: w995 -> [w1034 w1049]
                tunnel: w994 -> [w1035 w1048]
                tunnel: w993 -> [_ w1047]
                tunnel: w992 -> [_ w1046]
                tunnel: w991 -> [_ w1045]
                tunnel: w990 -> [w1033 w1044]
                tunnel: w989 -> [w1032 w1043]
                tunnel: w988 -> [_ w1042]
                tunnel: w986 -> [w1031 w1041]
                tunnel: w985 -> [_ w1040]
                tunnel: w984 -> [w1029 w1039]
                tunnel: w983 -> [w1030 w1038]
                frame False {
                  w1037 = 0.0
                  n462 = Build Array (concatenate)(w1035, w1037) -> (w1036:dbl[])
                  n463 = Build Array (concatenate)(w1034, w1037) -> (w1024:dbl[])
                  n464 = Build Array (concatenate)(w1033, w1037) -> (w1025:dbl[])
                  n465 = Build Array (concatenate)(w1032, w1037) -> (w1026:dbl[])
                  n466 = Build Array (concatenate)(w1031, w1037) -> (w1027:dbl[])
                  n467 = Build Array (concatenate)(w1030, w1029) -> (w1028:timestamp[])
                }
                frame True {
                  n468 = Build Array (concatenate)(w1048, w1047) -> (w1055:dbl[])
                  n469 = Build Array (concatenate)(w1049, w1046) -> (w1054:dbl[])
                  n470 = Build Array (concatenate)(w1044, w1045) -> (w1053:dbl[])
                  n471 = Build Array (concatenate)(w1043, w1042) -> (w1052:dbl[])
                  n472 = Build Array (concatenate)(w1041, w1040) -> (w1051:dbl[])
                  n473 = Build Array (concatenate)(w1038, w1039) -> (w1050:timestamp[])
                }
              }
              n474 = Build Array (concatenate)(w1003, w1004) -> (w978:dbl[])
              n475 = Build Array (concatenate)(w1007, w1006) -> (w977:dbl[])
            }
            n476 = local write "Numeric"(0.0 ("Numeric")) -> ()
            n477 = Array Size(array=w922) -> (size(s)=w946:i32[])
            n478 = Index Array(array=w946, index=1) -> (element=w944:i32)
            "History Index" <- w944
            n479 = call <vilib>:"Add State(s) to Queue__jki_lib_state_machine.vi"("State(s) in (\"\")"=w931, "State(s) at Back (\"\")"="Check Move\ntdms" ("State(s) at Back (\"\")")) -> ("States Out"=w938:string)  [unwired: 13 in]
            n480 = Unbundle By Name(w921) -> ("img to avg"=w918:i32)
            n481 = Initialize Array(0.0 ("element"), 12 ("dimension size"), w918) -> (w917:dbl[][])
            n482 = Greater?(x=w944, y="History Size") -> (0:w942:bool)
            n483 = Bundle By Name(cluster=w921, "Centroid X"=w917, "Centroid Y"=w917, "Mean Centroid X"=w947, "Mean Centroid Y"=w958, "Offset X"=w922, "Offset Y"=w948, "Mean Size"=w952, "Size"=w917, "Time"=w949, "Motor X"=w927, "Motor Y"=w926) -> (w959:T37)
            n484 = Select(t="history" ("State(s) at Back (\"\")"), s=w942, f="") -> (s? t:f=w939:string)
            n485 = call <vilib>:"Add State(s) to Queue__jki_lib_state_machine.vi"("State(s) in (\"\")"=w938, "State(s) at Back (\"\")"=w939) -> ("States Out"=w937:string)  [unwired: 13 in]
          }
          frame "Check Move" {
            (unwired) "Device Ini" ("State(s) in Front (\"\")")
            n486 = Unbundle By Name(w1060) -> ("move properties"=w1074:T2[], "Mean Size"=w1073:dbl[][], "move properties"=w1072:T2[], "Offset X"=w1071:dbl[][], "Offset Y"=w1070:dbl[][], "active cams"=w1069:string[])
            n487 = Unbundle By Name(w1060) -> ("steps speed X"=w1059:dbl[], "steps speed Y"=w1058:dbl[])
            n488 = for {
              tunnel: w1072 -> [w1117]
              tunnel: w1071 -> [w1115]
              tunnel: w1070 -> [w1113]
              tunnel: w1073 -> [w1120]
              tunnel: [w1111] -> w1068 mode=indexing
              tunnel: [w1124] -> w1067 mode=indexing
              tunnel: w1069 -> [w1121] mode=indexing
              tunnel: [w1145] -> w1075 mode=indexing
              tunnel: [w1144] -> w1065 mode=indexing
              tunnel: w1074 -> [w1104]
              tunnel: [w1106] -> w1064 mode=indexing
              tunnel: [w1105] -> w1063 mode=indexing
              tunnel: "Speedmode @" -> [w1110]
              tunnel: w1061 -> [w1122]
              shift-right: [w1097] -> w1057
              shift-left: w1059 -> [w1102]
              shift-right: [w1096] -> w1056
              shift-left: w1058 -> [w1101]
              n489 = call-poly <userlib>:"Filter 1D Array__ogtk.vi"("items to filter"=w1121, "array"=w1122) -> ("filtered item indices"=w1123:i32[])  [unwired: 4 in, 1 out]
              n490 = Index Array(array=w1123) -> (element=w1100:i32)  [unwired: 1 in]
              n491 = Index Array(array=w1104, index=w1100) -> (element=w1119:T2)
              n492 = Index Array(array=w1120, index (row)=w1100) -> (element=w1118:dbl[])  [unwired: 1 in]
              n493 = Index Array(array=w1117, index=w1100) -> (element=w1116:T2)
              n494 = Index Array(array=w1115, index (row)=w1100) -> (element=w1114:dbl[])  [unwired: 1 in]
              n495 = Index Array(array=w1113, index (row)=w1100) -> (element=w1112:dbl[])  [unwired: 1 in]
              n496 = Unbundle By Name(w1116) -> ("Tolerance [%]"=w1138:dbl)
              n497 = Reverse 1D Array(array=w1114) -> (reversed array=w1143:dbl[])
              n498 = Reverse 1D Array(array=w1112) -> (reversed array=w1142:dbl[])
              n499 = Reverse 1D Array(array=w1118) -> (reversed array=w1137:dbl[])
              n500 = Unbundle By Name(w1119) -> ("Stepsize"=w1103:dbl, "enable feedback"=w1127:bool)
              n501 = Index Array(array=w1143) -> (element=w1141:dbl)  [unwired: 1 in]
              n502 = Index Array(array=w1142) -> (element=w1140:dbl)  [unwired: 1 in]
              n503 = Index Array(array=w1137) -> (element=w1136:dbl)  [unwired: 1 in]
              n504 = Absolute Value(x=w1141) -> (abs(x)=w1107:dbl)
              n505 = Absolute Value(x=w1140) -> (abs(x)=w1108:dbl)
              n506 = Square Root(x=w1136) -> (sqrt(x)=w1135:dbl)
              n507 = Divide(x=w1138, y=100.0) -> (x/y=w1134:dbl)
              n508 = Multiply(x=w1135, y=w1134) -> (x*y=w1109:dbl)
              n509 = Not Equal To 0?(x=w1108) -> (x != 0?=w1125:bool)
              n510 = Not Equal To 0?(x=w1107) -> (x != 0?=w1129:bool)
              n511 = Greater Or Equal?(x=w1107, y=w1109) -> (x >= y?=w1128:bool)
              n512 = Greater Or Equal?(x=w1108, y=w1109) -> (x >= y?=w1126:bool)
              n513 = Compound Arithmetic op=AND(w1127, w1129, w1128) -> (w1111:bool)
              n514 = Compound Arithmetic op=AND(w1127, w1126, w1125) -> (w1124:bool)
              n515 = call "speedmode.vi"("offset X"=w1107, "offset Y"=w1108, "beamsize x tolerance"=w1109, "Speedmode @"=w1110, "step size"=w1103) -> ("steps speed Y"=w1098:dbl, "steps speed X"=w1099:dbl, "speedmode X"=w1106:bool, "speedmode Y"=w1105:bool)  [unwired: 3 in]
              n516 = Boolean To (0,1)(Boolean=w1124) -> (0, 1=w1130:i16)
              n517 = Replace Array Subset(array=w1101, new element=w1098, index=w1100) -> (w1096:dbl[])
              n518 = Replace Array Subset(array=w1102, new element=w1099, index=w1100) -> (w1097:dbl[])
              n519 = Multiply(x=w1130, y=w1108) -> (x*y=w1131:dbl)
              n520 = Boolean To (0,1)(Boolean=w1111) -> (0, 1=w1133:i16)
              n521 = Multiply(x=w1133, y=w1107) -> (x*y=w1132:dbl)
              n522 = Bundle(w1131, "GUIdevice 8"=w1121) -> (w1144:cluster{dbl, "GUIdevice 8":string})  [unwired: 1 in]
              n523 = Bundle(w1132, "GUIdevice 8"=w1121) -> (w1145:cluster{dbl, "GUIdevice 8":string})  [unwired: 1 in]
            }
            "required X" <- w1068
            "required Y" <- w1067
            "speedmode X" <- w1064
            "speedmode Y" <- w1063
            n524 = case shown="True" "Align" {
              tunnel: w1075 -> [w1151 w1156]
              tunnel: w1065 -> [w1150 w1153]
              tunnel: [w1149 w1155] -> w1078
              tunnel: [w1148 w1152] -> w1077
              frame False {
                n525 = Sort 1D Array(array=w1150) -> (sorted array=w1147:cluster{dbl, "GUIdevice 8":string}[])
                n526 = Sort 1D Array(array=w1151) -> (sorted array=w1146:cluster{dbl, "GUIdevice 8":string}[])
                n527 = Reverse 1D Array(array=w1147) -> (reversed array=w1148:cluster{dbl, "GUIdevice 8":string}[])
                n528 = Reverse 1D Array(array=w1146) -> (reversed array=w1149:cluster{dbl, "GUIdevice 8":string}[])
              }
              frame True {
                w1154 = cluster{dbl, "GUIdevice 8":string}[] [] ("Array")
                n529 = for {
                  shift-right: [w1166] -> w1155
                  shift-left: w1154 -> [w1168]
                  tunnel: w1156 -> [w1167] mode=indexing
                  n530 = Unbundle(w1167) -> (w1170:dbl)  [unwired: 1 out]
                  n531 = Not Equal To 0?(x=w1170) -> (x != 0?=w1169:bool)
                  n532 = case shown="True" w1169 {
                    tunnel: w1168 -> [w1171 w1174]
                    tunnel: w1167 -> [_ w1173]
                    tunnel: [w1171 w1172] -> w1166
                    frame False {
                    }
                    frame True {
                      n533 = Build Array (concatenate)(w1174, w1173) -> (w1172:cluster{dbl, "GUIdevice 8":string}[])
                    }
                  }
                }
                n534 = for {
                  shift-right: [w1157] -> w1152
                  shift-left: w1154 -> [w1159]
                  tunnel: w1153 -> [w1158] mode=indexing
                  n535 = Unbundle(w1158) -> (w1161:dbl)  [unwired: 1 out]
                  n536 = Not Equal To 0?(x=w1161) -> (x != 0?=w1160:bool)
                  n537 = case shown="True" w1160 {
                    tunnel: w1159 -> [w1162 w1165]
                    tunnel: w1158 -> [_ w1164]
                    tunnel: [w1162 w1163] -> w1157
                    frame False {
                    }
                    frame True {
                      n538 = Build Array (concatenate)(w1165, w1164) -> (w1163:cluster{dbl, "GUIdevice 8":string}[])
                    }
                  }
                }
              }
            }
            n539 = call <vilib>:"Add State(s) to Queue__jki_lib_state_machine.vi"("State(s) in (\"\")"=w1081) -> ("States Out"=w1080:string)  [unwired: 14 in]
            n540 = Bundle By Name(cluster=w1060, "steps speed X"=w1057, "steps speed Y"=w1056, "speedmode X"=w1064, "speedmode Y"=w1063) -> (w1062:T37)
            n541 = Index Array(array=w1077) -> (element=w1082:cluster{dbl, "GUIdevice 8":string})  [unwired: 1 in]
            n542 = Index Array(array=w1078) -> (element=w1083:cluster{dbl, "GUIdevice 8":string})  [unwired: 1 in]
            n543 = Empty Array?(array=w1077) -> (empty?=w1085:bool)
            n544 = Unbundle(w1083) -> (w1091:dbl)  [unwired: 1 out]
            n545 = Unbundle(w1082) -> (w1087:dbl)  [unwired: 1 out]
            n546 = Unbundle By Name(w1062) -> ("Feedback global"=w1092:bool)
            n547 = Empty Array?(array=w1078) -> (empty?=w1089:bool)
            n548 = property on="autodetect" class="Bool (strict)"("Value"=FALSE ("autodetect")) -> ()  [unwired: 2 in, 2 out]
            n549 = Equal To 0?(x=w1091) -> (x = 0?=w1090:bool)
            n550 = Equal To 0?(x=w1087) -> (x = 0?=w1086:bool)
            n551 = Or(x=w1090, y=w1089) -> (x .or. y?=w1088:bool)
            n552 = Or(x=w1086, y=w1085) -> (x .or. y?=w1084:bool)
            n553 = case shown="True" w1092 {
              tunnel: w1088 -> [_ w1182]
              tunnel: w1078 -> [_ w1181]
              tunnel: w1084 -> [_ w1179]
              tunnel: w1077 -> [_ w1178]
              tunnel: w1080 -> [w1175 w1177]
              tunnel: [w1175 w1176] -> w1093
              frame False {
              }
              frame True {
                n554 = case shown="False" w1182 {
                  tunnel: w1181 -> [w1198 _]
                  tunnel: w1177 -> [w1194 w1199]
                  tunnel: [w1192 w1199] -> w1180
                  frame False {
                    n555 = Index Array(array=w1198) -> (element=w1197:cluster{dbl, "GUIdevice 8":string})  [unwired: 1 in]
                    n556 = Unbundle By Name(w1197) -> ("GUIdevice 8"=w1196:string)
                    n557 = Wait (ms)(milliseconds to wait=u32 100) -> ()  [unwired: 1 out]
                    n558 = call <vilib>:"Build State String with Arguments__jki_lib_state_machine.vi"("Arguments (\"\")"=w1196, "State"="Move X") -> ("State with Arguments"=w1193:string)  [unwired: 4 in]
                    n559 = call <vilib>:"Add State(s) to Queue__jki_lib_state_machine.vi"("State(s) in (\"\")"=w1194, "State(s) at Back (\"\")"=w1193) -> ("States Out"=w1192:string)  [unwired: 13 in]
                  }
                  frame True {
                  }
                }
                n560 = case shown="False" w1179 {
                  tunnel: w1178 -> [w1189 _]
                  tunnel: w1180 -> [w1185 w1190]
                  tunnel: [w1183 w1190] -> w1176
                  frame False {
                    n561 = Index Array(array=w1189) -> (element=w1188:cluster{dbl, "GUIdevice 8":string})  [unwired: 1 in]
                    n562 = Unbundle By Name(w1188) -> ("GUIdevice 8"=w1187:string)
                    n563 = call <vilib>:"Build State String with Arguments__jki_lib_state_machine.vi"("Arguments (\"\")"=w1187, "State"="Move Y") -> ("State with Arguments"=w1184:string)  [unwired: 4 in]
                    n564 = call <vilib>:"Add State(s) to Queue__jki_lib_state_machine.vi"("State(s) in (\"\")"=w1185, "State(s) at Back (\"\")"=w1184) -> ("States Out"=w1183:string)  [unwired: 13 in]
                  }
                  frame True {
                  }
                }
              }
            }
            n565 = call <vilib>:"Add State(s) to Queue__jki_lib_state_machine.vi"("State(s) in (\"\")"=w1080, "State(s) at Back (\"\")"=w1093) -> ("States Out"=w1095:string)  [unwired: 13 in]
          }
          frame "Move X" {
            # "Your code here.\n(You can make a copy of, or modify, this frame)"
            n566 = Unbundle By Name(w1203) -> ("Offset X"=w1223:dbl[][])
            n567 = call-poly <userlib>:"Filter 1D Array__ogtk.vi"("items to filter"=w1209, "array"=w1227) -> ("filtered item indices"=w1214:i32[])  [unwired: 4 in, 1 out]
            n568 = Unbundle By Name(w1203) -> ("active axis refs 2"=w1226:T11, "move properties"=w1213:T2[])
            n569 = for {
              tunnel: w1214 -> [w1232] mode=indexing
              tunnel: w1213 -> [w1236]
              shift-right: [w1231] -> w1211
              shift-left: i32[] [] ("filtered item indices") -> [w1234]
              n570 = Index Array(array=w1236, index=w1232) -> (element=w1235:T2)
              n571 = Unbundle By Name(w1235) -> ("enable feedback"=w1233:bool)
              n572 = case shown="True" w1233 {
                tunnel: w1234 -> [w1237 w1240]
                tunnel: w1232 -> [_ w1239]
                tunnel: [w1237 w1238] -> w1231
                frame False {
                }
                frame True {
                  n573 = Build Array (concatenate)(w1240, w1239) -> (w1238:i32[])
                }
              }
            }
            n574 = Index Array(array=w1211) -> (element=w1202:i32)  [unwired: 1 in]
            n575 = Index Array(array=w1223, index (row)=w1202) -> (element=w1222:dbl[])  [unwired: 1 in]
            n576 = Reverse 1D Array(array=w1222) -> (reversed array=w1221:dbl[])
            n577 = Index Array(array=w1226, index=w1202) -> (element=w1225:cluster{"Ref X":refnum<vi>, "Ref Y":refnum<vi>})
            n578 = Index Array(array=w1221) -> (element=w1219:dbl)  [unwired: 1 in]
            n579 = Index Array(array=w1213, index=w1202) -> (element=w1224:T2)
            n580 = Unbundle By Name(w1225) -> ("Ref X"=w1217:refnum<vi>, "Ref Y"=w1216:refnum<vi>)
            n581 = Unbundle By Name(w1224) -> ("Invert Direction X"=w1201:bool, "Invert Axis"=w1220:bool, "enable feedback"=w1215:bool)
            n582 = Greater Or Equal To 0?(x=w1219) -> (x >= 0?=w1218:bool)
            n583 = Unbundle By Name(w1203) -> ("steps speed Y"=w1204:dbl[], "steps speed X"=w1205:dbl[])
            n584 = Index Array(array=w1205, index=w1202) -> (element=w1207:dbl)
            n585 = Index Array(array=w1204, index=w1202) -> (element=w1206:dbl)
            n586 = Select(t=w1206, s=w1201, f=w1207) -> (s? t:f=w1200:dbl)
            n587 = case shown="True" w1215 {
              tunnel: w1220 -> [_ w1246]
              tunnel: w1218 -> [_ w1245]
              tunnel: w1200 -> [_ w1244]
              tunnel: w1201 -> [_ w1243]
              tunnel: w1217 -> [_ w1242]
              tunnel: w1216 -> [_ w1241]
              frame False {
              }
              frame True {
                n588 = case shown="False" w1245 {
                  tunnel: w1243 -> [w1254 w1276]
                  tunnel: w1244 -> [w1252 w1274]
                  tunnel: w1246 -> [w1251 w1273]
                  tunnel: w1246 -> [w1250 w1272]
                  tunnel: w1242 -> [w1248 w1270]
                  tunnel: w1241 -> [w1247 w1269]
                  frame True {
                    n589 = case shown="False" w1251 {
                      tunnel: [w1265 w1267] -> w1253
                      tunnel: w1248 -> [w1266 _]
                      tunnel: w1247 -> [_ w1268]
                      frame False {
                        n590 = property class="DigNum (strict)"(reference=w1266) -> ("Value"=w1265:dbl)  [unwired: 1 in, 2 out]
                      }
                      frame True {
                        n591 = property class="DigNum (strict)"(reference=w1268) -> ("Value"=w1267:dbl)  [unwired: 1 in, 2 out]
                      }
                    }
                    n592 = case shown="False" w1254 {
                      tunnel: w1253 -> [w1261 w1264]
                      tunnel: w1252 -> [w1260 w1263]
                      tunnel: [w1259 w1262] -> w1249
                      frame False {
                        n593 = Add(x=w1261, y=w1260) -> (x+y=w1259:dbl)
                      }
                      frame True {
                        n594 = Subtract(x=w1264, y=w1263) -> (x-y=w1262:dbl)
                      }
                    }
                    n595 = case shown="False" w1250 {
                      tunnel: w1249 -> [w1255 w1257]
                      tunnel: w1248 -> [w1256 _]
                      tunnel: w1247 -> [_ w1258]
                      frame False {
                        n596 = property class="DigNum (strict)"(reference=w1256, "Val(Sgnl)"=w1255) -> ()  [unwired: 1 in, 2 out]
                      }
                      frame True {
                        n597 = property class="DigNum (strict)"(reference=w1258, "Val(Sgnl)"=w1257) -> ()  [unwired: 1 in, 2 out]
                      }
                    }
                  }
                  frame False {
                    n598 = case shown="False" w1273 {
                      tunnel: [w1287 w1289] -> w1275
                      tunnel: w1270 -> [w1288 _]
                      tunnel: w1269 -> [_ w1290]
                      frame False {
                        n599 = property class="DigNum (strict)"(reference=w1288) -> ("Value"=w1287:dbl)  [unwired: 1 in, 2 out]
                      }
                      frame True {
                        n600 = property class="DigNum (strict)"(reference=w1290) -> ("Value"=w1289:dbl)  [unwired: 1 in, 2 out]
                      }
                    }
                    n601 = case shown="False" w1276 {
                      tunnel: w1275 -> [w1283 w1286]
                      tunnel: w1274 -> [w1282 w1285]
                      tunnel: [w1281 w1284] -> w1271
                      frame False {
                        n602 = Subtract(x=w1283, y=w1282) -> (x-y=w1281:dbl)
                      }
                      frame True {
                        n603 = Add(x=w1286, y=w1285) -> (x+y=w1284:dbl)
                      }
                    }
                    n604 = case shown="False" w1272 {
                      tunnel: w1271 -> [w1277 w1279]
                      tunnel: w1270 -> [w1278 _]
                      tunnel: w1269 -> [_ w1280]
                      frame False {
                        n605 = property class="DigNum (strict)"(reference=w1278, "Val(Sgnl)"=w1277) -> ()  [unwired: 1 in, 2 out]
                      }
                      frame True {
                        n606 = property class="DigNum (strict)"(reference=w1280, "Val(Sgnl)"=w1279) -> ()  [unwired: 1 in, 2 out]
                      }
                    }
                  }
                }
              }
            }
            n607 = call <vilib>:"Build State String with Arguments__jki_lib_state_machine.vi"("Arguments (\"\")"=w1209, "State"="Wait" ("State(s) in Front (\"\")")) -> ("State with Arguments"=w1208:string)  [unwired: 4 in]
            n608 = call <vilib>:"Add State(s) to Queue__jki_lib_state_machine.vi"("State(s) in Front (\"\")"=w1208, "State(s) in (\"\")"=w1230) -> ("States Out"=w1229:string)  [unwired: 13 in]
            "Moving X" <- w1209
          }
          frame "ManMove X" {
            # "Your code here.\n(You can make a copy of, or modify, this frame)"
            n609 = Equal?(x=w1296, y="Right") -> (x = y?=w1297:bool)
            n610 = Unbundle By Name(w1306) -> ("move properties"=w1301:T2[], "active ccd"=w1294:i32, "active man refs"=w1299:cluster{"Ref X":refnum<vi>, "Ref Y":refnum<vi>}, "active cams"=w1295:string[])
            n611 = Index Array(array=w1295, index=w1294) -> (element=w1292:string)
            n612 = Index Array(array=w1301, index=w1294) -> (element=w1307:T2)
            n613 = Unbundle By Name(w1299) -> ("Ref X"=w1303:refnum<vi>, "Ref Y"=w1302:refnum<vi>)
            n614 = Unbundle By Name(w1307) -> ("Invert Direction X"=w1304:bool, "Invert Axis"=w1305:bool)
            n615 = call <vilib>:"Build State String with Arguments__jki_lib_state_machine.vi"("Arguments (\"\")"=w1292, "State"="Wait" ("State(s) in Front (\"\")")) -> ("State with Arguments"=w1291:string)  [unwired: 4 in]
            n616 = call <vilib>:"Add State(s) to Queue__jki_lib_state_machine.vi"("State(s) in Front (\"\")"=w1291, "State(s) in (\"\")"=w1310) -> ("States Out"=w1309:string)  [unwired: 13 in]
            n617 = case shown="False" w1297 {
              tunnel: w1304 -> [w1318 w1340]
              tunnel: "StepSize" -> [w1316 w1338]
              tunnel: w1305 -> [w1315 w1337]
              tunnel: w1305 -> [w1314 w1336]
              tunnel: w1303 -> [w1312 w1334]
              tunnel: w1302 -> [w1311 w1333]
              frame True {
                n618 = case shown="False" w1315 {
                  tunnel: [w1329 w1331] -> w1317
                  tunnel: w1312 -> [w1330 _]
                  tunnel: w1311 -> [_ w1332]
                  frame False {
                    n619 = property class="DigNum (strict)"(reference=w1330) -> ("Value"=w1329:dbl)  [unwired: 1 in, 2 out]
                  }
                  frame True {
                    n620 = property class="DigNum (strict)"(reference=w1332) -> ("Value"=w1331:dbl)  [unwired: 1 in, 2 out]
                  }
                }
                n621 = case shown="False" w1318 {
                  tunnel: w1317 -> [w1325 w1328]
                  tunnel: w1316 -> [w1324 w1327]
                  tunnel: [w1323 w1326] -> w1313
                  frame False {
                    n622 = Add(x=w1325, y=w1324) -> (x+y=w1323:dbl)
                  }
                  frame True {
                    n623 = Subtract(x=w1328, y=w1327) -> (x-y=w1326:dbl)
                  }
                }
                n624 = case shown="False" w1314 {
                  tunnel: w1313 -> [w1319 w1321]
                  tunnel: w1312 -> [w1320 _]
                  tunnel: w1311 -> [_ w1322]
                  frame False {
                    n625 = property class="DigNum (strict)"(reference=w1320, "Val(Sgnl)"=w1319) -> ()  [unwired: 1 in, 2 out]
                  }
                  frame True {
                    n626 = property class="DigNum (strict)"(reference=w1322, "Val(Sgnl)"=w1321) -> ()  [unwired: 1 in, 2 out]
                  }
                }
              }
              frame False {
                n627 = case shown="True" w1337 {
                  tunnel: [w1351 w1353] -> w1339
                  tunnel: w1334 -> [w1352 _]
                  tunnel: w1333 -> [_ w1354]
                  frame False {
                    n628 = property class="DigNum (strict)"(reference=w1352) -> ("Value"=w1351:dbl)  [unwired: 1 in, 2 out]
                  }
                  frame True {
                    n629 = property class="DigNum (strict)"(reference=w1354) -> ("Value"=w1353:dbl)  [unwired: 1 in, 2 out]
                  }
                }
                n630 = case shown="True" w1340 {
                  tunnel: w1339 -> [w1347 w1350]
                  tunnel: w1338 -> [w1346 w1349]
                  tunnel: [w1345 w1348] -> w1335
                  frame False {
                    n631 = Subtract(x=w1347, y=w1346) -> (x-y=w1345:dbl)
                  }
                  frame True {
                    n632 = Add(x=w1350, y=w1349) -> (x+y=w1348:dbl)
                  }
                }
                n633 = case shown="False" w1336 {
                  tunnel: w1335 -> [w1341 w1343]
                  tunnel: w1334 -> [w1342 _]
                  tunnel: w1333 -> [_ w1344]
                  frame False {
                    n634 = property class="DigNum (strict)"(reference=w1342, "Val(Sgnl)"=w1341) -> ()  [unwired: 1 in, 2 out]
                  }
                  frame True {
                    n635 = property class="DigNum (strict)"(reference=w1344, "Val(Sgnl)"=w1343) -> ()  [unwired: 1 in, 2 out]
                  }
                }
              }
            }
          }
          frame "ManMove Y" {
            # "Your code here.\n(You can make a copy of, or modify, this frame)"
            n636 = Equal?(x=w1360, y="Down") -> (x = y?=w1364:bool)
            n637 = Unbundle By Name(w1370) -> ("active cams"=w1359:string[], "move properties"=w1369:T2[], "active ccd"=w1358:i32, "active man refs"=w1368:cluster{"Ref X":refnum<vi>, "Ref Y":refnum<vi>})
            n638 = Index Array(array=w1359, index=w1358) -> (element=w1356:string)
            n639 = property on="StepSize" class="DigNum (strict)"() -> ("Value"=w1361:dbl)  [unwired: 2 in, 2 out]
            n640 = Index Array(array=w1369, index=w1358) -> (element=w1371:T2)
            n641 = Unbundle By Name(w1368) -> ("Ref Y"=w1363:refnum<vi>, "Ref X"=w1362:refnum<vi>)
            n642 = Unbundle By Name(w1371) -> ("Invert Direction Y"=w1366:bool, "Invert Axis"=w1365:bool)
            n643 = call <vilib>:"Build State String with Arguments__jki_lib_state_machine.vi"("Arguments (\"\")"=w1356, "State"="Wait" ("State(s) in Front (\"\")")) -> ("State with Arguments"=w1355:string)  [unwired: 4 in]
            n644 = call <vilib>:"Add State(s) to Queue__jki_lib_state_machine.vi"("State(s) in Front (\"\")"=w1355, "State(s) in (\"\")"=w1374) -> ("States Out"=w1373:string)  [unwired: 13 in]
            n645 = case shown="True" w1364 {
              tunnel: w1366 -> [w1382 w1404]
              tunnel: w1361 -> [w1380 w1402]
              tunnel: w1365 -> [w1379 w1401]
              tunnel: w1365 -> [w1378 w1400]
              tunnel: w1363 -> [w1376 w1398]
              tunnel: w1362 -> [w1375 w1397]
              frame True {
                n646 = case shown="False" w1379 {
                  tunnel: [w1393 w1395] -> w1381
                  tunnel: w1376 -> [w1394 _]
                  tunnel: w1375 -> [_ w1396]
                  frame False {
                    n647 = property class="DigNum (strict)"(reference=w1394) -> ("Value"=w1393:dbl)  [unwired: 1 in, 2 out]
                  }
                  frame True {
                    n648 = property class="DigNum (strict)"(reference=w1396) -> ("Value"=w1395:dbl)  [unwired: 1 in, 2 out]
                  }
                }
                n649 = case shown="False" w1382 {
                  tunnel: w1381 -> [w1389 w1392]
                  tunnel: w1380 -> [w1388 w1391]
                  tunnel: [w1387 w1390] -> w1377
                  frame False {
                    n650 = Add(x=w1389, y=w1388) -> (x+y=w1387:dbl)
                  }
                  frame True {
                    n651 = Subtract(x=w1392, y=w1391) -> (x-y=w1390:dbl)
                  }
                }
                n652 = case shown="False" w1378 {
                  tunnel: w1377 -> [w1383 w1385]
                  tunnel: w1376 -> [w1384 _]
                  tunnel: w1375 -> [_ w1386]
                  frame False {
                    n653 = property class="DigNum (strict)"(reference=w1384, "Val(Sgnl)"=w1383) -> ()  [unwired: 1 in, 2 out]
                  }
                  frame True {
                    n654 = property class="DigNum (strict)"(reference=w1386, "Val(Sgnl)"=w1385) -> ()  [unwired: 1 in, 2 out]
                  }
                }
              }
              frame False {
                n655 = case shown="False" w1401 {
                  tunnel: [w1415 w1417] -> w1403
                  tunnel: w1398 -> [w1416 _]
                  tunnel: w1397 -> [_ w1418]
                  frame False {
                    n656 = property class="DigNum (strict)"(reference=w1416) -> ("Value"=w1415:dbl)  [unwired: 1 in, 2 out]
                  }
                  frame True {
                    n657 = property class="DigNum (strict)"(reference=w1418) -> ("Value"=w1417:dbl)  [unwired: 1 in, 2 out]
                  }
                }
                n658 = case shown="False" w1404 {
                  tunnel: w1403 -> [w1411 w1414]
                  tunnel: w1402 -> [w1410 w1413]
                  tunnel: [w1409 w1412] -> w1399
                  frame False {
                    n659 = Subtract(x=w1411, y=w1410) -> (x-y=w1409:dbl)
                  }
                  frame True {
                    n660 = Add(x=w1414, y=w1413) -> (x+y=w1412:dbl)
                  }
                }
                n661 = case shown="False" w1400 {
                  tunnel: w1399 -> [w1405 w1407]
                  tunnel: w1398 -> [w1406 _]
                  tunnel: w1397 -> [_ w1408]
                  frame False {
                    n662 = property class="DigNum (strict)"(reference=w1406, "Val(Sgnl)"=w1405) -> ()  [unwired: 1 in, 2 out]
                  }
                  frame True {
                    n663 = property class="DigNum (strict)"(reference=w1408, "Val(Sgnl)"=w1407) -> ()  [unwired: 1 in, 2 out]
                  }
                }
              }
            }
          }
          frame "Move Y" {
            # "Your code here.\n(You can make a copy of, or modify, this frame)"
            n664 = Unbundle By Name(w1426) -> ("Offset Y"=w1442:dbl[][])
            n665 = call-poly <userlib>:"Filter 1D Array__ogtk.vi"("items to filter"=w1428, "array"=w1446) -> ("filtered item indices"=w1433:i32[])  [unwired: 4 in, 1 out]
            n666 = Unbundle By Name(w1426) -> ("active axis refs 2"=w1445:T11, "move properties"=w1431:T2[])
            n667 = for {
              tunnel: w1433 -> [w1451] mode=indexing
              tunnel: w1431 -> [w1455]
              shift-right: [w1450] -> w1432
              shift-left: i32[] [] ("filtered item indices") -> [w1453]
              n668 = Index Array(array=w1455, index=w1451) -> (element=w1454:T2)
              n669 = Unbundle By Name(w1454) -> ("enable feedback"=w1452:bool)
              n670 = case shown="True" w1452 {
                tunnel: w1453 -> [w1456 w1459]
                tunnel: w1451 -> [_ w1458]
                tunnel: [w1456 w1457] -> w1450
                frame False {
                }
                frame True {
                  n671 = Build Array (concatenate)(w1459, w1458) -> (w1457:i32[])
                }
              }
            }
            n672 = Index Array(array=w1432) -> (element=w1423:i32)  [unwired: 1 in]
            n673 = Index Array(array=w1442, index (row)=w1423) -> (element=w1441:dbl[])  [unwired: 1 in]
            n674 = Reverse 1D Array(array=w1441) -> (reversed array=w1440:dbl[])
            n675 = Index Array(array=w1445, index=w1423) -> (element=w1444:cluster{"Ref X":refnum<vi>, "Ref Y":refnum<vi>})
            n676 = Index Array(array=w1440) -> (element=w1438:dbl)  [unwired: 1 in]
            n677 = Index Array(array=w1431, index=w1423) -> (element=w1443:T2)
            n678 = Unbundle By Name(w1444) -> ("Ref Y"=w1436:refnum<vi>, "Ref X"=w1435:refnum<vi>)
            n679 = Unbundle By Name(w1426) -> ("steps speed X"=w1425:dbl[], "steps speed Y"=w1424:dbl[])
            n680 = Unbundle By Name(w1443) -> ("Invert Direction Y"=w1420:bool, "Invert Axis"=w1439:bool, "enable feedback"=w1434:bool)
            n681 = Greater Or Equal To 0?(x=w1438) -> (x >= 0?=w1437:bool)
            n682 = Index Array(array=w1425, index=w1423) -> (element=w1422:dbl)
            n683 = Index Array(array=w1424, index=w1423) -> (element=w1421:dbl)
            n684 = Select(t=w1422, s=w1420, f=w1421) -> (s? t:f=w1419:dbl)
            n685 = case shown="True" w1434 {
              tunnel: w1439 -> [_ w1465]
              tunnel: w1437 -> [_ w1464]
              tunnel: w1419 -> [_ w1463]
              tunnel: w1420 -> [_ w1462]
              tunnel: w1436 -> [_ w1461]
              tunnel: w1435 -> [_ w1460]
              frame False {
              }
              frame True {
                n686 = case shown="True" w1464 {
                  tunnel: w1462 -> [w1473 w1495]
                  tunnel: w1463 -> [w1471 w1493]
                  tunnel: w1465 -> [w1470 w1492]
                  tunnel: w1465 -> [w1469 w1491]
                  tunnel: w1461 -> [w1467 w1489]
                  tunnel: w1460 -> [w1466 w1488]
                  frame True {
                    n687 = case shown="False" w1470 {
                      tunnel: [w1484 w1486] -> w1472
                      tunnel: w1467 -> [w1485 _]
                      tunnel: w1466 -> [_ w1487]
                      frame False {
                        n688 = property class="DigNum (strict)"(reference=w1485) -> ("Value"=w1484:dbl)  [unwired: 1 in, 2 out]
                      }
                      frame True {
                        n689 = property class="DigNum (strict)"(reference=w1487) -> ("Value"=w1486:dbl)  [unwired: 1 in, 2 out]
                      }
                    }
                    n690 = case shown="False" w1473 {
                      tunnel: w1472 -> [w1480 w1483]
                      tunnel: w1471 -> [w1479 w1482]
                      tunnel: [w1478 w1481] -> w1468
                      frame False {
                        n691 = Add(x=w1480, y=w1479) -> (x+y=w1478:dbl)
                      }
                      frame True {
                        n692 = Subtract(x=w1483, y=w1482) -> (x-y=w1481:dbl)
                      }
                    }
                    n693 = case shown="False" w1469 {
                      tunnel: w1468 -> [w1474 w1476]
                      tunnel: w1467 -> [w1475 _]
                      tunnel: w1466 -> [_ w1477]
                      frame False {
                        n694 = property class="DigNum (strict)"(reference=w1475, "Val(Sgnl)"=w1474) -> ()  [unwired: 1 in, 2 out]
                      }
                      frame True {
                        n695 = property class="DigNum (strict)"(reference=w1477, "Val(Sgnl)"=w1476) -> ()  [unwired: 1 in, 2 out]
                      }
                    }
                  }
                  frame False {
                    n696 = case shown="False" w1492 {
                      tunnel: [w1506 w1508] -> w1494
                      tunnel: w1489 -> [w1507 _]
                      tunnel: w1488 -> [_ w1509]
                      frame False {
                        n697 = property class="DigNum (strict)"(reference=w1507) -> ("Value"=w1506:dbl)  [unwired: 1 in, 2 out]
                      }
                      frame True {
                        n698 = property class="DigNum (strict)"(reference=w1509) -> ("Value"=w1508:dbl)  [unwired: 1 in, 2 out]
                      }
                    }
                    n699 = case shown="False" w1495 {
                      tunnel: w1494 -> [w1502 w1505]
                      tunnel: w1493 -> [w1501 w1504]
                      tunnel: [w1500 w1503] -> w1490
                      frame False {
                        n700 = Subtract(x=w1502, y=w1501) -> (x-y=w1500:dbl)
                      }
                      frame True {
                        n701 = Add(x=w1505, y=w1504) -> (x+y=w1503:dbl)
                      }
                    }
                    n702 = case shown="False" w1491 {
                      tunnel: w1490 -> [w1496 w1498]
                      tunnel: w1489 -> [w1497 _]
                      tunnel: w1488 -> [_ w1499]
                      frame False {
                        n703 = property class="DigNum (strict)"(reference=w1497, "Val(Sgnl)"=w1496) -> ()  [unwired: 1 in, 2 out]
                      }
                      frame True {
                        n704 = property class="DigNum (strict)"(reference=w1499, "Val(Sgnl)"=w1498) -> ()  [unwired: 1 in, 2 out]
                      }
                    }
                  }
                }
              }
            }
            n705 = call <vilib>:"Build State String with Arguments__jki_lib_state_machine.vi"("Arguments (\"\")"=w1428, "State"="Wait" ("State(s) in Front (\"\")")) -> ("State with Arguments"=w1427:string)  [unwired: 4 in]
            n706 = call <vilib>:"Add State(s) to Queue__jki_lib_state_machine.vi"("State(s) in Front (\"\")"=w1427, "State(s) in (\"\")"=w1449) -> ("States Out"=w1448:string)  [unwired: 13 in]
            "Moving Y" <- w1428
          }
          frame "Wait" {
            # "Your code here.\n(You can make a copy of, or modify, this frame)"
            n707 = flat-sequence {
              tunnel: T20."Disabled and Grayed Out" ("Disabled") -> [w1526]
              tunnel: w1516 -> [w1535]
              tunnel: w1515 -> [w1534]
              tunnel: [w1533] -> w1514
              tunnel: w1513 -> [w1532]
              tunnel: w1512 -> [w1531]
              tunnel: T20."Enabled" ("Disabled") -> [w1545]
              frame #0 {
                n708 = property on="Right" class="Bool (strict)"("DisabledEnum"=w1526) -> ()  [unwired: 2 in, 2 out]
                n709 = property on="Up" class="Bool (strict)"("DisabledEnum"=w1526) -> ()  [unwired: 2 in, 2 out]
                n710 = property on="Left" class="Bool (strict)"("DisabledEnum"=w1526) -> ()  [unwired: 2 in, 2 out]
                n711 = property on="Down" class="Bool (strict)"("DisabledEnum"=w1526) -> ()  [unwired: 2 in, 2 out]
                n712 = property on="StepSize" class="DigNum (strict)"("DisabledEnum"=w1526) -> ()  [unwired: 2 in, 2 out]
              }
              frame #1 {
                n713 = Wait (ms)(milliseconds to wait=u32 1500) -> ()  [unwired: 1 out]
              }
              frame #2 {
                n714 = property on="Moving Y" class="Str"("Value"="") -> ()  [unwired: 2 in, 2 out]
                n715 = property on="Moving X" class="Str"("Value"="") -> ()  [unwired: 2 in, 2 out]
              }
              frame #3 {
                n716 = Equal?(x=w1531, y=w1532) -> (x = y?=w1530:bool)
                n717 = case shown="True" w1530 {
                  tunnel: w1535 -> [_ w1542]
                  tunnel: w1534 -> [w1536 w1539]
                  tunnel: [w1536 w1537] -> w1533
                  frame False {
                  }
                  frame True {
                    n718 = Unbundle By Name(w1542) -> ("Ref X"=w1541:refnum<vi>, "Ref Y"=w1540:refnum<vi>)
                    n719 = property class="DigNum (strict)"(reference=w1541, error in=w1539) -> (error out=w1538:errorcluster, "Value"=w1544:dbl)  [unwired: 1 out]
                    n720 = property class="DigNum (strict)"(reference=w1540, error in=w1538) -> (error out=w1537:errorcluster, "Value"=w1543:dbl)  [unwired: 1 out]
                    n721 = property on="Position 1" class="DigNum (strict)"("Value"=w1544) -> ()  [unwired: 2 in, 2 out]
                    n722 = property on="Position 2" class="DigNum (strict)"("Value"=w1543) -> ()  [unwired: 2 in, 2 out]
                  }
                }
              }
              frame #4 {
                n723 = property on="Right" class="Bool (strict)"("DisabledEnum"=w1545) -> ()  [unwired: 2 in, 2 out]
                n724 = property on="Up" class="Bool (strict)"("DisabledEnum"=w1545) -> ()  [unwired: 2 in, 2 out]
                n725 = property on="Left" class="Bool (strict)"("DisabledEnum"=w1545) -> ()  [unwired: 2 in, 2 out]
                n726 = property on="Down" class="Bool (strict)"("DisabledEnum"=w1545) -> ()  [unwired: 2 in, 2 out]
                n727 = property on="StepSize" class="DigNum (strict)"("DisabledEnum"=w1545) -> ()  [unwired: 2 in, 2 out]
              }
            }
            n728 = call-poly <userlib>:"Filter 1D Array__ogtk.vi"("items to filter"=w1519, "array"=w1520) -> ("filtered item indices"=w1518:i32[])  [unwired: 4 in, 1 out]
            n729 = Index Array(array=w1518) -> (element=w1513:i32)  [unwired: 1 in]
            n730 = Unbundle By Name(w1521) -> ("active axis refs 2"=w1517:T11, "active ccd"=w1512:i32)
            n731 = Index Array(array=w1517, index=w1513) -> (element=w1516:cluster{"Ref X":refnum<vi>, "Ref Y":refnum<vi>})
            n732 = call <vilib>:"Add State(s) to Queue__jki_lib_state_machine.vi"("State(s) in (\"\")"=w1525) -> ("States Out"=w1524:string)  [unwired: 14 in]
            n733 = local read "Mean Centroid X"() -> (w1522:dbl[][])
            n734 = Bundle By Name(cluster=w1521, "Mean Centroid X"=w1522, "Mean Centroid Y"=w1522) -> (w1523:T37)
          }
          frame "---------------Statistics--------------" {
            # "Template Separator\n(You can make a copy of, or modify, this frame)"
            n735 = call <vilib>:"Add State(s) to Queue__jki_lib_state_machine.vi"("State(s) in (\"\")"=w1549) -> ("States Out"=w1548:string)  [unwired: 14 in]
          }
          frame "Save Stats" {
            # "Your code here.\n(You can make a copy of, or modify, this frame)"
            n736 = property on="CCD 1" class="XYGraph (strict)"() -> ("Value"=w1560:cluster{timestamp[], dbl[]}[])  [unwired: 2 in, 2 out]
            n737 = property on="CCD 2" class="XYGraph (strict)"() -> ("Value"=w1559:cluster{timestamp[], dbl[]}[])  [unwired: 2 in, 2 out]
            n738 = property on="CCD 3" class="XYGraph (strict)"() -> ("Value"=w1558:cluster{timestamp[], dbl[]}[])  [unwired: 2 in, 2 out]
            n739 = property on="CCD 4" class="XYGraph (strict)"() -> ("Value"=w1557:cluster{timestamp[], dbl[]}[])  [unwired: 2 in, 2 out]
            n740 = property on="CCD 5" class="XYGraph (strict)"() -> ("Value"=w1556:cluster{timestamp[], dbl[]}[])  [unwired: 2 in, 2 out]
            n741 = property on="CCD 6" class="XYGraph (strict)"() -> ("Value"=w1555:cluster{timestamp[], dbl[]}[])  [unwired: 2 in, 2 out]
            n742 = property on="CCD 7" class="XYGraph (strict)"() -> ("Value"=w1554:cluster{timestamp[], dbl[]}[])  [unwired: 2 in, 2 out]
            n743 = property on="CCD 8" class="XYGraph (strict)"() -> ("Value"=w1553:cluster{timestamp[], dbl[]}[])  [unwired: 2 in, 2 out]
            n744 = Build Array(w1560, w1559, w1558, w1557, w1556, w1555, w1554, w1553) -> (w1552:cluster{timestamp[], dbl[]}[][])
            n745 = disable-structure shown="Disabled" {
              disable-tunnel: w1564 -> [w1568 _]
              disable-tunnel: [w1567 _] -> w1563
              disable-tunnel: w1552 -> [w1566 _]
              disable-tunnel: w1551 -> [w1565 _]
              frame Disabled {
                n746 = for {
                  tunnel: w1566 -> [w1571] mode=indexing
                  tunnel: w1565 -> [w1570] mode=indexing
                  n747 = Empty String/Path?(string/path=w1570) -> (empty?=w1569:bool)
                  n748 = case shown="False" w1569 {
                    tunnel: w1571 -> [w1577 _]
                    tunnel: w1570 -> [w1575 _]
                    frame False {
                      n749 = Index Array(array=w1577, index #1=0 ("index"), index #2=1 ("index"), index #3=2 ("index"), index #4=3 ("index")) -> (element #1=w1612:cluster{timestamp[], dbl[]}, element #2=w1606:cluster{timestamp[], dbl[]}, element #3=w1605:cluster{timestamp[], dbl[]}, element #4=w1604:cluster{timestamp[], dbl[]})  [unwired: 1 in, 1 out]
                      n750 = Concatenate Strings(w1575, ".dat" ("string")) -> (w1573:string)
                      n751 = Unbundle(w1612) -> (w1611:timestamp[], w1589:dbl[])
                      n752 = Unbundle(w1606) -> (w1580:dbl[])  [unwired: 1 out]
                      n753 = Unbundle(w1605) -> (w1579:dbl[])  [unwired: 1 out]
                      n754 = Unbundle(w1604) -> (w1578:dbl[])  [unwired: 1 out]
                      n755 = Build Path(base path="save path", name or relative path=w1573) -> (appended path=w1572:path)
                      n756 = for {
                        tunnel: w1611 -> [w1614] mode=indexing
                        tunnel: [w1613] -> w1587 mode=indexing
                        n757 = Format Date/Time String(time format string (%c)="%Y%m%d%H%M%S", seconds (now)=w1614) -> (date/time string=w1613:string)  [unwired: 1 in]
                      }
                      n758 = Array Size(array=w1589) -> (size(s)=w1590:i32)
                      n759 = Number To Fractional String(number=w1589) -> (F-format string=w1586:string[])  [unwired: 3 in]
                      n760 = Number To Fractional String(number=w1580) -> (F-format string=w1583:string[])  [unwired: 3 in]
                      n761 = Number To Fractional String(number=w1579) -> (F-format string=w1582:string[])  [unwired: 3 in]
                      n762 = Number To Fractional String(number=w1578) -> (F-format string=w1581:string[])  [unwired: 3 in]
                      n763 = Initialize Array("", w1590, 5 ("dimension size")) -> (w1588:string[][])
                      n764 = Insert Into Array(array=w1588, index (col)=0 ("disabled index (col)"), new element=w1587) -> (w1598:string[][])  [unwired: 1 in]
                      n765 = Insert Into Array(array=w1598, index (col)=1 ("disabled index (col)"), new element=w1586) -> (w1597:string[][])  [unwired: 1 in]
                      n766 = Insert Into Array(array=w1597, index (col)=2 ("disabled index (col)"), new element=w1583) -> (w1601:string[][])  [unwired: 1 in]
                      n767 = Insert Into Array(array=w1601, index (col)=3 ("disabled index (col)"), new element=w1582) -> (w1602:string[][])  [unwired: 1 in]
                      n768 = Insert Into Array(array=w1602, index (col)=4 ("disabled index (col)"), new element=w1581) -> (w1603:string[][])  [unwired: 1 in]
                      n769 = Insert Into Array(array=w1603, index (row)=0, new element=string[] ["time", "Centroid X", "Centroid Y", "Motor Axis 1", "Motor Axis 2"] ("new element/subarray 2")) -> (w1585:string[][])  [unwired: 1 in]
                      n770 = call-poly <vilib>:"Write To Spreadsheet File.vi"("2D data"=w1585, "file path (dialog if empty)"=w1572) -> ()  [unwired: 6 in, 1 out]
                    }
                    frame True {
                    }
                  }
                }
                n771 = call <vilib>:"Add State(s) to Queue__jki_lib_state_machine.vi"("State(s) in (\"\")"=w1568) -> ("States Out"=w1567:string)  [unwired: 14 in]
              }
              frame Enabled {
              }
            }
            n772 = property on="Save Stats" class="Bool (strict)"("Value"=FALSE ("Save Stats")) -> ()  [unwired: 2 in, 2 out]
          }
          frame "tdms" {
            w1625 = 21600.0 ("new tdms")
            # "Your code here.\n(You can make a copy of, or modify, this frame)"
            n773 = Unbundle By Name(w1634) -> ("active cams"=w1618:string[], "Data Value Reference out"=w1633:refnum<k34>, "Offset X"=w1632:dbl[][], "Offset Y"=w1631:dbl[][], "active axis refs 2"=w1630:T11)
            n774 = for {
              tunnel: w1632 -> [w1681]
              tunnel: w1631 -> [w1680]
              tunnel: w1618 -> [w1644] mode=indexing
              tunnel: w1633 -> [w1645]
              tunnel: w1630 -> [w1666]
              tunnel: w1636 -> [w1650]
              tunnel: [w1648] -> w1635
              i -> [w1667]
              n775 = Index Array(array=w1681, index (row)=w1667) -> (element=w1679:dbl[])  [unwired: 1 in]
              n776 = Index Array(array=w1680, index (row)=w1667) -> (element=w1678:dbl[])  [unwired: 1 in]
              n777 = Index Array(array=w1666, index=w1667) -> (element=w1665:cluster{"Ref X":refnum<vi>, "Ref Y":refnum<vi>})
              n778 = Reverse 1D Array(array=w1678) -> (reversed array=w1676:dbl[])
              n779 = Reverse 1D Array(array=w1679) -> (reversed array=w1677:dbl[])
              n780 = Unbundle By Name(w1665) -> ("Ref X"=w1664:refnum<vi>, "Ref Y"=w1663:refnum<vi>)
              n781 = Index Array(array=w1677) -> (element=w1675:dbl)  [unwired: 1 in]
              n782 = Index Array(array=w1676) -> (element=w1674:dbl)  [unwired: 1 in]
              n783 = property class="DigNum (strict)"(reference=w1664, error in=w1650) -> (error out=w1649:errorcluster, "Value"=w1658:dbl)  [unwired: 1 out]
              n784 = Build Array(w1675) -> (w1647:dbl[])
              n785 = Build Array(w1674) -> (w1669:dbl[])
              n786 = Get Date/Time In Seconds() -> (seconds since 1Jan1904=w1646:timestamp)
              n787 = Build Array(w1646) -> (w1642:timestamp[])
              n788 = property class="DigNum (strict)"(reference=w1663, error in=w1649) -> (error out=w1640:errorcluster, "Value"=w1652:dbl)  [unwired: 1 out]
              n789 = Build Array(w1658) -> (w1657:dbl[])
              n790 = TDMS Write(0:w1645, 5:w1644, 7:"time", 9:w1642, 11:w1640) -> (4:w1641:refnum<k34>, 15:w1639:errorcluster)  [unwired: 1 in, 2 out]
              n791 = Build Array(w1652) -> (w1651:dbl[])
              n792 = TDMS Write(0:w1641, 5:w1644, 7:"centroid X", 9:w1647, 11:w1639) -> (4:w1672:refnum<k34>, 6:w1671:string, 15:w1670:errorcluster)  [unwired: 1 in, 1 out]
              n793 = TDMS Write(0:w1672, 5:w1671, 7:"centroid Y", 9:w1669, 11:w1670) -> (4:w1661:refnum<k34>, 6:w1660:string, 15:w1662:errorcluster)  [unwired: 1 in, 1 out]
              n794 = TDMS Write(0:w1661, 5:w1660, 7:"Motor Axis 1", 9:w1657, 11:w1662) -> (4:w1656:refnum<k34>, 6:w1655:string, 15:w1653:errorcluster)  [unwired: 1 in, 1 out]
              n795 = TDMS Write(0:w1656, 5:w1655, 7:"Motor Axis 2", 9:w1651, 11:w1653) -> (15:w1648:errorcluster)  [unwired: 1 in, 3 out]
            }
            n796 = property on="millisecond timer value" class="DigNum (strict)"() -> ("Value"=w1617:u32)  [unwired: 2 in, 2 out]
            n797 = Tick Count (ms)() -> (millisecond timer value=w1616:u32)
            n798 = Unbundle By Name(w1634) -> ()  [unwired: 1 out]
            n799 = Subtract(x=w1616, y=w1617) -> (x-y=w1620:u32)
            n800 = Divide(x=w1620, y=u32 1000) -> (x/y=w1622:dbl)
            n801 = Quotient & Remainder(x=w1622, y=w1625) -> (x-y*floor(x/y)=w1623:dbl)  [unwired: 1 out]
            n802 = Subtract(x=w1625, y=20.0) -> (x-y=w1627:dbl)
            n803 = Greater?(x=w1623, y=w1627) -> (0:w1624:bool)
            n804 = Select(t="newtdms", s=w1624, f="") -> (s? t:f=w1619:string)
            n805 = call <vilib>:"Add State(s) to Queue__jki_lib_state_machine.vi"("State(s) in (\"\")"=w1638, "State(s) at Back (\"\")"=w1619) -> ("States Out"=w1637:string)  [unwired: 13 in]
          }
          frame "Reset History" {
            # "Your code here.\n(You can make a copy of, or modify, this frame)"
            n806 = for {
              N: 1 -> [_]
              shift-right: [w1691] -> w1683
              shift-left: timestamp[][] [] ("Time") -> [w1693]
              n807 = for {
                N: 12 -> [_]
                tunnel: w1693 -> [w1696] mode=indexing
                tunnel: [w1694] -> w1691 mode=indexing
                n808 = Get Date/Time In Seconds() -> (seconds since 1Jan1904=w1695:timestamp)
                n809 = Build Array (concatenate)(w1696, w1695) -> (w1694:timestamp[])
              }
            }
            n810 = local read "Offset X"() -> (w1682:dbl[][])
            n811 = Bundle By Name(cluster=w1687, "Offset X"=w1682, "Offset Y"=w1682, "Time"=w1683, "Motor X"=w1682) -> (w1686:T37)
            n812 = call <vilib>:"Add State(s) to Queue__jki_lib_state_machine.vi"("State(s) in (\"\")"=w1690) -> ("States Out"=w1689:string)  [unwired: 14 in]
          }
          frame "New Category: 2" {
            # "Your code here.\n(You can make a copy of, or modify, this frame)"
            n813 = call <vilib>:"Add State(s) to Queue__jki_lib_state_machine.vi"("State(s) in (\"\")"=w1700) -> ("States Out"=w1699:string)  [unwired: 14 in]
          }
          frame "stats" {
            # "Your code here.\n(You can make a copy of, or modify, this frame)"
            n814 = Unbundle By Name(w1715) -> ("Offset X"=w1713:dbl[][], "Offset Y"=w1712:dbl[][], "Time"=w1711:timestamp[][], "Motor X"=w1710:dbl[][], "Motor Y"=w1709:dbl[][], "Data Value Reference out"=w1705:refnum<k34>)
            n815 = TDMS List Contents(4:w1704, 7:w1705) -> (0:w1701:errorcluster, 2:w1706:string[], 3:w1707:refnum<k34>)  [unwired: 1 in, 1 out]
            n816 = call <vilib>:"ClearError.vi"("error in (no error)"=w1701) -> ("error out"=w1708:errorcluster)
            n817 = for {
              tunnel: w1708 -> [w1760]
              tunnel: [w1746] -> w1703 mode=indexing
              tunnel: [w1745] -> w1702
              tunnel: [w1744] -> _
              tunnel: w1707 -> [w1743]
              tunnel: w1706 -> [w1742] mode=indexing
              w1761 = dbl[] [] ("appended array")
              n818 = TDMS Read(0:w1743, 5:w1742, 7:"time", 11:w1760, 12:timestamp[] [] ("appended array")) -> (4:w1775:refnum<k34>, 6:w1771:string, 10:w1752:timestamp[], 15:w1759:errorcluster)  [unwired: 3 in, 2 out]
              n819 = TDMS Read(0:w1775, 5:w1771, 7:"centroid X", 11:w1759, 12:w1761) -> (4:w1774:refnum<k34>, 6:w1770:string, 10:w1755:dbl[], 15:w1758:errorcluster)  [unwired: 3 in, 2 out]
              n820 = TDMS Read(0:w1774, 5:w1770, 7:"centroid Y", 11:w1758, 12:w1761) -> (4:w1773:refnum<k34>, 6:w1769:string, 10:w1754:dbl[], 15:w1757:errorcluster)  [unwired: 3 in, 2 out]
              n821 = TDMS Read(0:w1773, 5:w1769, 7:"Motor Axis 1", 11:w1757, 12:w1761) -> (4:w1772:refnum<k34>, 6:w1768:string, 10:w1753:dbl[], 15:w1756:errorcluster)  [unwired: 3 in, 2 out]
              n822 = TDMS Read(0:w1772, 5:w1768, 7:"Motor Axis 2", 11:w1756, 12:w1761) -> (4:w1744:refnum<k34>, 10:w1751:dbl[], 15:w1745:errorcluster)  [unwired: 3 in, 3 out]
              n823 = Bundle("appended array"=w1752, "appended array"=w1755) -> (w1750:T39)  [unwired: 1 in]
              n824 = Bundle("appended array"=w1752, "appended array"=w1754) -> (w1749:T39)  [unwired: 1 in]
              n825 = Bundle("appended array"=w1752, "appended array"=w1753) -> (w1748:T39)  [unwired: 1 in]
              n826 = Bundle("appended array"=w1752, "appended array"=w1751) -> (w1747:T39)  [unwired: 1 in]
              n827 = Build Array(w1750, w1749, w1748, w1747) -> (w1746:T40)
            }
            n828 = disable-structure shown="Disabled" {
              disable-tunnel: w1714 -> [w1782 _]
              disable-tunnel: w1713 -> [w1781 _]
              disable-tunnel: w1712 -> [w1780 _]
              disable-tunnel: w1711 -> [w1779 _]
              disable-tunnel: w1710 -> [w1778 _]
              disable-tunnel: w1709 -> [w1777 _]
              disable-tunnel: [w1776 _] -> _
              frame Disabled {
                n829 = for {
                  tunnel: w1782 -> [_] mode=indexing
                  tunnel: w1781 -> [w1792]
                  tunnel: w1780 -> [w1791]
                  tunnel: w1779 -> [w1790]
                  tunnel: w1778 -> [w1786]
                  tunnel: w1777 -> [w1785]
                  tunnel: [w1794] -> w1776 mode=indexing
                  i -> [w1793]
                  n830 = Index Array(array=w1791, index (row)=w1793) -> (element=w1787:dbl[])  [unwired: 1 in]
                  n831 = Index Array(array=w1792, index (row)=w1793) -> (element=w1788:dbl[])  [unwired: 1 in]
                  n832 = Index Array(array=w1786, index (row)=w1793) -> (element=w1784:dbl[])  [unwired: 1 in]
                  n833 = Index Array(array=w1785, index (row)=w1793) -> (element=w1783:dbl[])  [unwired: 1 in]
                  n834 = Index Array(array=w1790, index (row)=w1793) -> (element=w1789:timestamp[])  [unwired: 1 in]
                  n835 = Bundle("Time"=w1789, "Motor X"=w1784) -> (w1797:cluster{"Time":timestamp[], "Motor X":dbl[]})  [unwired: 1 in]
                  n836 = Bundle("Time"=w1789, "Motor Y"=w1783) -> (w1798:cluster{"Time":timestamp[], "Motor Y":dbl[]})  [unwired: 1 in]
                  n837 = Bundle("Time"=w1789, "Offset X"=w1788) -> (w1796:cluster{"Time":timestamp[], "Offset X":dbl[]})  [unwired: 1 in]
                  n838 = Bundle("Time"=w1789, "Offset Y"=w1787) -> (w1795:cluster{"Time":timestamp[], "Offset Y":dbl[]})  [unwired: 1 in]
                  n839 = Build Array(w1795, w1796, w1797, w1798) -> (w1794:cluster{"Time":timestamp[], "Motor Y":dbl[]}[])
                }
              }
              frame Enabled {
              }
            }
            n840 = call <vilib>:"Add State(s) to Queue__jki_lib_state_machine.vi"("State(s) in (\"\")"=w1741) -> ("States Out"=w1740:string)  [unwired: 14 in]
            n841 = Index Array(array=w1703, index (row) #1=0 ("index (row)"), index (row) #2=1 ("index (row)"), index (row) #3=2 ("index (row)"), index (row) #4=3 ("index (row)"), index (row) #5=4 ("index (row)"), index (row) #6=5 ("index (row)"), index (row) #7=6 ("index (row)"), index (row) #8=7 ("index (row)"), index (row) #9=8 ("index (row)"), index (row) #10=9 ("index (row)"), index (row) #11=10 ("index (row)"), index (row) #12=11 ("index (row)")) -> (element #1=→"CCD 1":T40, element #2=→"CCD 2":T40, element #3=→"CCD 3":T40, element #4=→"CCD 4":T40, element #5=→"CCD 5":T40, element #6=→"CCD 6":T40, element #7=→"CCD 7":T40, element #8=→"CCD 8":T40, element #9=→"CCD 9":T40, element #10=→"CCD 10":T40, element #11=→"CCD 11":T40, element #12=→"CCD 12":T40)  [unwired: 12 in]
          }
          frame "newtdms" {
            # "Your code here.\n(You can make a copy of, or modify, this frame)"
            n842 = Unbundle By Name(w1835) -> ("Data Value Reference out"=w1823:refnum<k34>, "active cams"=w1818:string[])
            n843 = TDMS Close(8:w1833, 11:w1823) -> (0:w1817:errorcluster)  [unwired: 1 out]
            n844 = Get Date/Time In Seconds() -> (seconds since 1Jan1904=w1811:timestamp)
            n845 = call <vilib>:"Clear Errors.vi"("error in (no error)"=w1817) -> ("error out"=w1804:errorcluster)  [unwired: 5 in, 1 out]
            n846 = Format Date/Time String(time format string (%c)="%Y%m%d", seconds (now)=w1811) -> (date/time string=w1812:string)  [unwired: 1 in]
            n847 = Format Date/Time String(time format string (%c)="%Y%m%d%H%M", seconds (now)=w1811) -> (date/time string=w1809:string)  [unwired: 1 in]
            n848 = property on="new tdms" class="Bool (strict)"("Value"=FALSE ("new tdms")) -> ()  [unwired: 2 in, 2 out]
            n849 = Get Date/Time In Seconds() -> (seconds since 1Jan1904=w1832:timestamp)
            n850 = Format Date/Time String(time format string (%c)="%Y%m%d%H%M", seconds (now)=w1832) -> (date/time string=w1824:string)  [unwired: 1 in]
            n851 = Build Path(base path=w1805, name or relative path=w1812) -> (appended path=w1813:path)
            n852 = Concatenate Strings(w1824, "Beampointingbooster_PICO.tdms" ("string")) -> (w1830:string)
            n853 = String To Path(string=w1830) -> ()  [unwired: 1 out]
            n854 = Concatenate Strings(w1809, "Beampointing_heater.tdms" ("string")) -> (w1807:string)
            n855 = String To Path(string=w1807) -> (path=w1802:path)
            n856 = call <vilib>:"Check if File or Folder Exists.vi"("error in (no error)"=w1804, "path"=w1813) -> ("error out"=w1816:errorcluster, "file or folder exists?"=w1814:bool, "dup path"=w1815:path)  [unwired: 7 in]
            n857 = case shown="False" w1814 {
              tunnel: w1815 -> [w1841 w1843]
              tunnel: [w1840 w1843] -> w1801
              tunnel: w1816 -> [w1839 w1842]
              tunnel: [w1838 w1842] -> w1803
              frame False {
                n858 = Create Folder(path (use dialog)=w1841, error in=w1839) -> (created path=w1840:path, error out=w1838:errorcluster)  [unwired: 1 in, 1 out]
              }
              frame True {
              }
            }
            n859 = call <vilib>:"Add State(s) to Queue__jki_lib_state_machine.vi"("State(s) in (\"\")"=w1837) -> ("States Out"=w1836:string)  [unwired: 14 in]
            n860 = Build Path(base path=w1801, name or relative path=w1802) -> (appended path=w1825:path)
            n861 = TDMS Open(6:FALSE ("disable buffering (T)"), 7:enum16{"1.0", "2.0"}."2.0" ("file format version (2.0)"), 8:w1803, 10:T17."create or replace" ("operation"), 11:w1825) -> (0:w1821:errorcluster, 3:w1820:refnum<k34>)  [unwired: 2 in]
            n862 = call "TDMSbuffersize.vi"("error in (no error)"=w1821, "group names"=w1818, "Data Value Reference in"=w1820) -> ("error out"=w1800:errorcluster, "Data Value Reference out"=w1819:refnum<k34>)  [unwired: 7 in]
            n863 = Bundle By Name(cluster=w1835, "Data Value Reference out"=w1819) -> (w1834:T37)
            n864 = call <vilib>:"Clear Errors.vi"("error in (no error)"=w1800) -> ("error out"=w1799:errorcluster)  [unwired: 5 in, 1 out]
          }
          frame "Center" {
            # "Your code here.\n(You can make a copy of, or modify, this frame)"
            n865 = control-ref of="image::1"() -> (w1858:refnum<vi>)
            n866 = control-ref of="image::2"() -> (w1857:refnum<vi>)
            n867 = control-ref of="image::3"() -> (w1856:refnum<vi>)
            n868 = control-ref of="image::4"() -> (w1855:refnum<vi>)
            n869 = control-ref of="image::5"() -> (w1854:refnum<vi>)
            n870 = control-ref of="image::6"() -> (w1853:refnum<vi>)
            n871 = control-ref of="image::7"() -> (w1852:refnum<vi>)
            n872 = control-ref of="image::8"() -> (w1851:refnum<vi>)
            n873 = control-ref of="image::9"() -> (w1850:refnum<vi>)
            n874 = control-ref of="image::10"() -> (w1849:refnum<vi>)
            n875 = control-ref of="image::11"() -> (w1848:refnum<vi>)
            n876 = control-ref of="image::12"() -> (w1847:refnum<vi>)
            n877 = for {
              tunnel: [w1867] -> w1846 mode=indexing
              tunnel: w1845 -> [w1866] mode=indexing
              n878 = Unbundle By Name(w1866) -> ("Target.X::12"=w1865:refnum<vi>, "Target.Y::12"=w1864:refnum<vi>)
              n879 = property class="DigNum (strict)"(reference=w1865) -> ("Value"=w1868:dbl)  [unwired: 1 in, 2 out]
              n880 = property class="DigNum (strict)"(reference=w1864) -> ("Value"=w1869:dbl)  [unwired: 1 in, 2 out]
              n881 = Bundle("Value"=w1868, "Value"=w1869) -> (w1867:cluster{"Value":dbl, "Value":dbl})  [unwired: 1 in]
            }
            n882 = call <vilib>:"Add State(s) to Queue__jki_lib_state_machine.vi"("State(s) in (\"\")"=w1863) -> ("States Out"=w1862:string)  [unwired: 14 in]
            n883 = Build Array(w1858, w1857, w1856, w1855, w1854, w1853, w1852, w1851, w1850, w1849, w1848, w1847) -> (w1859:refnum<vi>[])
            n884 = for {
              tunnel: w1859 -> [w1871] mode=indexing
              tunnel: w1846 -> [w1870] mode=indexing
              n885 = property class="ImageControl"(reference=w1871, "Image Center Position"=w1870) -> ()  [unwired: 1 in, 2 out]
            }
            n886 = property on="Center" class="Bool (strict)"("Value"=FALSE ("Center")) -> ()  [unwired: 2 in, 2 out]
          }
          frame "ImgToAvg" {
            n887 = Decimal String To Number(string=w1881) -> (number=w1878:i32)  [unwired: 2 in, 1 out]
            n888 = Bundle By Name(cluster=w1880, "img to avg"=w1878) -> (w1879:T37)
            n889 = call <vilib>:"Build State String with Arguments__jki_lib_state_machine.vi"("Arguments (\"\")"="T" ("Arguments (\"\")"), "State"=" Device Ini") -> ("State with Arguments"=w1872:string)  [unwired: 4 in]
            n890 = call <vilib>:"Add State(s) to Queue__jki_lib_state_machine.vi"("State(s) in Front (\"\")"=w1872, "State(s) in (\"\")"=w1877) -> ("States Out"=w1876:string)  [unwired: 13 in]
          }
          frame "history" {
            # "Your code here.\n(You can make a copy of, or modify, this frame)"
            n891 = Unbundle By Name(w1891) -> ("Offset X"=w1897:dbl[][], "Offset Y"=w1896:dbl[][], "Mean Centroid X"=w1895:dbl[][], "Mean Centroid Y"=w1894:dbl[][], "Motor X"=w1893:dbl[][], "Motor Y"=w1892:dbl[][], "Time"=w1883:timestamp[][])
            n892 = for {
              tunnel: w1897 -> [w1915] mode=indexing
              tunnel: w1896 -> [w1913] mode=indexing
              tunnel: w1895 -> [w1912] mode=indexing
              tunnel: w1894 -> [w1911] mode=indexing
              tunnel: w1893 -> [w1910] mode=indexing
              tunnel: w1892 -> [w1909] mode=indexing
              tunnel: [w1914] -> w1889 mode=indexing
              tunnel: [w1908] -> w1888 mode=indexing
              tunnel: [w1904] -> w1887 mode=indexing
              tunnel: [w1907] -> w1886 mode=indexing
              tunnel: [w1906] -> w1885 mode=indexing
              tunnel: [w1905] -> w1884 mode=indexing
              tunnel: w1883 -> [w1903] mode=indexing
              tunnel: [w1901] -> w1882 mode=indexing
              w1902 = 0
              n893 = Delete From Array(array=w1910, index=w1902) -> (array with subset deleted=w1906:dbl[])  [unwired: 1 in, 1 out]
              n894 = Delete From Array(array=w1909, index=w1902) -> (array with subset deleted=w1905:dbl[])  [unwired: 1 in, 1 out]
              n895 = Delete From Array(array=w1903, index=w1902) -> (array with subset deleted=w1901:timestamp[])  [unwired: 1 in, 1 out]
              n896 = Delete From Array(array=w1912, index=w1902) -> (array with subset deleted=w1904:dbl[])  [unwired: 1 in, 1 out]
              n897 = Delete From Array(array=w1911, index=w1902) -> (array with subset deleted=w1907:dbl[])  [unwired: 1 in, 1 out]
              n898 = Delete From Array(array=w1913, index=w1902) -> (array with subset deleted=w1908:dbl[])  [unwired: 1 in, 1 out]
              n899 = Delete From Array(array=w1915, index=w1902) -> (array with subset deleted=w1914:dbl[])  [unwired: 1 in, 1 out]
            }
            n900 = call <vilib>:"Add State(s) to Queue__jki_lib_state_machine.vi"("State(s) in (\"\")"=w1900) -> ("States Out"=w1899:string)  [unwired: 14 in]
            n901 = Bundle By Name(cluster=w1891, "Offset X"=w1889, "Offset Y"=w1888, "Mean Centroid X"=w1887, "Mean Centroid Y"=w1886, "Motor X"=w1885, "Motor Y"=w1884, "Time"=w1882) -> (w1890:T37)
          }
        }
        n902 = property on="Box" class="Arr (strict)"() -> ("Value"=w139:T6)  [unwired: 2 in, 2 out]
        n903 = for {
          tunnel: w141 -> [w173]
          tunnel: w140 -> [w174]
          tunnel: w137 -> [w154] mode=indexing
          tunnel: w139 -> [w170] mode=indexing
          tunnel: "ljloj" ("overlay name") -> [w158]
          i -> [w160]
          n904 = call-poly <userlib>:"Filter 1D Array__ogtk.vi"("items to filter"=w154, "array"=w174) -> ("filtered item indices"=w175:i32[])  [unwired: 4 in, 1 out]
          n905 = Index Array(array=w175) -> (element=w171:i32)  [unwired: 1 in]
          n906 = Index Array(array=w173, index=w171) -> (element=w172:T31)
          n907 = Unbundle By Name(w172) -> ("Target.X::12"=w177:refnum<vi>, "Target.Y::12"=w176:refnum<vi>)
          n908 = property class="DigNum (strict)"(reference=w177) -> ("Value"=w167:dbl)  [unwired: 1 in, 2 out]
          n909 = property class="DigNum (strict)"(reference=w176) -> ("Value"=w166:dbl)  [unwired: 1 in, 2 out]
          n910 = Bundle By Name(cluster=T14 {"Draw"=TRUE, "Target"={"x"=20.0, "y"=20.0}, "Size"={"x"=20.0, "y"=20.0}, "Angle"=1250067.0, "Color"=1250067, "Thickness"=20, "CrosshairLabel"=""} ("Crosshair"), "Draw"=TRUE, "Target.x"=w167, "Target.y"=w166, "Size"=cluster{"xhair size":dbl, "xhair size 2":dbl} {"xhair size"=25.0, "xhair size 2"=25.0} ("size"), "Color"=u32 16774656, "Angle"=0.0) -> (w162:T14)
          n911 = call "draw crosshair imaq.vi"("overlay name"="donotrename", "Crosshair"=w162, "Bounding Rectangle"=T15 {"Left"=0, "Top"=0, "Right"=0, "Bottom"=0}, "image in"=w154) -> ("error out"=→"error out":errorcluster, "image out"=w153:T9)  [unwired: 6 in]
          n912 = call "draw box imaq.vi"("Color"=u32 1244928, "Rectangle"=w170, "image in"=w153) -> ("error out"=→"error out 3":errorcluster)  [unwired: 7 in, 1 out]
          n913 = Number To Decimal String(number=w160) -> (decimal integer string=w159:string)  [unwired: 1 in]
          n914 = Concatenate Strings(w159, w158) -> ()  [unwired: 1 out]
        }
      }
      n915 = call "supergui create stop queue.vi"() -> ("STOP Queue out"=w32:refnum<queue>)  [unwired: 11 in]
      n916 = control-ref of="This Application"() -> (w125:refnum<vi>)
      n917 = control-ref of="This VI"() -> (w129:refnum<vi>)
      n918 = Current VI's Menubar() -> (w128:refnum<k9>)
      n919 = call "GUI_Master_subvi_reentrant_queues.vi"("STOP Queue in"=w32, "This Application"=w125, "error in (no error)"=w126, "tcp data event"=w124, "Caller menu reference"=w128, "Caller VI ref"=w129) -> ("error out"=→"error IO 2":errorcluster)  [unwired: 5 in]
      n920 = Unbundle By Name(w70) -> ("Data Value Reference out"=w69:refnum<k34>)
      n921 = for {
        tunnel: w99 -> [w133] mode=indexing
        tunnel: w98 -> [w132]
        tunnel: [w131] -> w68
        n922 = call "IMAQ Dispose"("Image"=w133, "error in (no error)"=w132) -> ("error out"=w131:errorcluster)  [unwired: 4 in]
      }
      n923 = TDMS Close(8:w68, 11:w69) -> (0:w34:errorcluster)  [unwired: 1 out]
      n924 = Release Queue(queue=w32, error in (no error)=w34) -> (error out=→"error out 2":errorcluster)  [unwired: 1 in, 2 out]
      "Names" <- w39
    }
  }
